vi "myRIO_BRig_RT_v0,80__PortC.vi"() -> ()   [LabVIEW 2014]
uses:
  myRIO_BRig_RT__Case_Exp_stateList.ctl
  myRIO_BRig_RT__Case_NonExp_stateList.ctl
  <vilib>/Platform/TimedLoop/XDataNode/timing_clust.ctl
  <vilib>/Platform/TimedLoop/XDataNode/nitl_modes.ctl
  <vilib>/Platform/TimedLoop/XDataNode/wakeup.ctl
  <vilib>/WebDAVClient/Advanced/SessionHandle.ctl
  <vilib>/myRIO/Common/Instrument Driver Framework/myRIO v1.0/UART/vis/myRIO v1.0 Close UART.vi
  <vilib>/FPGAPlugInAG/myRIO-1900/niLvFpga_Open_myRIO-1900.vi
  <vilib>/rvi/interface/common/dynamic/niFpgaDynamicAddResources.vi
  <vilib>/Utility/error.llb/Error Cluster From Error Code.vi
  <vilib>/rvi/errors/niLvFpgaAdjustHostInterfaceError.vi
  <vilib>/FPGAPlugInAG/Dynamic/niLvFpga_Close_Dynamic.vi
  <vilib>/myRIO/Common/Instrument Driver Framework/Utilities/vis/FPGA Ref Manager.vi
  <vilib>/myRIO/Common/Instrument Driver Framework/myRIO v1.0/myRIO v1.0 Reset FPGA.vi
  <vilib>/myRIO/Common/Instrument Driver Framework/myRIO v1.0/IRQ/vis/myRIO v1.0 IRQ Info FGV.vi
  <vilib>/myRIO/Common/Instrument Driver Framework/myRIO v1.0/IRQ/vis/myRIO v1.0 Timer IRQ Info FGV.vi
  <vilib>/myRIO/Common/Instrument Driver Framework/myRIO v1.0/IRQ/vis/myRIO v1.0 ISR Agent.vi
  <vilib>/rvi/interface/nirviOpenFPGA/nirviOpenFPGA.xnode
  myRIO_BRig_FPGA_v3,71__PortC__build.lvbitx
  myRIO_BRig_FPGA_v3,71__PortC.vi
  <vilib>/rvi/interface/nirviReadWriteControl/nirviReadWriteControl.xnode
  <vilib>/Platform/TimedLoop/XDataNode/XDataNode.xnode
  <vilib>/rvi/interface/nirviCloseFPGA/nirviCloseFPGA.xnode
  <vilib>/Platform/TimedLoop/XDataNode/XDNodeRunTimeDep.lvlib
  <vilib>/rvi/interface/Simulation/niFpgaSimulationCallBeginRW.vi
  <vilib>/myRIO/Instrument Drivers/Utilities/Utilities.lvlib
  <vilib>/WebDAVClient/NI_WebDAV.lvlib
  NiFpgaLv.dll
panel:
  in  "Tcycle_Cue_LED_max":u16=1000 caption="Max" min=5 max=5000 step=5
  in  "Tcycle_Cue_LED_min":u16=1000 caption="Min" min=5 max=5000 step=5
  in  "Tcycle_CuePenalty_LED":u16=1000 caption="Penalty" min=1 max=10000 step=1
  out "power_l2":dbl
  out "error out 6":errorcluster
  in  "MTrig_Laser_Switch":bool
  in  "Cue1Param_AudioLed_Count_NS":u16
  in  "Cue1Param_AudioLed_Count_Switch":u16
  in  "Cue1Param_AudioLed_Probability_NS":u16
  in  "Cue1Param_CueType_NS":u16(slide) max=2 step=1 scale=0.0..2.0
  in  "Cue1Param_AudioLed_Probability_Switch":u16
  in  "Cue1Param_CueType_Switch":u16(slide) max=2 step=1 scale=0.0..2.0
  in  "CueLed_Freq":dbl=10.0
  in  "CueLed_Tpeak":dbl=2.0
  in  "Laser_power_step_l2":dbl
  in  "Laser_power_max_l2":dbl
  in  "Laser_power_min_l2":dbl
  in  "Laser_Tshutter_l2":dbl=2.0
  in  "Laser_Freq_l2":dbl=10.0
  in  "Laser_Tpeak_l2":dbl=2.0
  in  "Laser_duration_l2":u16
  in  "LC_Sel_Count_NS_l2":u16
  in  "LC_Sel_Count_Switch_l2":u16
  in  "LC_Sel_Probability_NS_l2":u16
  in  "LC_Sel_Block_NS_l2":u16(slide) max=2 step=1 scale=0.0..2.0
  in  "LC_Sel_OnOff_NS_l2":bool
  in  "LC_Sel_Probability_Switch_l2":u16
  in  "LC_Sel_Block_Switch_l2":u16(slide) max=2 step=1 scale=0.0..2.0
  in  "LC_Sel_OnOff_Switch_l2":bool
  in  "LC_Sel_Tdelay_NS_l2":u16
  in  "LC_Sel_Tdelay_Switch_l2":u16
  in  "LC_Cue1_Count_NS_l2":u16
  in  "LC_Cue1_Count_Switch_l2":u16
  in  "LC_Cue1_delayOpt_NS_l2":bool
  in  "LC_ENL1_delayOpt_NS_l2":bool
  in  "LC_ENL1_Count_NS_l2":u16
  in  "LC_ENL1_Count_Switch_l2":u16
  in  "LC_Cue1_delayOpt_Switch_l2":bool
  in  "LC_ENL1_delayOpt_Switch_l2":bool
  in  "LC_Cue1_Probability_NS_l2":u16
  in  "LC_Cue1_Block_NS_l2":u16(slide) max=2 step=1 scale=0.0..2.0
  in  "LC_Cue1_OnOff_NS_l2":bool
  in  "LC_Cue1_Probability_Switch_l2":u16
  in  "LC_Cue1_Block_Switch_l2":u16(slide) max=2 step=1 scale=0.0..2.0
  in  "LC_Cue1_OnOff_Switch_l2":bool
  in  "LC_ENL1_Probability_NS_l2":u16 max=100 step=1
  in  "LC_ENL1_Block_NS_l2":u16(slide) max=2 step=1 scale=0.0..2.0
  in  "LC_ENL1_OnOff_NS_l2":bool
  in  "LC_ENL1_Probability_Switch_l2":u16 max=100 step=1
  in  "LC_ENL1_Block_Switch_l2":u16(slide) max=2 step=1 scale=0.0..2.0
  in  "LC_Cue1_Tdelay_NS_l2":u16
  in  "LC_ENL1_Tdelay_NS_l2":u16
  in  "LC_Cue1_Tdelay_Switch_l2":u16
  in  "LC_ENL1_Tdelay_Switch_l2":u16
  in  "LC_ENL1_OnOff_Switch_l2":bool
  in  "LC_Wrong_Probability_l2":u16
  in  "LC_Wrong_Trial_l2":u16(slide) max=2 step=1 scale=0.0..2.0
  in  "LC_Wrong_Block_l2":u16(slide) max=2 step=1 scale=0.0..2.0
  in  "LC_Wrong_OnOff_l2":bool
  in  "LC_Reward_Probability_l2":u16
  in  "LC_Reward_Trial_l2":u16(slide) max=2 step=1 scale=0.0..2.0
  in  "LC_Reward_Block_l2":u16(slide) max=2 step=1 scale=0.0..2.0
  in  "LC_Reward_OnOff_l2":bool
  in  "LC_Wrong_Tdelay_l2":u16
  in  "LC_Reward_Tdelay_l2":u16
  in  "LC_Sel_Count_NS_l1":u16
  in  "LC_Sel_Count_Switch_l1":u16
  in  "LC_Sel_Probability_NS_l1":u16
  in  "LC_Sel_Block_NS_l1":u16(slide) max=2 step=1 scale=0.0..2.0
  in  "LC_Sel_OnOff_NS_l1":bool
  in  "LC_Sel_Probability_Switch_l1":u16
  in  "LC_Sel_Block_Switch_l1":u16(slide) max=2 step=1 scale=0.0..2.0
  in  "LC_Sel_OnOff_Switch_l1":bool
  in  "LC_Sel_Tdelay_NS_l1":u16
  in  "LC_Sel_Tdelay_Switch_l1":u16
  out "I_connect_TCP":bool
  out "error out 5":errorcluster
  in  "get_countPerMS":bool
  in  "count_warmup_R_reset":bool
  in  "count_warmup_L_reset":bool
  out "count_warmup_R":u16
  out "count_warmup_L":u16
  out "SolenoidReward":bool
  in  "SolenoidProbability_L":u16=100 caption="Reward Time [ms]" min=1 max=1000 step=1
  in  "SolenoidProbability_R":u16=100 caption="Reward Time [ms]" min=1 max=1000 step=1
  out "power_l1":dbl caption="LaserPower"
  out "error out 4":errorcluster
  in  "Laser_power_step_l1":dbl
  in  "Laser_power_max_l1":dbl
  in  "Recording":bool
  out "error out 3":errorcluster
  out "error out 2":errorcluster
  in  "Laser_power_min_l1":dbl
  in  "FPGA_count2ms":dbl=159.0
  in  "Laser_Tshutter_l1":dbl=2.0
  in  "Laser_Freq_l1":dbl=10.0
  in  "Laser_Tpeak_l1":dbl=2.0
  in  "Laser_duration_l1":u16
  out "error out":errorcluster
  in  "LC_Cue1_Count_NS_l1":u16
  in  "LC_Cue1_Count_Switch_l1":u16
  in  "LC_Cue1_delayOpt_NS_l1":bool
  in  "LC_ENL1_delayOpt_NS_l1":bool
  in  "LC_ENL1_Count_NS_l1":u16
  in  "LC_ENL1_Count_Switch_l1":u16
  in  "LC_Cue1_delayOpt_Switch_l1":bool
  in  "LC_ENL1_delayOpt_Switch_l1":bool
  in  "Tcycle_Cue_Audio_max":u16=1000 caption="Max" min=5 max=5000 step=5
  in  "Tcycle_Cue_Audio_min":u16=1000 caption="Min" min=5 max=5000 step=5
  in  "SendData":bool
  out "cSpout":enum16{"Left", "Right"}(ring) caption="Left or Right Spout"
  out "A4":u32 caption="LickCounter_Right"
  out "A2":u32 caption="LickCounter_Left"
  in  "LR_wrong_Event":bool
  out "error_initTrial":errorcluster
  out "error_Selection_pre":errorcluster
  out "error_Selection":errorcluster
  out "SelectWrong":bool
  out "SelectReward":bool
  in  "Left(F)_or_Right(T)":bool
  in  "ignoreWrong":bool
  in  "SelectionState":bool
  in  "LR_wrong_Laser":bool
  in  "LR_reward_Laser":bool
  in  "LR_reward_Event":bool
  out "nRewards_Right":u16 caption="# Rewards Total (Right)"
  out "nRewards_Left":u16 caption="# Rewards Total (Left)"
  out "nRewards_cur":u16 caption="# Rewards in Current Block"
  out "TpB_target":u16 caption="Target Trials Per Block"
  out "cState_NonExp":T1 caption="WarmUp State"
  out "iBlock":u16 caption="Current Block"
  out "cState":T2 caption="Experimental State"
  out "iTrial":u16 caption="Current Trial"
  in  "warmupType":u8(slide) max=2 step=1 scale=0.0..2.0
  in  "TestConnection":bool
  in  "warmup":bool caption="WarmUp"
  in  "Data Set Prefix":string="Exp1_TM2"
  out "Connected To Host?":bool
  in  "Host Password":string="sabalab"
  in  "Host UserName":string="Test2"
  in  "sp_RightSpout":u16(slide)=2 max=2 step=1 scale=0.0..2.0
  in  "sp_LeftSpout":u16(slide)=2 max=2 step=1 scale=0.0..2.0
  in  "BUR_max":u16 caption="Count Reward Structure  (0 = off)"
  in  "LC_Wrong_Probability_l1":u16
  in  "LC_Wrong_Trial_l1":u16(slide) max=2 step=1 scale=0.0..2.0
  in  "LC_Wrong_Block_l1":u16(slide) max=2 step=1 scale=0.0..2.0
  in  "LC_Wrong_OnOff_l1":bool
  in  "LC_Reward_Probability_l1":u16
  in  "LC_Reward_Trial_l1":u16(slide) max=2 step=1 scale=0.0..2.0
  in  "LC_Reward_Block_l1":u16(slide) max=2 step=1 scale=0.0..2.0
  in  "LC_Reward_OnOff_l1":bool
  in  "LC_Cue1_Probability_NS_l1":u16
  in  "LC_Cue1_Block_NS_l1":u16(slide) max=2 step=1 scale=0.0..2.0
  in  "LC_Cue1_OnOff_NS_l1":bool
  in  "LC_Cue1_Probability_Switch_l1":u16
  in  "LC_Cue1_Block_Switch_l1":u16(slide) max=2 step=1 scale=0.0..2.0
  in  "LC_Cue1_OnOff_Switch_l1":bool
  in  "LC_ENL1_Probability_NS_l1":u16 max=100 step=1
  in  "LC_ENL1_Block_NS_l1":u16(slide) max=2 step=1 scale=0.0..2.0
  in  "LC_ENL1_OnOff_NS_l1":bool
  in  "LC_ENL1_Probability_Switch_l1":u16 max=100 step=1
  in  "LC_ENL1_Block_Switch_l1":u16(slide) max=2 step=1 scale=0.0..2.0
  in  "Tcycle_Timeout":u16=1000 caption="Timeout Time [ms]" min=10 max=10000 step=1
  in  "Tcycle_Wrong":u16=1000 caption="Wrong Time [ms]" min=10 max=10000 step=1
  in  "Tcycle_Selection":u16=1000 caption="Answer Time [ms]" min=1 max=10000 step=1
  in  "Tcycle_RewardPost":u16=1000 caption="Consumption Time [ms]" min=250 max=10000 step=250
  in  "Tcycle_Reward_L":u16=500 caption="Reward Time [ms]" min=1 max=1000 step=1
  in  "Tcycle_Reward_R":u16=500 caption="Reward Time [ms]" min=1 max=1000 step=1
  in  "TpB_Max_R":u16=4 caption="Max TrialsPerBlock" min=1 max=12 step=1
  in  "TpB_Min_R":u16=4 caption="Min TrialsPerBlock" min=1 max=12 step=1
  in  "TpB_Max_L":u16=4 caption="Max TrialsPerBlock" min=1 max=12 step=1
  in  "TpB_Min_L":u16=4 caption="Min TrialsPerBlock" min=1 max=12 step=1
  in  "BUR_min":u16 caption="Count Reward Structure\n(0 = off)"
  in  "TrialUntilReward":bool caption="Ignore Wrong Selection"
  in  "CueCycles":u16=1 caption="Cue Structure" min=1 max=1 step=1
  in  "MTrig_Laser_Tcycle":u16=10 caption="Time [ms]"
  in  "MTrig_Laser_trig":bool
  in  "MTrig_Audio_trig__R":bool caption="Trigger Audio"
  in  "MTrig_Audio_trig__L":bool caption="Trigger Audio"
  in  "RewCalib_Trig_R":bool caption="Calibrate_R"
  in  "RewCalib_Trig_L":bool caption="Calibrate_L"
  in  "MTrig_Solenoid_Tcycle__R":u16=300 caption="Time [ms]"
  in  "MTrig_Solenoid_Tcycle__L":u16=300 caption="Time [ms]"
  in  "MTrig_Solenoid_trig__R":bool caption="Solenoid"
  in  "MTrig_Solenoid_trig__L":bool caption="Solenoid"
  in  "STOP_abort":bool caption="Stop LabView\n(Stops myRio and FPGA)"
  in  "STOP_endBlock":bool caption="Stop Experiment\n@ End of Block"
  in  "STOP_endTrial":bool caption="Stop Experiment\n@ End of Trial"
  in  "START":bool caption="Start Experiment"
  in  "Tcycle_CuePenalty_Audio":u16=1000 caption="Penalty" min=1 max=10000 step=1
  in  "Audio_Amp__R":u16=100 caption="Amp"
  in  "Audio_Freq__R":u8=5 caption="Freq [kHz]" max=14 step=1
  in  "Audio_Amp__L":u16=100 caption="Amp"
  in  "Audio_Freq__L":u8=5 caption="Freq [kHz]" max=14 step=1
  in  "LC_Wrong_Tdelay_l1":u16
  in  "LC_Cue1_Tdelay_NS_l1":u16
  in  "LC_ENL1_Tdelay_NS_l1":u16
  in  "LC_Reward_Tdelay_l1":u16
  in  "LC_Cue1_Tdelay_Switch_l1":u16
  in  "LC_ENL1_Tdelay_Switch_l1":u16
  in  "LC_ENL1_OnOff_Switch_l1":bool
  in  "Tcycle_ENLPenalty":u16=100 caption="Penalty" min=10 max=10000 step=10
  in  "Tcycle_ENL_max":u16=1000 caption="Max" min=250 max=10000 step=250
  in  "Tcycle_ENL_min":u16=1000 caption="Min" min=250 max=10000 step=250
  # "Communication (Host PC)"
  # "Recording Rig"
  # "Experimental Run"
  # "Current State"
  # "STOP experiment at"
  # "Global Parameters                                                         Trial Parameters"
  # "Left/Right        Give Reward?        Laser Power [V]"
  # "Laser1      Laser2"
  # "FPGA Count per [ms]"
  # "Experiment Task Structure"
  # "Block                   Trial            Target Trials       # Rewards \n                                                            Per Block             Current"
  # "Min            Max            Penalty"
  # "(1) = Switching\n(2) = Two Choice"
  # "WarmUp State"
  # "Lick Counter"
  # "Enforced\nNonLick"
  # "WarmUp"
  # "Left           Right"
  # "Cue then reward (no lick)\n \nLeft                    Right"
  # "# Rewards Total\n                                                                  Left                    Right"
  # "Cue Audio"
  # "Experimental State"
  # "Cue LED"
  # "Selection\n \n\n \nReward\n    Dispense\n    Time\n \n    Dispense\n    Probability\n \n\n    Consumption\n    Time\n\nWrong Choice\n \n \nTimeout Penalty"
  # "Left                  Right"
  # "Manual Control"
  # "Min"
  # "Max"
  # "Solenoid\n \nLeft              Right"
  # "Speaker\n \nLeft                    Right"
  # "Laser 1  |  Laser 2"
  # "Trial Per Block Structure \n               Left                        Right"
  # "Time\n[ms]"
  # "Time\n[ms]"
  # "Time = Cue Min"
  # "Min"
  # "Power = Min"
  # "Max"
  # "Cue1 Control\n                                  Cue Type           LED Probability [%]      Count"
  # "Laser1 Control\n                               On/Off      Block        Probability [%]   Delay [ms]                              Count"
  # "Laser2 Control\n                               On/Off      Block        Probability [%]   Delay [ms]                              Count"
  # "Audio or LED"
  # "Cue 1"
  # "Enforced\nNonLick\n      1"
  # "Enforced\nNonLick\n      1"
  # "from end"
  # "from end"
  # "Switch\nTrial"
  # "Switch\nTrial"
  # "Switch\nTrial"
  # "from start"
  # "from start"
  # "from end"
  # "from end"
  # "NonSwitch\nTrials"
  # "NonSwitch\nTrials"
  # "NonSwitch\nTrials"
  # "from start"
  # "from start"
  # "Cue 1"
  # "Cue 1"
  # "from end"
  # "from end"
  # "Switch\nTrial"
  # "Switch\nTrial"
  # "Cue Audio Parameters"
  # "Cue LED Parameters"
  # "from start"
  # "from start"
  # "Left                  Right"
  # "Frequency\n[Hz]"
  # "Frequency\n[kHz]"
  # "from end"
  # "from end"
  # "NonSwitch\nTrials"
  # "NonSwitch\nTrials"
  # "Timing [ms]\n                    Peak Width"
  # "from start"
  # "from start"
  # "Amp\n(0 - 32,000)"
  # "Selection"
  # "Selection"
  # "from start"
  # "from start"
  # "Switch\nTrial"
  # "Switch\nTrial"
  # "Speaker\nPattern\nDuring Cue"
  # "from start"
  # "from start"
  # "NonSwitch\nTrials"
  # "NonSwitch\nTrials"
  # "Laser1 Parameters"
  # "Laser2 Parameters"
  # "Laser1 Response\n                               On/Off      Block       Trial       Probability [%]   Delay [ms]"
  # "Laser2 Response\n                               On/Off      Block       Trial       Probability [%]   Delay [ms]"
  # "Frequency\n[Hz]"
  # "Frequency\n[Hz]"
  # "Timing [ms]\n Duration     Peak Width   Shutter"
  # "Timing [ms]\n Duration     Peak Width   Shutter"
  # "Selection Reward"
  # "Selection Reward"
  # "Laser Power [V]\nMin          Max              Step"
  # "Laser Power [V]\nMin          Max              Step"
  # "Selection Wrong"
  # "Selection Wrong"
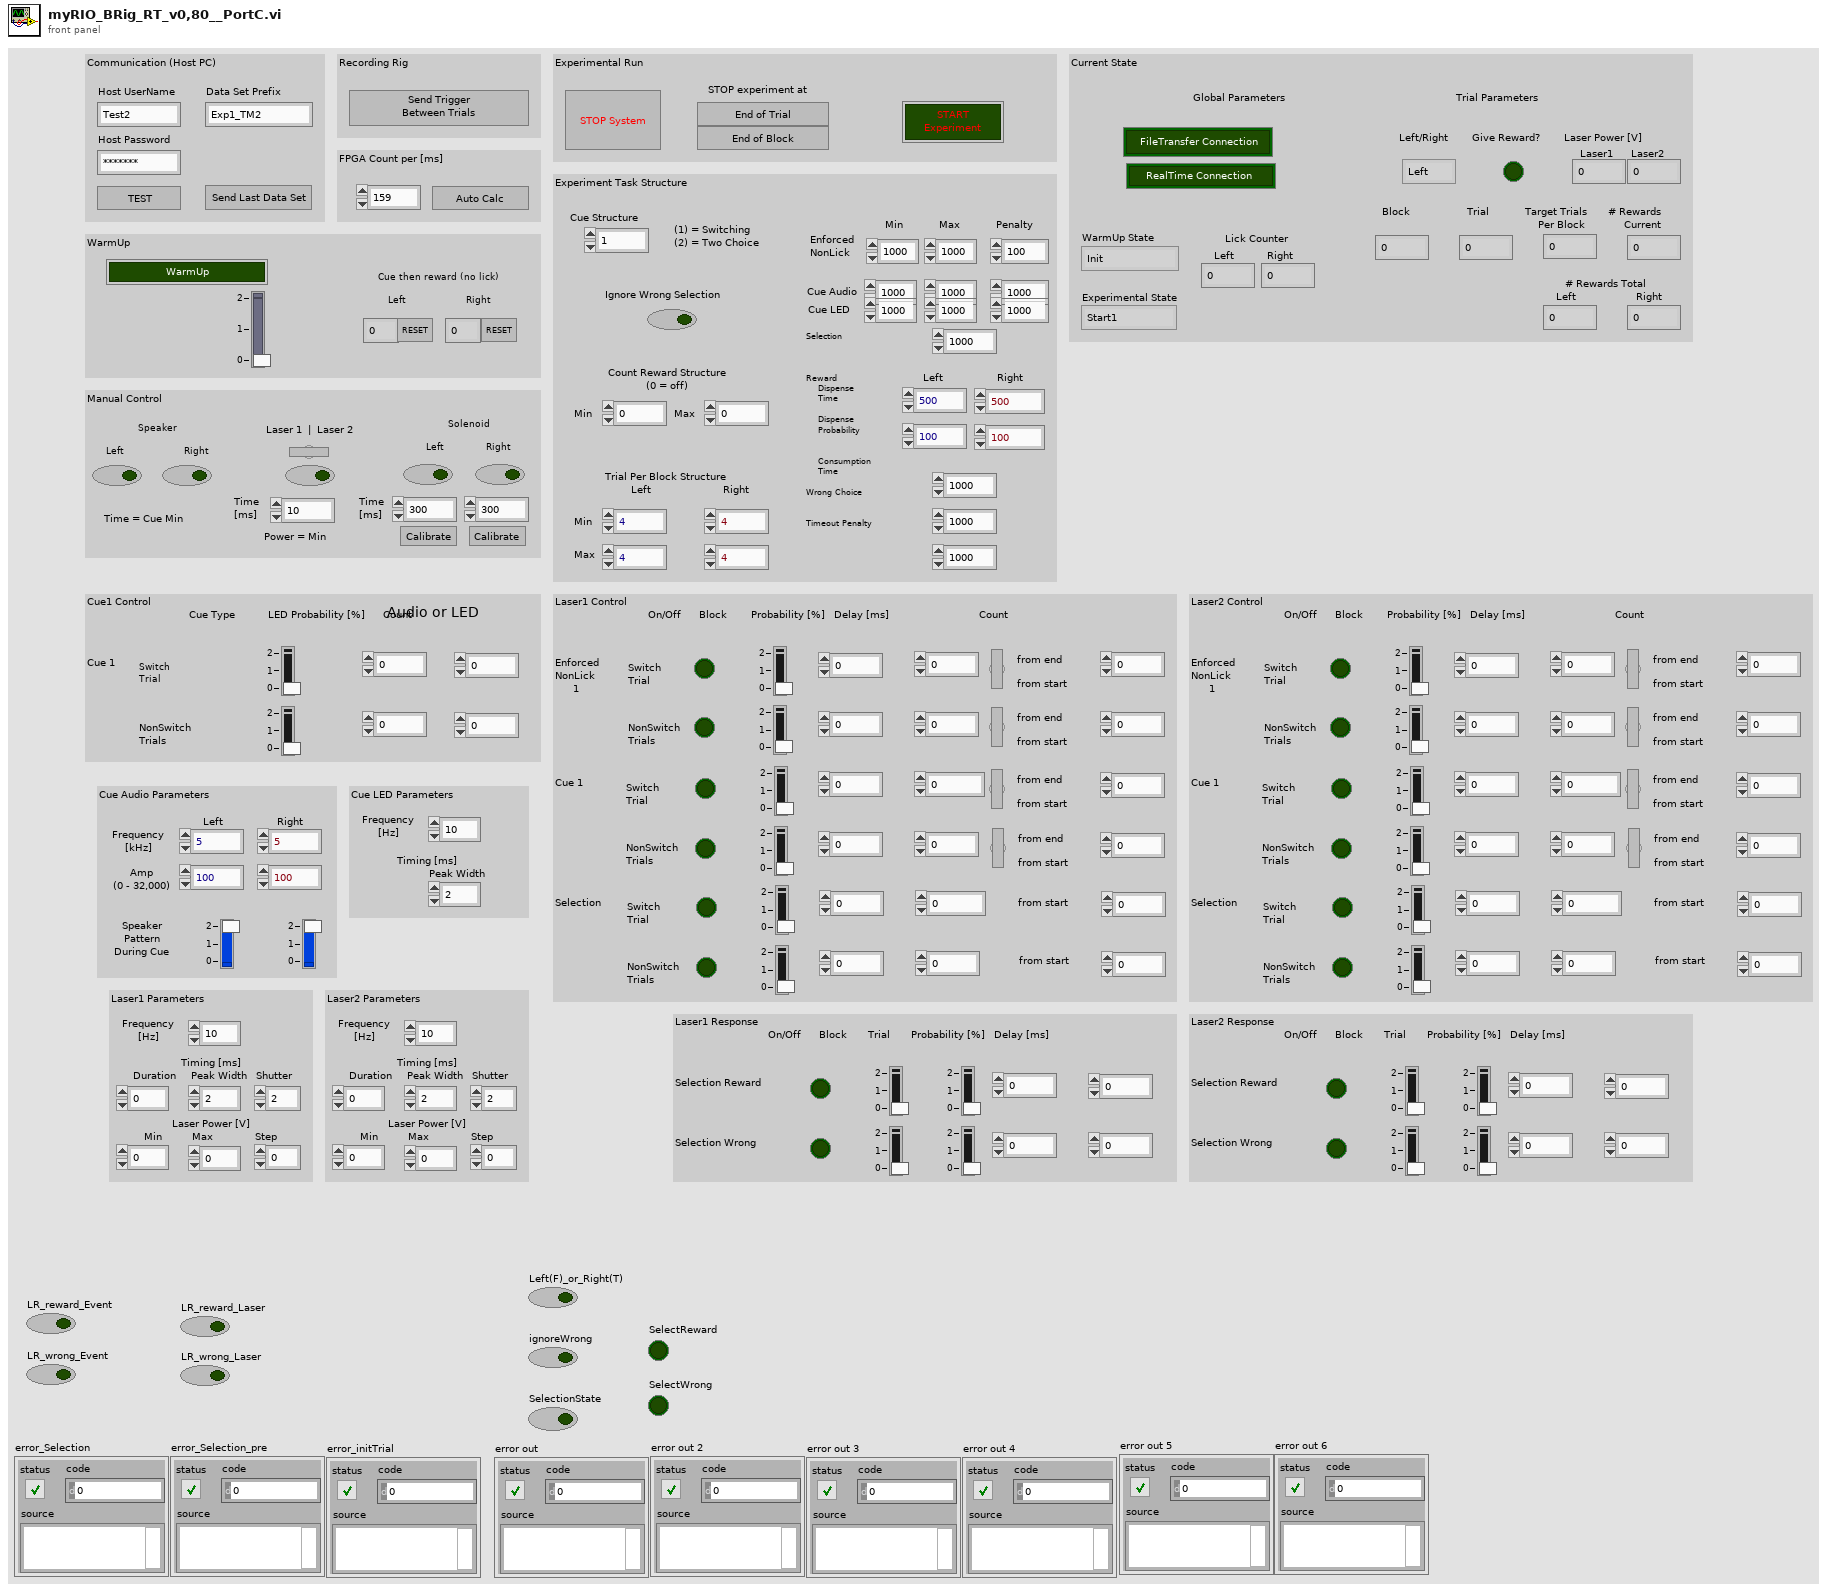
[diagram p1: front panel]
types:
  T1 = typedef "myRIO_BRig_RT__Case_NonExp_stateList.ctl" = enum16{"Init", "UploadSettings_pre", "UploadSettings_Read_dataExp", "UploadSettings_dataExp_1", "UploadSettings_dataExp_2", "UploadSettings_Read_dataLC", "UploadSettings_dataLC_1", "UploadSettings_dataLC_2", "UploadSettings_dataLC_3", "UploadSettings_dataLC_4", "UploadSettings_Read_dataMTrig", "UploadSettings_dataMTrig_1", "UploadSettings_post", "Idle_pre", "IdleEmpty", "IdleEmpty2", "IdleEmpty3", "IdleEmpty4", "Idle", "Idle_2", "Idle_3", "Idle_4", "Idle_5", "Idle_6", "Idle_post", "Cue_pre__pre", "Cue_pre", "Cue", "Cue_LED", "Cue_post", "RewardCalibration_pre", "DispenseWater_pre__pre", "DispenseWater_pre", "DispenseWater", "DispenseWater_post", "TestConnection", "SendData", "Get_FPGA_count_per_ms", "End"}
  T2 = typedef "myRIO_BRig_RT__Case_Exp_stateList.ctl" = enum16{"Start1", "Start2", "Start3", "saveSettings1", "saveSettings2", "saveSettings3", "saveSettings4", "saveSettings_LC_ENL_l1", "saveSettings_LC_ENL_l2", "saveSettings_LC_Cue_l1", "saveSettings_LC_Cue_l2", "saveSettings6_LC_l1_Other", "SaveSettings6_LC_l2_Other", "setSettings_Audio", "setSettings_Laser", "initBlock_pre", "initBlock", "initBlock2", "initBlock_post", "initTrial_pre", "initTrial", "initTrial2", "initTrial3", "initTrial4", "initTrial_LC_ENL1", "initTrial_LC_Cue1", "initTrial_LC_Cue1_2", "initTrial_LC_Sel", "initTrial_post", "ENL1_pre", "ENL1", "ENL1_post", "ENL1Penalty_pre", "ENL1Penalty", "ENL2_pre", "ENL2", "ENL2Penalty_pre", "ENL2Penalty", "Cue1_pre", "Cue1", "Cue1_post", "Cue1Penalty_pre", "Cue1Penalty", "Cue2_pre", "Cue2", "Cue2Penalty_pre", "Cue2Penalty", "Selection_pre", "Selection", "Select_post", "SelectReward_pre", "SelectReward", "SelectRewardPost_pre", "SelectRewardPost", "SelectWrong_pre", "SelectWrong", "SelectWrong_post", "SelectTimeout_pre", "SelectTimeout", "SelectTimeout_post", "endTrial_pre", "endTrial1", "endTrial2", "endTrial3", "endTrial_post", "endBlock_pre", "endBlock", "endBlock_post", "endExp", "commConnect", "commUpload_pre", "commUpload_dataBlock", "commUpload_dataCurrent", "commUpload_dataExp", "commUpload_dataLC", "commUpload_dataTrial", "commUpload_post", "saveData_pre", "saveData_dataBlock", "saveData_dataCurrent", "saveData_dataExp", "saveData_dataLC", "saveData_dataTrial", "saveData_post", "empty_endBlock1", "empty_endBlock2", "empty_endTrial1", "empty_endTrial2", "empty_endTrial3", "empty_endTrial4", "empty_endTrial5", "dummyState", "dummyState_endBlock"}
  T3 = typedef "XDNodeRunTimeDep.lvlib/timing_clust.ctl" = cluster{"Expected End [f-1]":u64, "Actual End [f-1]":u64, "Finished Late? [f-1]":bool, "Expected End [i-1]":u64, "Actual End [i-1]":u64, "Finished Late? [i-1]":bool, "Expected Start [i]":u64, "Actual Start [i]":u64, "Expected Start [f]":u64, "Actual Start [f]":u64, "Source Name":string, "Structure Name":string, "Period":i64, "Deadline":i64, "Offset":i64, "Start":i64, "Priority":i32, "Timeout":i32, "Mode":T4, "Wakeup Reason":T5, "Error":errorcluster, "Source Type":string, "Secondary Source Type":string, "Global End Time":u64, "Global Start Time":u64, "Frame Duration":u64, "Iteration Duration":u64, "Assigned CPU":i32, "I/O Scan Engine Mode":u32}
  T4 = typedef "XDNodeRunTimeDep.lvlib/nitl_modes.ctl" = enum32{"No Change", "Process missed periods, maintain original phase", "Discard missed periods, maintain original phase", "Process missed periods, ignore original phase", "Discard missed periods, ignore original phase"}
  T5 = typedef "XDNodeRunTimeDep.lvlib/wakeup.ctl" = enum32{"Normal", "Aborted", "Asynchronous wakeup", "Timing source error", "Timed loop error", "Timeout"}
  T6 = typedef "NI_WebDAV.lvlib/SessionHandle.ctl" = refnum<k1>
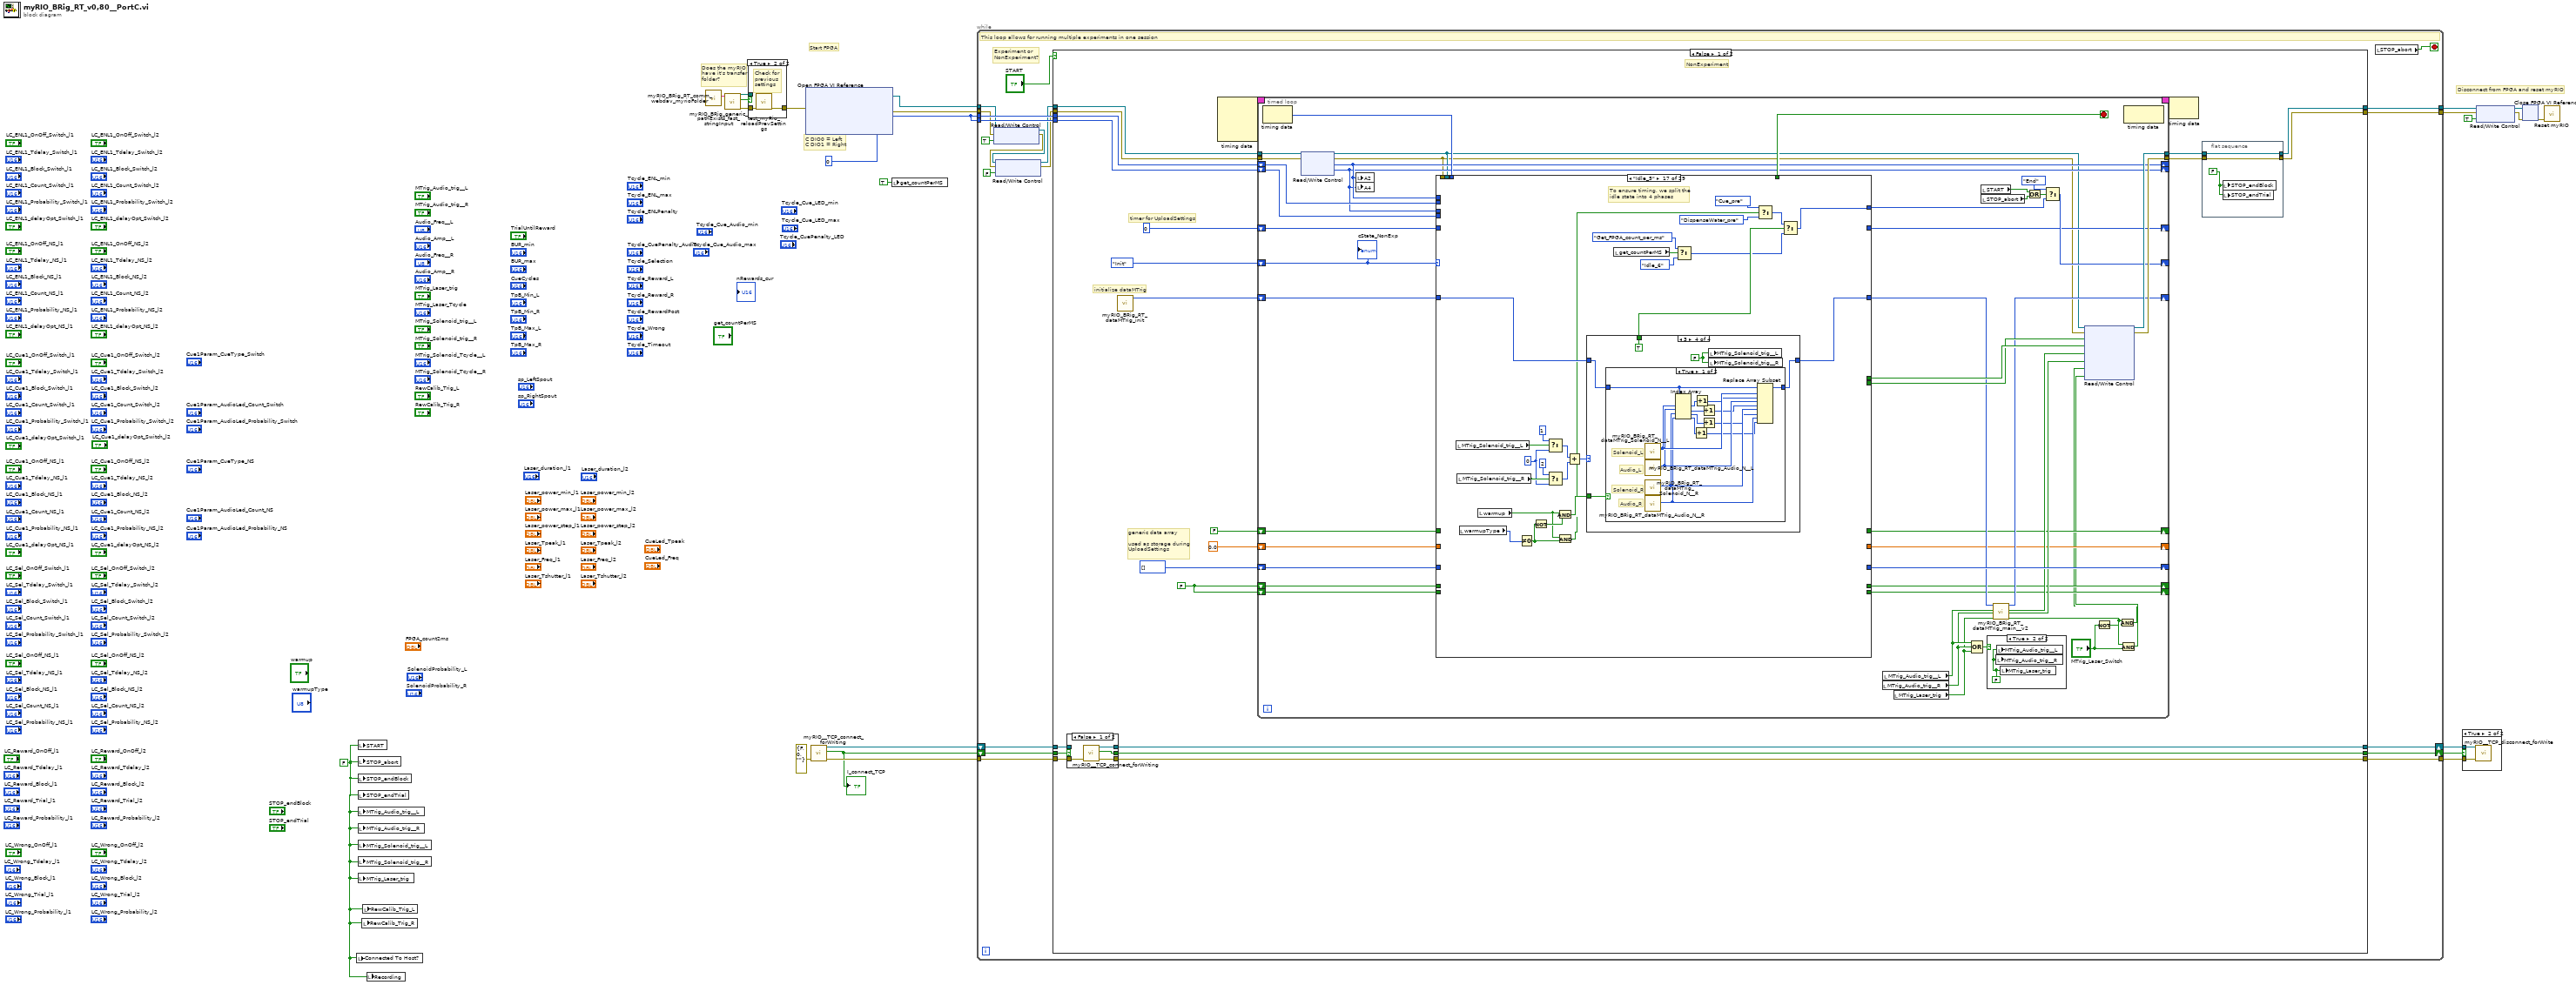
[diagram p0: block diagram]
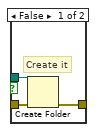
[diagram p3: hidden frame]
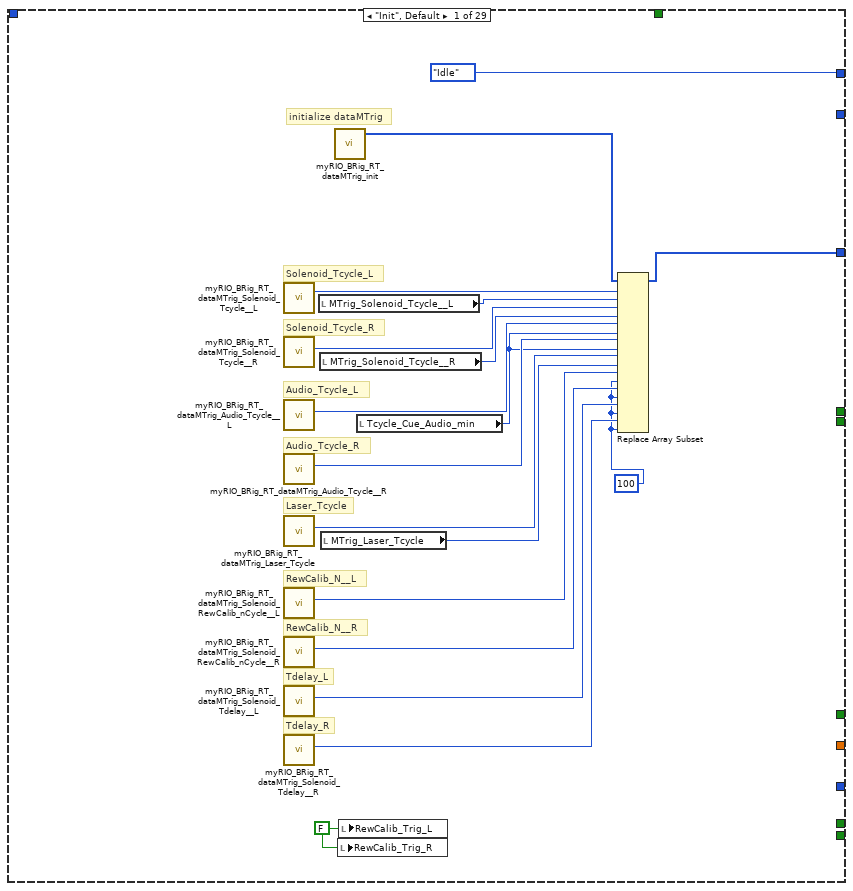
[diagram p6: hidden frame]
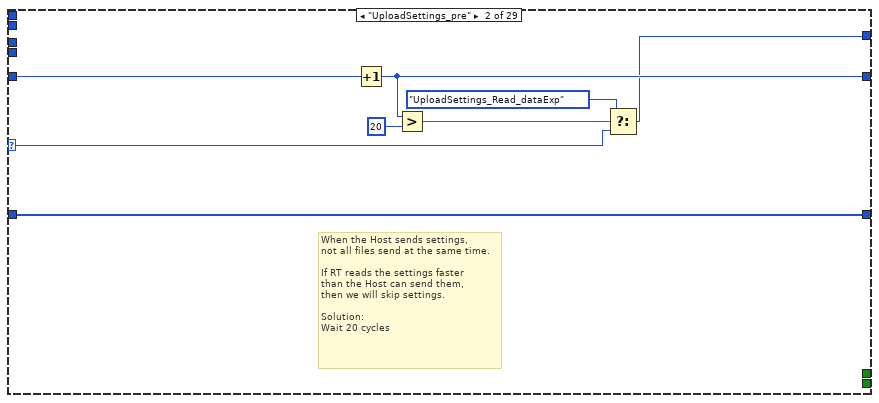
[diagram p7: hidden frame]
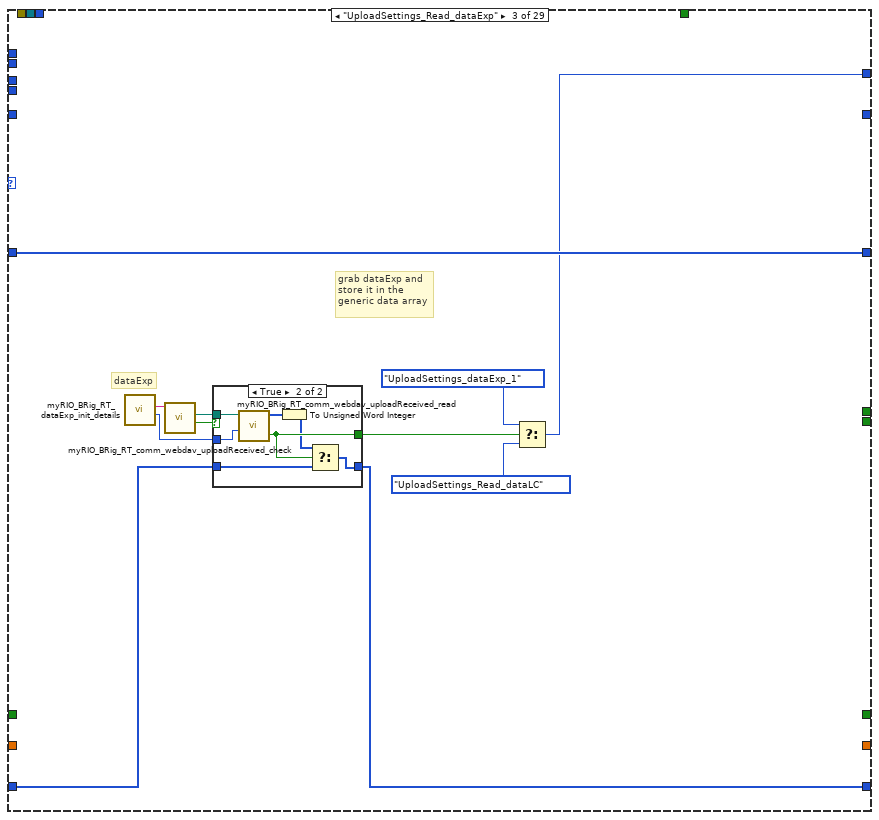
[diagram p8: hidden frame]
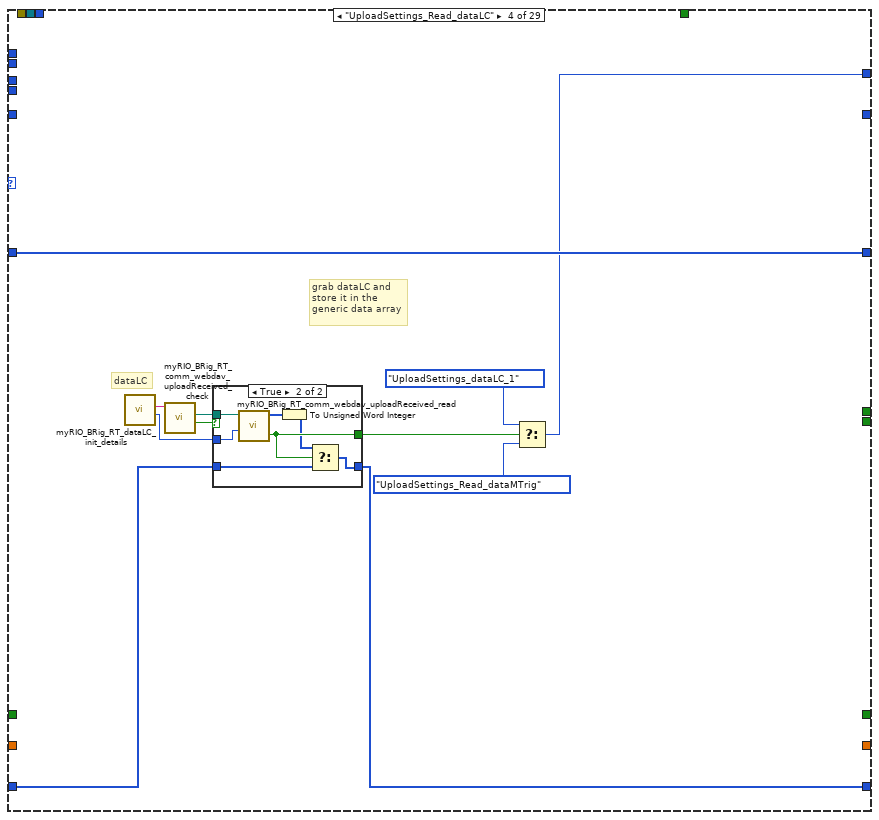
[diagram p10: hidden frame]
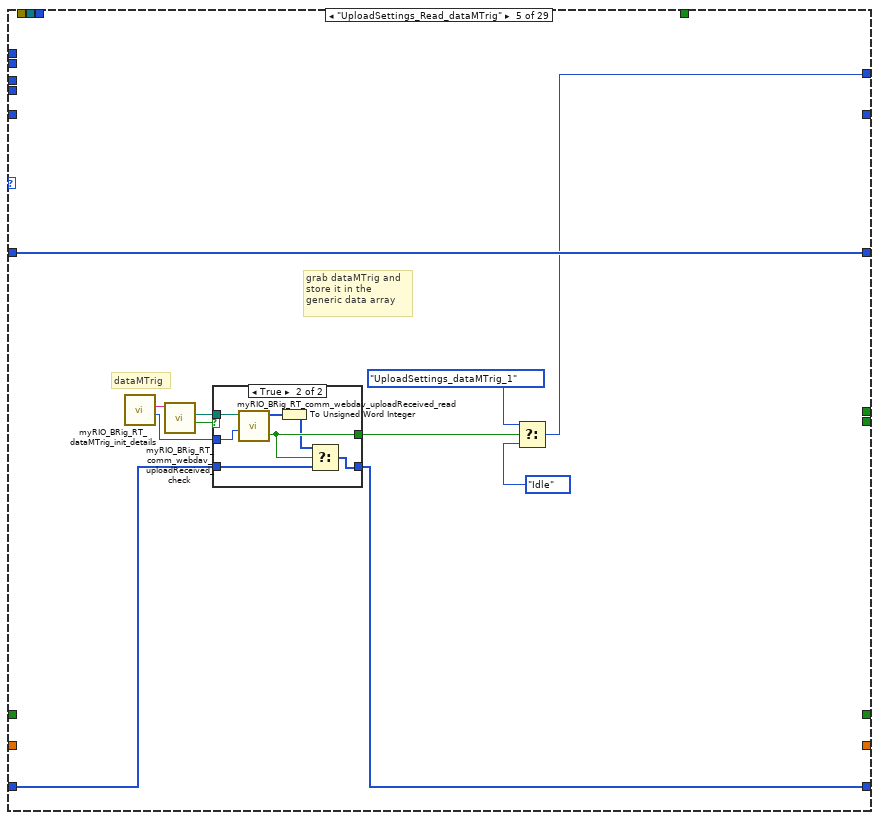
[diagram p12: hidden frame]
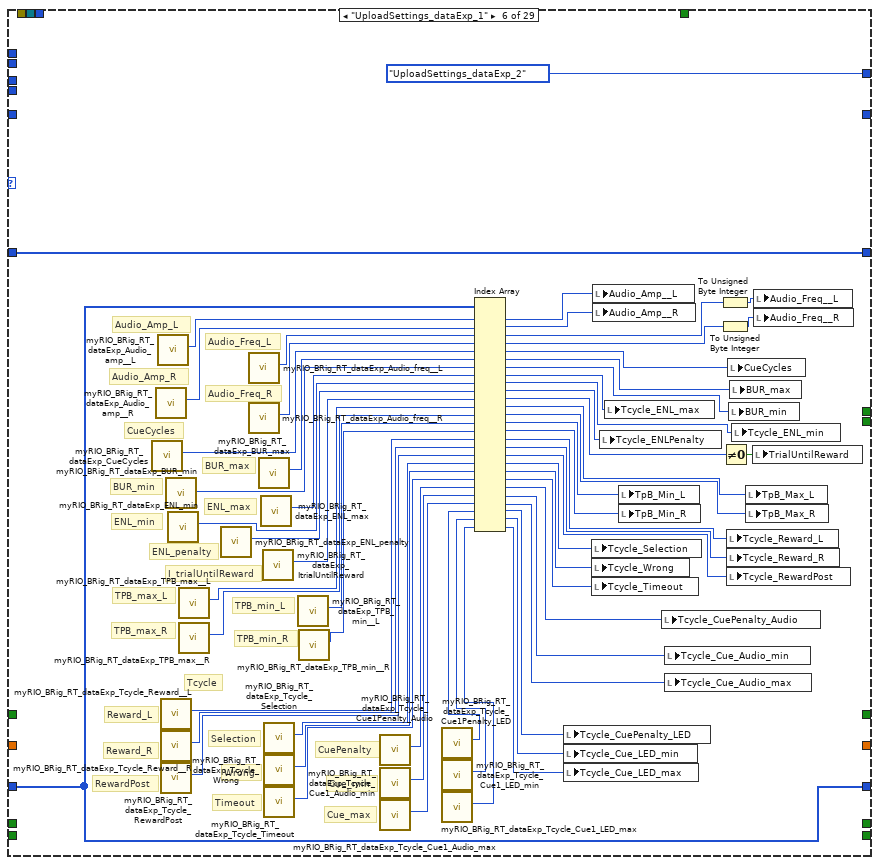
[diagram p14: hidden frame]
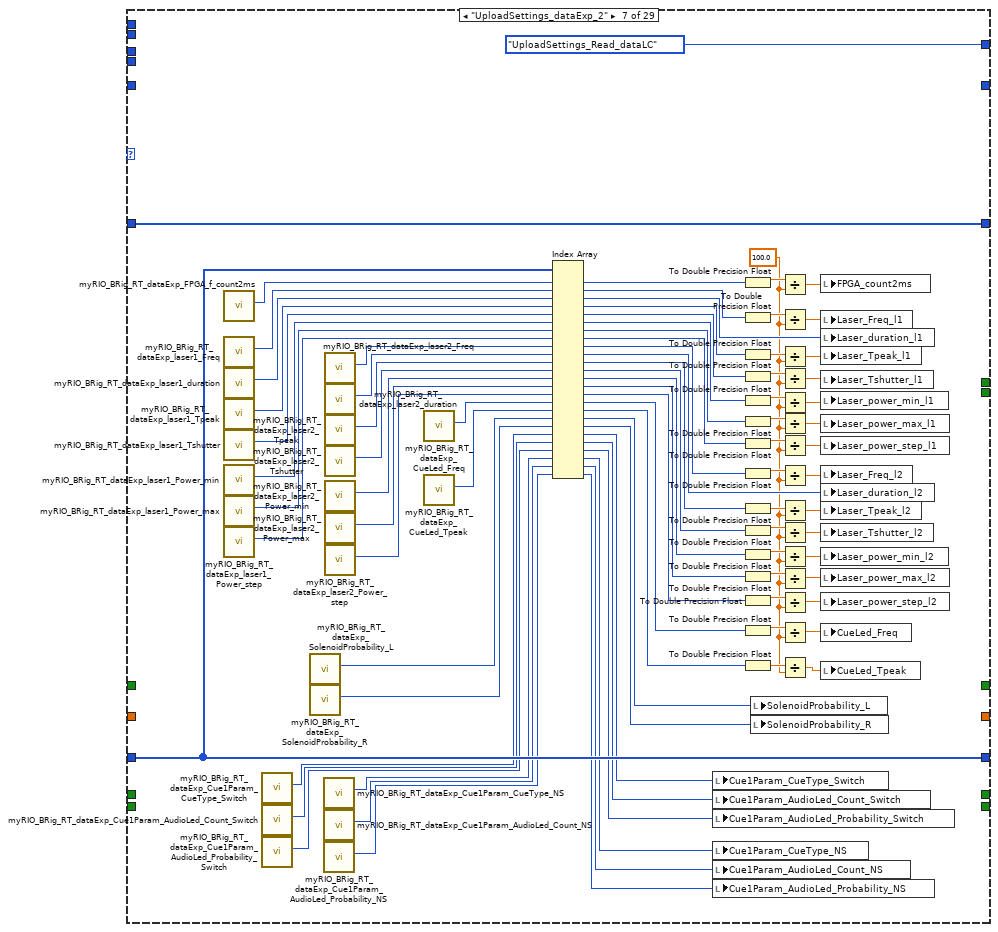
[diagram p15: hidden frame]
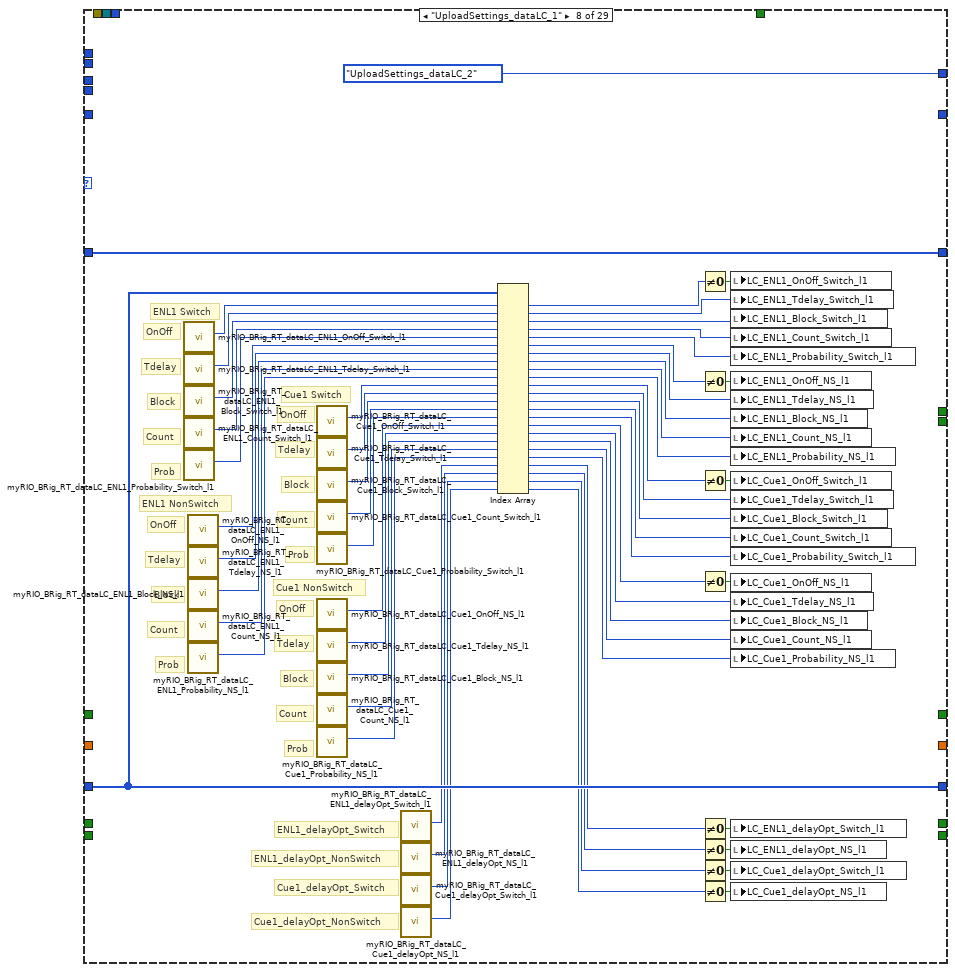
[diagram p16: hidden frame]
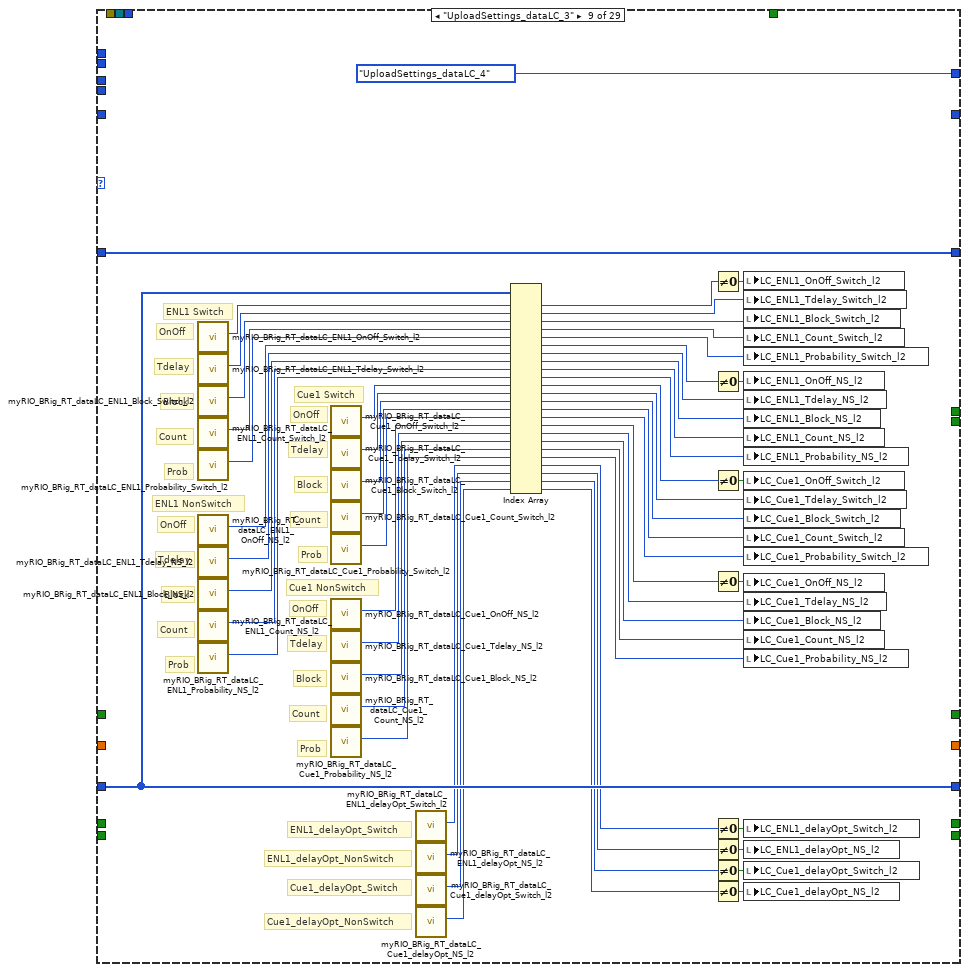
[diagram p17: hidden frame]
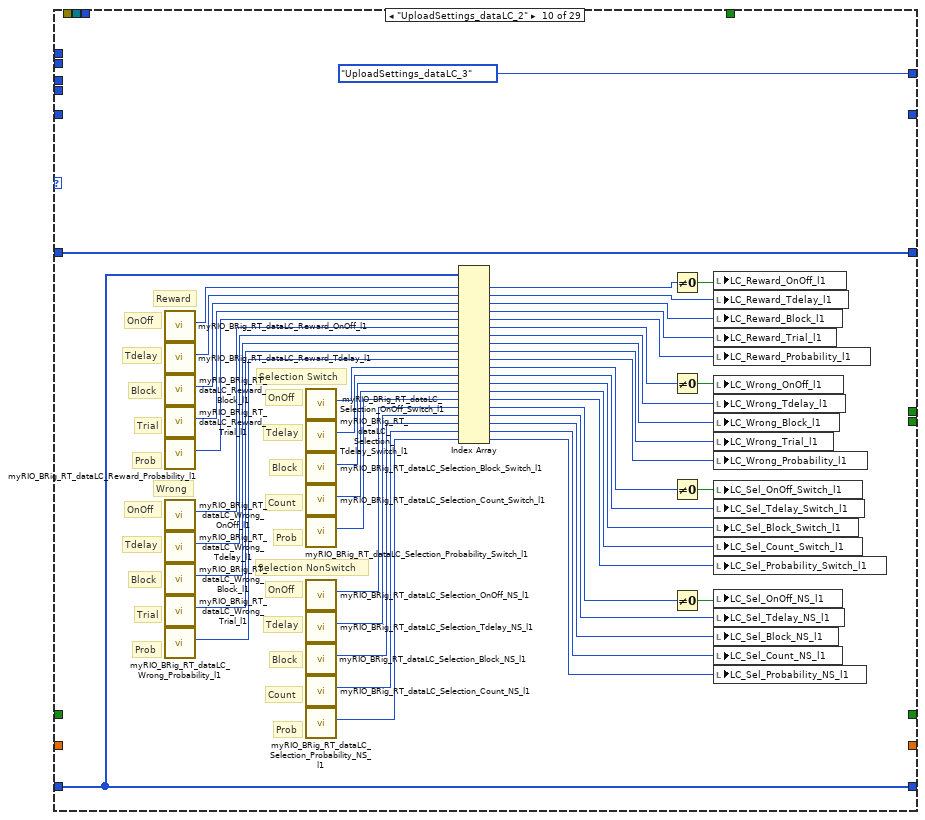
[diagram p18: hidden frame]
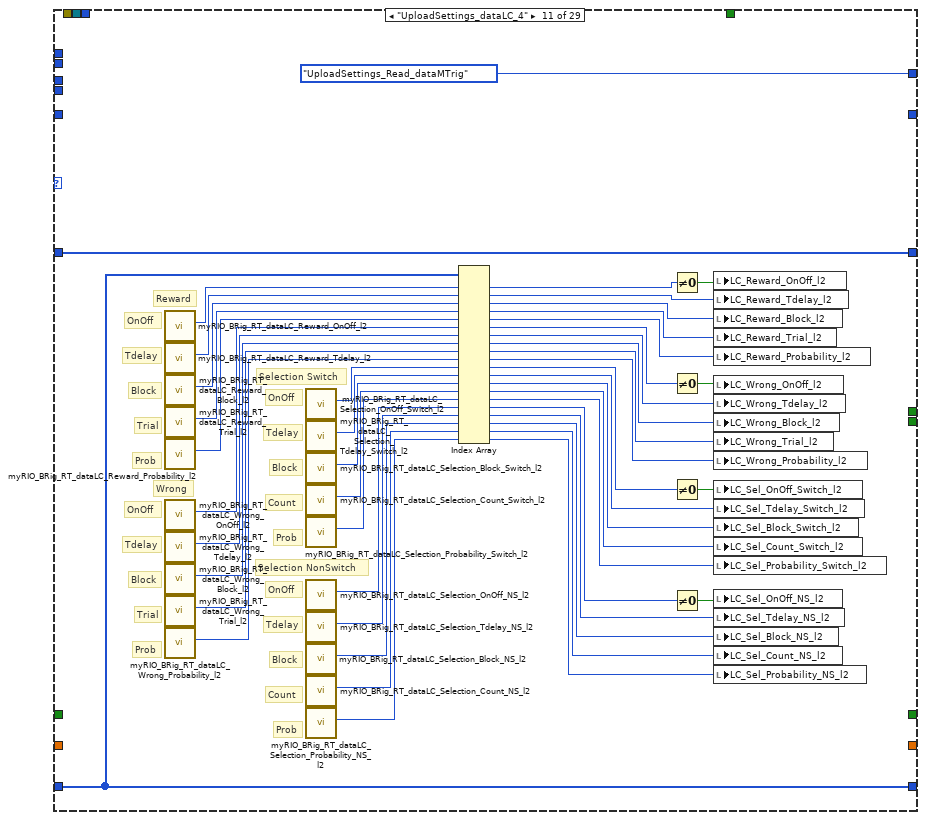
[diagram p19: hidden frame]
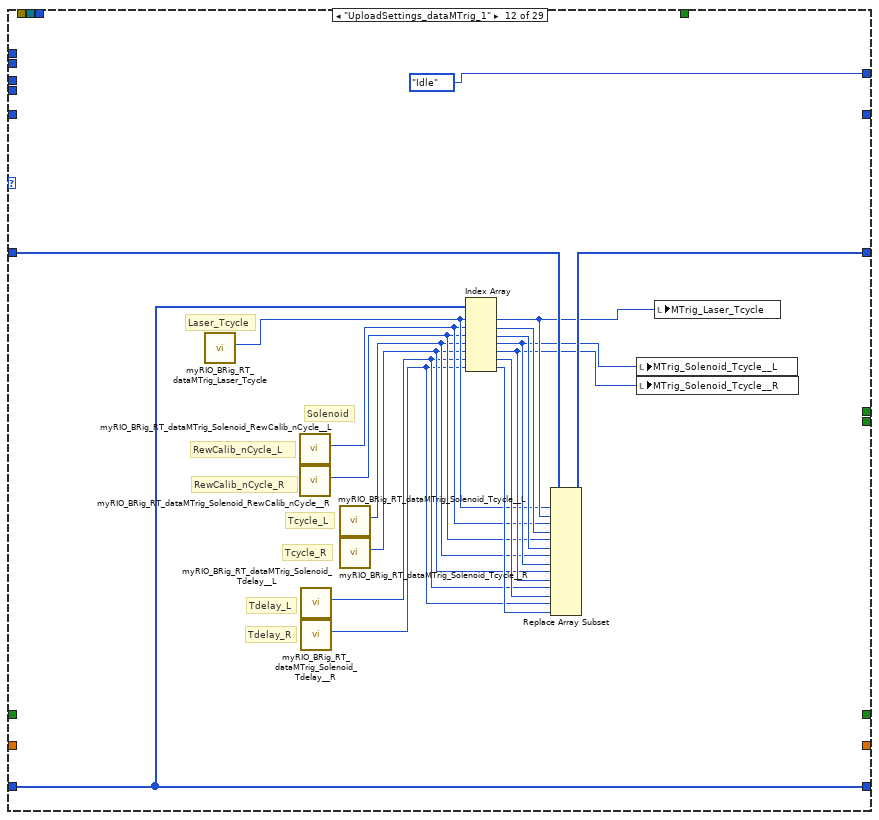
[diagram p20: hidden frame]
diagram:
  w17 = u32 0
  w1 = FALSE
  # "Does the myRIO\nhave it's transfer\nfolder?"
  # "C DIO0 = Left\nC DIO1 = Right"
  # "Start FPGA"
  # "Disconnect from FPGA and reset myRIO"
  n1 = local write "Connected To Host?"(w1) -> ()
  n2 = local write "START"(w1) -> ()
  n3 = local write "STOP_abort"(w1) -> ()
  n4 = local write "STOP_endBlock"(w1) -> ()
  n5 = local write "STOP_endTrial"(w1) -> ()
  n6 = local write "MTrig_Audio_trig__L"(w1) -> ()
  n7 = local write "MTrig_Audio_trig__R"(w1) -> ()
  n8 = local write "MTrig_Solenoid_trig__L"(w1) -> ()
  n9 = local write "MTrig_Solenoid_trig__R"(w1) -> ()
  n10 = local write "MTrig_Laser_trig"(w1) -> ()
  n11 = local write "RewCalib_Trig_R"(w1) -> ()
  n12 = local write "RewCalib_Trig_L"(w1) -> ()
  n13 = local write "Recording"(w1) -> ()
  n14 = call "myRIO_BRig_RT_comm_webdav_myrioFolder.vi"() -> ("output_myrioFolder"=w14:string)  [unwired: 11 in]
  n15 = call "myRIO_BRig_generic_pathExists_fast_stringInput.vi"("input_filePath"=w14) -> ("output_error"=w13:errorcluster, "output_Iexist"=w12:bool, "output_filePath"=w11:path)  [unwired: 8 in]
  n16 = case shown="True" w12 {
    tunnel: w11 -> [w26 _]
    tunnel: w13 -> [w25 w28]
    tunnel: [w24 w27] -> w9
    frame False {
      # "Create it"
      n17 = Create Folder(path (use dialog)=w26, error in=w25) -> (error out=w24:errorcluster)  [unwired: 1 in, 2 out]
    }
    frame True {
      # "Check for\nprevious\nsettings"
      n18 = call "test_myRio_reloadPrevSettings.vi"("input_error"=w28) -> ("output_error"=w27:errorcluster)  [unwired: 10 in]
    }
  }
  n19 = xnode "Open FPGA VI Reference"("error in"=w9) -> ("FPGA VI Reference Out"=w19:refnum<k20>, "error out"=w18:errorcluster)  [unwired: 1 in]
  n20 = call "myRIO__TCP_connect_forWriting.vi"("input_error"=errorcluster {"status"=FALSE, "code"=0, "source"=""}) -> ("output_error"=w7:errorcluster, "output_connected"=w6:bool, "output_hTCP"=w10:refnum<k5>)  [unwired: 8 in]
  "I_connect_TCP" <- w6
  n21 = local write "get_countPerMS"(TRUE ("get_countPerMS")) -> ()
  n22 = while {
    tunnel: w19 -> [w38]
    tunnel: w18 -> [w43]
    tunnel: w17 -> [w46]
    tunnel: w17 -> [w45]
    tunnel: [w36] -> w16
    tunnel: [w35] -> w15
    shift-right: [w32] -> w5
    shift-left: w6 -> [w33]
    tunnel: w7 -> [w31]
    shift-right: [w30] -> w4
    shift-left: w10 -> [w34]
    tunnel: [w29] -> w3
    stop <- w44 stop-if-true
    # "Experiment or\nNonExperiment?"
    # "This loop allows for running multiple experiments in one session"
    n23 = xnode "Read/Write Control"("FPGA VI Reference In"=w38, "error in"=w43, "Counts_Reset"=TRUE) -> ("FPGA VI Reference Out"=w40:refnum<k20>, "error out"=w41:errorcluster)
    n24 = xnode "Read/Write Control"("FPGA VI Reference In"=w40, "error in"=w41, "Counts_Reset"=FALSE) -> ("FPGA VI Reference Out"=w37:refnum<k20>, "error out"=w39:errorcluster)
    n25 = case shown="False" "START" {
      tunnel: w46 -> [w67 w1331]
      tunnel: w45 -> [w66 w1330]
      tunnel: w39 -> [w64 w1262]
      tunnel: w37 -> [w65 w1263]
      tunnel: [w62 w1327] -> w36
      tunnel: [w60 w1322] -> w35
      tunnel: w34 -> [w53 w1273]
      tunnel: [w51 w1277] -> w30
      tunnel: w33 -> [w52 w1275]
      tunnel: [w50 w1276] -> w32
      tunnel: w31 -> [w54 w1274]
      tunnel: [w49 w1272] -> w29
      frame False {
        w57 = FALSE
        # "generic data array\n\nused as storage during\nUploadSettings"
        # "timer for UploadSettings"
        # "initialize dataMTrig"
        # "NonExperiment"
        n26 = case shown="False" w52 {
          selector: w52 -> [_ w76]
          tunnel: w54 -> [w73 w78]
          tunnel: [w74 w78] -> w49
          tunnel: w53 -> [_ w77]
          tunnel: [w75 w77] -> w51
          tunnel: [w72 w76] -> w50
          frame False {
            n27 = call "myRIO__TCP_connect_forWriting.vi"("input_error"=w73) -> ("output_error"=w74:errorcluster, "output_connected"=w72:bool, "output_hTCP"=w75:refnum<k5>)  [unwired: 8 in]
          }
          frame True {
          }
        }
        n28 = call "myRIO_BRig_RT_dataMTrig_init.vi"() -> ("output_dataMTrig"=w68:u16[])  [unwired: 5 in]
        n29 = node-c288() -> (w71:T3)  [unwired: 4 in]
        n30 = timed-loop {
          timing: w71 -> [_]
          timing-out: [_] -> w70
          shift-right: [w115] -> _
          shift-left: w68 -> [w127]
          shift-right: [w109] -> _
          shift-left: myRIO_BRig_RT__Case_NonExp_stateList."Init" ("Enum") -> [w121]
          shift-right: [w103] -> _
          shift-left: w67 -> [w104]
          shift-right: [w101] -> _
          shift-left: w66 -> [w102]
          tunnel: [w123] -> w63
          tunnel: [w122] -> w61
          tunnel: w64 -> [w125]
          tunnel: w65 -> [w124]
          shift-right: [w120] -> _
          shift-left: u16[] [] ("output_data") -> [w119]
          shift-right: [w105] -> _
          shift-left: u16 0 ("Audio_Amp__L") -> [w106]
          shift-right: [w98] -> _
          shift-left: w57 -> [w100]
          shift-right: [w97] -> _
          shift-left: w57 -> [w99]
          shift-right: [w93] -> _
          shift-left: FALSE -> [w94]
          shift-right: [w91] -> _
          shift-left: 0.0 -> [w92]
          stop <- w128 stop-if-true
          n31 = node-c288() -> (w126:i64)  [unwired: 1 in]
          n32 = xnode "Read/Write Control"("FPGA VI Reference In"=w124, "error in"=w125) -> ("FPGA VI Reference Out"=w96:refnum<k20>, "error out"=w95:errorcluster, "A2_LickL"=w103:u32, "A4_LickR"=w101:u32)
          n33 = local write "A2"(w103) -> ()
          n34 = local write "A4"(w101) -> ()
          n35 = case shown="\"Idle_5\"" w121 {
            selector: w121 -> [_ w151 _ _ _ _ _ _ _ _ _ _ _ _ _ _ _ _ _ w881 w937 _ _ w1142 _ _ _ w1214 w1256]
            tunnel: [myRIO_BRig_RT__Case_NonExp_stateList."Idle" ("Enum") w149 w156 w175 w194 myRIO_BRig_RT__Case_NonExp_stateList."UploadSettings_dataExp_2" ("Enum") myRIO_BRig_RT__Case_NonExp_stateList."UploadSettings_Read_dataLC" ("Enum") myRIO_BRig_RT__Case_NonExp_stateList."UploadSettings_dataLC_2" ("Enum") myRIO_BRig_RT__Case_NonExp_stateList."UploadSettings_dataLC_4" ("Enum") myRIO_BRig_RT__Case_NonExp_stateList."UploadSettings_dataLC_3" ("f") myRIO_BRig_RT__Case_NonExp_stateList."UploadSettings_Read_dataMTrig" ("f") myRIO_BRig_RT__Case_NonExp_stateList."Idle" ("Enum") w604 w619 myRIO_BRig_RT__Case_NonExp_stateList."Idle_4" ("Enum") myRIO_BRig_RT__Case_NonExp_stateList."Idle_5" ("Enum") w715 w823 w847 w876 w932 myRIO_BRig_RT__Case_NonExp_stateList."DispenseWater_pre" ("Enum") w1088 w1140 w1162 myRIO_BRig_RT__Case_NonExp_stateList."Idle" ("Enum") myRIO_BRig_RT__Case_NonExp_stateList."Idle" ("Enum") w1213 w1256] -> w110
            tunnel: [w139 w148 w166 w185 w204 w272 w356 w409 w468 w521 w568 w584 w608 w634 w647 w701 w720 w821 w856 w882 w938 w999 w1125 w1147 w1173 w1207 w1212 w1224 w1254] -> w116
            tunnel: [_ _ _ _ _ _ _ _ _ _ _ _ _ _ _ _ _ _ _ _ _ _ _ _ _ _ _ _ TRUE] -> w128
            tunnel: w127 -> [_ w148 w166 w185 w204 w272 w356 w409 w468 w521 w568 w585 w607 w634 w647 w701 w721 w821 w857 w883 w939 w985 w1121 w1148 w1174 w1207 w1212 w1224 w1254]
            tunnel: w126 -> [_ _ _ _ _ _ _ _ _ _ _ _ _ _ _ _ _ _ _ _ _ _ _ w1152 _ _ _ _ _]
            tunnel: [_ _ w157 w176 w195 w221 w354 w410 w469 w517 w564 w569 _ _ _ _ _ _ w843 _ w926 _ _ _ _ _ _ _ _] -> w120
            tunnel: w119 -> [_ _ w158 w177 w196 w221 w354 w410 w469 w517 w564 w569 _ _ _ _ _ _ _ _ w927 _ _ _ _ _ _ _ _]
            tunnel: [_ _ _ _ _ _ _ _ _ _ _ _ _ _ _ _ _ _ _ _ _ _ _ w1149 _ _ _ _ _] -> w118
            tunnel: [_ _ _ _ _ _ _ _ _ _ _ _ _ _ _ _ _ _ _ _ _ _ _ w1131 _ _ _ _ _] -> w117
            tunnel: w106 -> [_ w155 _ _ _ _ _ _ _ _ _ _ _ _ _ _ _ _ _ _ _ _ _ _ _ _ _ _ _]
            tunnel: [_ w154 _ _ _ _ _ _ _ _ _ _ _ _ _ _ _ _ _ _ _ _ _ _ _ _ _ _ _] -> w105
            tunnel: w104 -> [_ _ _ _ _ _ _ _ _ _ _ _ _ _ _ _ _ _ _ w887 w943 _ _ _ _ _ _ _ _]
            tunnel: w103 -> [_ _ _ _ _ _ _ _ _ _ _ _ _ _ _ _ _ _ _ w888 w944 _ _ _ _ _ _ _ _]
            tunnel: w102 -> [_ _ _ _ _ _ _ _ _ _ _ _ _ _ _ _ _ _ _ w885 w941 _ _ _ _ _ _ _ _]
            tunnel: w101 -> [_ _ _ _ _ _ _ _ _ _ _ _ _ _ _ _ _ _ _ w886 w942 _ _ _ _ _ _ _ _]
            tunnel: w100 -> [_ _ _ _ _ _ _ _ _ _ _ _ _ _ _ _ _ _ _ w873 w929 _ _ _ _ _ _ _ _]
            tunnel: w99 -> [_ _ _ _ _ _ _ _ _ _ _ _ _ _ _ _ _ _ _ w872 w928 _ _ _ _ _ _ _ _]
            tunnel: [_ _ _ _ _ _ _ _ _ _ _ _ _ _ _ _ _ _ w845 w873 w929 _ _ _ _ _ _ _ _] -> w98
            tunnel: [_ _ _ _ _ _ _ _ _ _ _ _ _ _ _ _ _ _ w844 w872 w928 _ _ _ _ _ _ _ _] -> w97
            tunnel: w96 -> [_ _ _ _ _ _ _ _ _ _ _ _ w597 _ w668 w703 _ _ _ _ w925 _ _ _ _ _ _ w1219 _]
            tunnel: w95 -> [_ _ _ _ _ _ _ _ _ _ _ _ w596 _ w667 w702 _ _ _ _ w924 _ _ _ _ _ _ w1218 _]
            tunnel: w94 -> [_ _ _ _ _ _ _ _ _ _ _ _ _ _ _ _ _ _ _ _ _ _ _ _ _ _ _ w1223 _]
            tunnel: [_ _ _ _ _ _ _ _ _ _ _ _ _ _ _ _ _ _ _ _ _ _ _ _ _ _ _ TRUE _] -> w93
            tunnel: w92 -> [_ _ _ _ _ _ _ _ _ _ _ _ _ _ _ _ _ _ _ _ _ _ _ _ _ _ _ w1221 _]
            tunnel: [_ _ _ _ _ _ _ _ _ _ _ _ _ _ _ _ _ _ _ _ _ _ _ _ _ _ _ w1220 _] -> w91
            frame "Init", Default {
              w133 = FALSE ("RewCalib_Trig_L")
              w130 = u16 100 ("new element/subarray")
              # "Tdelay_R"
              # "Tdelay_L"
              # "RewCalib_N__R"
              # "RewCalib_N__L"
              # "Solenoid_Tcycle_R"
              # "Solenoid_Tcycle_L"
              # "Laser_Tcycle"
              # "Audio_Tcycle_R"
              # "Audio_Tcycle_L"
              # "initialize dataMTrig"
              n36 = call "myRIO_BRig_RT_dataMTrig_Solenoid_Tcycle__L.vi"() -> ("output_Solenoid_Tcycle__L"=w141:i32)  [unwired: 11 in]
              n37 = call "myRIO_BRig_RT_dataMTrig_Solenoid_Tcycle__R.vi"() -> ("output_Solenoid_Tcycle__R"=w142:i32)  [unwired: 11 in]
              n38 = call "myRIO_BRig_RT_dataMTrig_Audio_Tcycle__L.vi"() -> ("output_Audio_Tcycle__L"=w143:i32)  [unwired: 11 in]
              n39 = call "myRIO_BRig_RT_dataMTrig_Audio_Tcycle__R.vi"() -> ("output_Audio_Tcycle__R"=w144:i32)  [unwired: 11 in]
              n40 = call "myRIO_BRig_RT_dataMTrig_Laser_Tcycle.vi"() -> ("output_Laser_Tcycle"=w145:i32)  [unwired: 11 in]
              n41 = call "myRIO_BRig_RT_dataMTrig_Solenoid_RewCalib_nCycle__L.vi"() -> ("output_Solenoid_RewCalib_nCycle__L"=w137:i32)  [unwired: 11 in]
              n42 = call "myRIO_BRig_RT_dataMTrig_Solenoid_RewCalib_nCycle__R.vi"() -> ("output_Solenoid_RewCalib_nCycle__R"=w136:i32)  [unwired: 11 in]
              n43 = call "myRIO_BRig_RT_dataMTrig_Solenoid_Tdelay__L.vi"() -> ("output_Solenoid_Tdelay__L"=w135:i32)  [unwired: 11 in]
              n44 = call "myRIO_BRig_RT_dataMTrig_Solenoid_Tdelay__R.vi"() -> ("output_Solenoid_Tdelay__R"=w134:i32)  [unwired: 11 in]
              n45 = local read "MTrig_Solenoid_Tcycle__L"() -> (w146:u16)
              n46 = local read "MTrig_Solenoid_Tcycle__R"() -> (w147:u16)
              n47 = local read "MTrig_Laser_Tcycle"() -> (w131:u16)
              n48 = call "myRIO_BRig_RT_dataMTrig_init.vi"() -> ("output_dataMTrig"=w140:u16[])  [unwired: 5 in]
              n49 = local write "RewCalib_Trig_R"(w133) -> ()
              n50 = local write "RewCalib_Trig_L"(w133) -> ()
              n51 = local read "Tcycle_Cue_Audio_min"() -> (w132:u16)
              n52 = Replace Array Subset(array=w140, new element #1=w146, index #1=w141, new element #2=w147, index #2=w142, new element #3=w132, index #3=w143, new element #4=w132, index #4=w144, new element #5=w131, index #5=w145, new element #6=w130, index #6=w137, new element #7=w130, index #7=w136, new element #8=w130, index #8=w135, new element #9=w130, index #9=w134) -> (w139:u16[])
            }
            frame "UploadSettings_pre" {
              # "When the Host sends settings,\nnot all files send at the same time.\n\nIf RT reads the settings faster\nthan the Host can send them,\nthen we will skip settings.\n\nSolution:\nWait 20 cycles"
              n53 = Increment(x=w155) -> (x+1=w154:u16)
              n54 = Greater?(x=w154, y=u16 20) -> (0:w152:bool)
              n55 = Select(t=myRIO_BRig_RT__Case_NonExp_stateList."UploadSettings_Read_dataExp", s=w152, f=w151) -> (s? t:f=w149:T1)
            }
            frame "UploadSettings_Read_dataExp" {
              # "grab dataExp and\nstore it in the\ngeneric data array"
              # "dataExp"
              n56 = call "myRIO_BRig_RT_dataExp_init_details.vi"() -> ("output_dataSize"=w162:i32, "output_dataName"=w165:string)  [unwired: 10 in]
              n57 = call "myRIO_BRig_RT_comm_webdav_uploadReceived_check.vi"("input_dataName"=w165) -> ("output_Iexist"=w164:bool, "output_dataPath"=w163:path)  [unwired: 9 in]
              n58 = case shown="True" w164 {
                tunnel: w163 -> [_ w174]
                tunnel: w162 -> [_ w173]
                tunnel: [_ w172] -> w161
                tunnel: w158 -> [w167 w171]
                tunnel: [w167 w168] -> w157
                frame False {
                }
                frame True {
                  n59 = call "myRIO_BRig_RT_comm_webdav_uploadReceived_read.vi"("input_dataSize"=w173, "input_filePath"=w174) -> ("output_Ivalid"=w172:bool, "output_data"=w170:i64[])  [unwired: 8 in]
                  n60 = To Unsigned Word Integer(number=w170) -> (unsigned 16bit integer=w169:u16[])
                  n61 = Select(t=w169, s=w172, f=w171) -> (s? t:f=w168:u16[])
                }
              }
              n62 = Select(t=myRIO_BRig_RT__Case_NonExp_stateList."UploadSettings_dataExp_1", s=w161, f=myRIO_BRig_RT__Case_NonExp_stateList."UploadSettings_Read_dataLC" ("t")) -> (s? t:f=w156:T1)
            }
            frame "UploadSettings_Read_dataLC" {
              # "grab dataLC and\nstore it in the\ngeneric data array"
              # "dataLC"
              n63 = call "myRIO_BRig_RT_dataLC_init_details.vi"() -> ("output_dataSize"=w181:i32, "output_dataName"=w184:string)  [unwired: 10 in]
              n64 = call "myRIO_BRig_RT_comm_webdav_uploadReceived_check.vi"("input_dataName"=w184) -> ("output_Iexist"=w183:bool, "output_dataPath"=w182:path)  [unwired: 9 in]
              n65 = case shown="True" w183 {
                tunnel: w182 -> [_ w193]
                tunnel: w181 -> [_ w192]
                tunnel: [_ w191] -> w180
                tunnel: w177 -> [w186 w190]
                tunnel: [w186 w187] -> w176
                frame False {
                }
                frame True {
                  n66 = call "myRIO_BRig_RT_comm_webdav_uploadReceived_read.vi"("input_dataSize"=w192, "input_filePath"=w193) -> ("output_Ivalid"=w191:bool, "output_data"=w189:i64[])  [unwired: 8 in]
                  n67 = To Unsigned Word Integer(number=w189) -> (unsigned 16bit integer=w188:u16[])
                  n68 = Select(t=w188, s=w191, f=w190) -> (s? t:f=w187:u16[])
                }
              }
              n69 = Select(t=myRIO_BRig_RT__Case_NonExp_stateList."UploadSettings_dataLC_1", s=w180, f=myRIO_BRig_RT__Case_NonExp_stateList."UploadSettings_Read_dataMTrig" ("t")) -> (s? t:f=w175:T1)
            }
            frame "UploadSettings_Read_dataMTrig" {
              # "grab dataMTrig and\nstore it in the\ngeneric data array"
              # "dataMTrig"
              n70 = call "myRIO_BRig_RT_dataMTrig_init_details.vi"() -> ("output_dataSize"=w200:i32, "output_dataName"=w203:string)  [unwired: 10 in]
              n71 = call "myRIO_BRig_RT_comm_webdav_uploadReceived_check.vi"("input_dataName"=w203) -> ("output_Iexist"=w202:bool, "output_dataPath"=w201:path)  [unwired: 9 in]
              n72 = case shown="True" w202 {
                tunnel: w201 -> [_ w212]
                tunnel: w200 -> [_ w211]
                tunnel: [_ w210] -> w199
                tunnel: w196 -> [w205 w209]
                tunnel: [w205 w206] -> w195
                frame False {
                }
                frame True {
                  n73 = call "myRIO_BRig_RT_comm_webdav_uploadReceived_read.vi"("input_dataSize"=w211, "input_filePath"=w212) -> ("output_Ivalid"=w210:bool, "output_data"=w208:i64[])  [unwired: 8 in]
                  n74 = To Unsigned Word Integer(number=w208) -> (unsigned 16bit integer=w207:u16[])
                  n75 = Select(t=w207, s=w210, f=w209) -> (s? t:f=w206:u16[])
                }
              }
              n76 = Select(t=myRIO_BRig_RT__Case_NonExp_stateList."UploadSettings_dataMTrig_1", s=w199, f=myRIO_BRig_RT__Case_NonExp_stateList."Idle" ("t")) -> (s? t:f=w194:T1)
            }
            frame "UploadSettings_dataExp_1" {
              # "Cue_max"
              # "Cue_min"
              # "CuePenalty"
              # "Timeout"
              # "Wrong"
              # "Selection"
              # "RewardPost"
              # "Reward_R"
              # "Reward_L"
              # "Tcycle"
              # "TPB_min_R"
              # "TPB_min_L"
              # "TPB_max_R"
              # "TPB_max_L"
              # "I_trialUntilReward"
              # "ENL_penalty"
              # "ENL_min"
              # "ENL_max"
              # "BUR_max"
              # "BUR_min"
              # "CueCycles"
              # "Audio_Freq_R"
              # "Audio_Freq_L"
              # "Audio_Amp_R"
              # "Audio_Amp_L"
              n77 = call "myRIO_BRig_RT_dataExp_CueCycles.vi"() -> ("output_CueCycles"=w264:i32)  [unwired: 11 in]
              n78 = call "myRIO_BRig_RT_dataExp_Audio_amp__R.vi"() -> ("output_Audio_amp__R"=w268:i32)  [unwired: 11 in]
              n79 = call "myRIO_BRig_RT_dataExp_Audio_amp__L.vi"() -> ("output_Audio_amp__L"=w270:i32)  [unwired: 11 in]
              n80 = call "myRIO_BRig_RT_dataExp_Tcycle_Reward__L.vi"() -> ("output_Tcycle_Reward__L"=w241:i32)  [unwired: 11 in]
              n81 = call "myRIO_BRig_RT_dataExp_Tcycle_Reward__R.vi"() -> ("output_Tcycle_Reward__R"=w240:i32)  [unwired: 11 in]
              n82 = call "myRIO_BRig_RT_dataExp_Tcycle_RewardPost.vi"() -> ("output_Tcycle_RewardPost"=w239:i32)  [unwired: 11 in]
              n83 = call "myRIO_BRig_RT_dataExp_BUR_min.vi"() -> ("output_BUR_min"=w261:i32)  [unwired: 11 in]
              n84 = call "myRIO_BRig_RT_dataExp_ENL_min.vi"() -> ("output_ENL_min"=w257:i32)  [unwired: 11 in]
              n85 = call "myRIO_BRig_RT_dataExp_TPB_max__L.vi"() -> ("output_TPB_max__L"=w249:i32)  [unwired: 11 in]
              n86 = call "myRIO_BRig_RT_dataExp_TPB_max__R.vi"() -> ("output_TPB_max__R"=w248:i32)  [unwired: 11 in]
              n87 = call "myRIO_BRig_RT_dataExp_ENL_penalty.vi"() -> ("output_ENL_penalty"=w256:i32)  [unwired: 11 in]
              n88 = call "myRIO_BRig_RT_dataExp_Audio_freq__L.vi"() -> ("output_Audio_freq__L"=w266:i32)  [unwired: 11 in]
              n89 = call "myRIO_BRig_RT_dataExp_Audio_freq__R.vi"() -> ("output_Audio_freq__R"=w265:i32)  [unwired: 11 in]
              n90 = call "myRIO_BRig_RT_dataExp_BUR_max.vi"() -> ("output_BUR_max"=w262:i32)  [unwired: 11 in]
              n91 = call "myRIO_BRig_RT_dataExp_ENL_max.vi"() -> ("output_ENL_max"=w258:i32)  [unwired: 11 in]
              n92 = call "myRIO_BRig_RT_dataExp_ItrialUntilReward.vi"() -> ("output_I_trialUntilReward"=w252:i32)  [unwired: 11 in]
              n93 = call "myRIO_BRig_RT_dataExp_Tcycle_Selection.vi"() -> ("output_Tcycle_Selection"=w238:i32)  [unwired: 11 in]
              n94 = call "myRIO_BRig_RT_dataExp_Tcycle_Wrong.vi"() -> ("output_Tcycle_Wrong"=w237:i32)  [unwired: 11 in]
              n95 = call "myRIO_BRig_RT_dataExp_Tcycle_Timeout.vi"() -> ("output_Tcycle_Timeout"=w236:i32)  [unwired: 11 in]
              n96 = call "myRIO_BRig_RT_dataExp_TPB_min__L.vi"() -> ("output_TPB_min__L"=w247:i32)  [unwired: 11 in]
              n97 = call "myRIO_BRig_RT_dataExp_TPB_min__R.vi"() -> ("output_TPB_min__R"=w246:i32)  [unwired: 11 in]
              n98 = call "myRIO_BRig_RT_dataExp_Tcycle_Cue1Penalty_Audio.vi"() -> ("output_Tcycle_Cue1Penalty_Audio"=w229:i32)  [unwired: 11 in]
              n99 = call "myRIO_BRig_RT_dataExp_Tcycle_Cue1_Audio_min.vi"() -> ("output_Tcycle_Cue1_Audio_min"=w228:i32)  [unwired: 11 in]
              n100 = call "myRIO_BRig_RT_dataExp_Tcycle_Cue1_Audio_max.vi"() -> ("output_Tcycle_Cue1_Audio_max"=w227:i32)  [unwired: 11 in]
              n101 = call "myRIO_BRig_RT_dataExp_Tcycle_Cue1Penalty_LED.vi"() -> ("output_Tcycle_Cue1Penalty_LED"=w218:i32)  [unwired: 11 in]
              n102 = call "myRIO_BRig_RT_dataExp_Tcycle_Cue1_LED_min.vi"() -> ("output_Tcycle_Cue1_LED_min"=w217:i32)  [unwired: 11 in]
              n103 = call "myRIO_BRig_RT_dataExp_Tcycle_Cue1_LED_max.vi"() -> ("output_Tcycle_Cue1_LED_max"=w216:i32)  [unwired: 11 in]
              n104 = Index Array(array=w221, index #1=w270, index #2=w268, index #3=w266, index #4=w265, index #5=w264, index #6=w262, index #7=w261, index #8=w258, index #9=w257, index #10=w256, index #11=w252, index #12=w249, index #13=w248, index #14=w247, index #15=w246, index #16=w241, index #17=w240, index #18=w239, index #19=w238, index #20=w237, index #21=w236, index #22=w229, index #23=w228, index #24=w227, index #25=w218, index #26=w217, index #27=w216) -> (element #1=w269:u16, element #2=w267:u16, element #3=w224:u16, element #4=w223:u16, element #5=w263:u16, element #6=w260:u16, element #7=w259:u16, element #8=w255:u16, element #9=w254:u16, element #10=w253:u16, element #11=w250:u16, element #12=w245:u16, element #13=w244:u16, element #14=w243:u16, element #15=w242:u16, element #16=w235:u16, element #17=w234:u16, element #18=w233:u16, element #19=w232:u16, element #20=w231:u16, element #21=w230:u16, element #22=w226:u16, element #23=w220:u16, element #24=w219:u16, element #25=w215:u16, element #26=w214:u16, element #27=w213:u16)
              n105 = local write "Tcycle_CuePenalty_LED"(w215) -> ()
              n106 = local write "Tcycle_Cue_LED_min"(w214) -> ()
              n107 = local write "Tcycle_Cue_LED_max"(w213) -> ()
              n108 = local write "Tcycle_Selection"(w232) -> ()
              n109 = local write "Tcycle_Wrong"(w231) -> ()
              n110 = local write "Tcycle_Timeout"(w230) -> ()
              n111 = local write "Audio_Amp__L"(w269) -> ()
              n112 = local write "Audio_Amp__R"(w267) -> ()
              n113 = local write "Tcycle_ENLPenalty"(w253) -> ()
              n114 = local write "Tcycle_ENL_max"(w255) -> ()
              n115 = local write "TpB_Min_L"(w243) -> ()
              n116 = local write "TpB_Min_R"(w242) -> ()
              n117 = local write "Tcycle_CuePenalty_Audio"(w226) -> ()
              n118 = local write "Tcycle_Cue_Audio_min"(w220) -> ()
              n119 = local write "Tcycle_Cue_Audio_max"(w219) -> ()
              n120 = To Unsigned Byte Integer(number=w224) -> (unsigned 8bit integer=w225:u8)
              n121 = To Unsigned Byte Integer(number=w223) -> (unsigned 8bit integer=w222:u8)
              n122 = Not Equal To 0?(x=w250) -> (x != 0?=w251:bool)
              n123 = local write "Tcycle_Reward_L"(w235) -> ()
              n124 = local write "Tcycle_Reward_R"(w234) -> ()
              n125 = local write "Tcycle_RewardPost"(w233) -> ()
              n126 = local write "CueCycles"(w263) -> ()
              n127 = local write "BUR_min"(w259) -> ()
              n128 = local write "BUR_max"(w260) -> ()
              n129 = local write "Tcycle_ENL_min"(w254) -> ()
              n130 = local write "TpB_Max_L"(w245) -> ()
              n131 = local write "TpB_Max_R"(w244) -> ()
              n132 = local write "TrialUntilReward"(w251) -> ()
              n133 = local write "Audio_Freq__L"(w225) -> ()
              n134 = local write "Audio_Freq__R"(w222) -> ()
            }
            frame "UploadSettings_dataExp_2" {
              w292 = 100.0 ("y")
              n135 = call "myRIO_BRig_RT_dataExp_FPGA_f_count2ms.vi"() -> ("output_FPGA_f_count2ms"=w353:i32)  [unwired: 11 in]
              n136 = call "myRIO_BRig_RT_dataExp_laser1_Freq.vi"() -> ("output_laser1_Freq"=w341:i32)  [unwired: 11 in]
              n137 = call "myRIO_BRig_RT_dataExp_laser1_duration.vi"() -> ("output_laser1_duration"=w340:i32)  [unwired: 11 in]
              n138 = call "myRIO_BRig_RT_dataExp_laser1_Tpeak.vi"() -> ("output_laser1_Tpeak"=w339:i32)  [unwired: 11 in]
              n139 = call "myRIO_BRig_RT_dataExp_laser1_Tshutter.vi"() -> ("output_laser1_Tshutter"=w338:i32)  [unwired: 11 in]
              n140 = call "myRIO_BRig_RT_dataExp_laser1_Power_min.vi"() -> ("output_laser1_Power_min"=w337:i32)  [unwired: 11 in]
              n141 = call "myRIO_BRig_RT_dataExp_laser1_Power_max.vi"() -> ("output_laser1_Power_max"=w336:i32)  [unwired: 11 in]
              n142 = call "myRIO_BRig_RT_dataExp_laser1_Power_step.vi"() -> ("output_laser1_Power_step"=w335:i32)  [unwired: 11 in]
              n143 = call "myRIO_BRig_RT_dataExp_Cue1Param_CueType_Switch.vi"() -> ("output_Cue1Param_CueType_Switch"=w286:i32)  [unwired: 11 in]
              n144 = call "myRIO_BRig_RT_dataExp_Cue1Param_AudioLed_Count_Switch.vi"() -> ("output_Cue1Param_AudioLed_Count_Switch"=w285:i32)  [unwired: 11 in]
              n145 = call "myRIO_BRig_RT_dataExp_Cue1Param_AudioLed_Probability_Switch.vi"() -> ("output_Cue1Param_AudioLed_Probability_Switch"=w284:i32)  [unwired: 11 in]
              n146 = call "myRIO_BRig_RT_dataExp_SolenoidProbability_L.vi"() -> ("output_SolenoidProbability_L"=w288:i32)  [unwired: 11 in]
              n147 = call "myRIO_BRig_RT_dataExp_SolenoidProbability_R.vi"() -> ("output_SolenoidProbability_R"=w287:i32)  [unwired: 11 in]
              n148 = call "myRIO_BRig_RT_dataExp_Cue1Param_CueType_NS.vi"() -> ("output_Cue1Param_CueType_NS"=w283:i32)  [unwired: 11 in]
              n149 = call "myRIO_BRig_RT_dataExp_Cue1Param_AudioLed_Count_NS.vi"() -> ("output_Cue1Param_AudioLed_Count_NS"=w282:i32)  [unwired: 11 in]
              n150 = call "myRIO_BRig_RT_dataExp_Cue1Param_AudioLed_Probability_NS.vi"() -> ("output_Cue1Param_AudioLed_Probability_NS"=w281:i32)  [unwired: 11 in]
              n151 = call "myRIO_BRig_RT_dataExp_laser2_Freq.vi"() -> ("output_laser2_Freq"=w334:i32)  [unwired: 11 in]
              n152 = call "myRIO_BRig_RT_dataExp_laser2_duration.vi"() -> ("output_laser2_duration"=w333:i32)  [unwired: 11 in]
              n153 = call "myRIO_BRig_RT_dataExp_laser2_Tpeak.vi"() -> ("output_laser2_Tpeak"=w332:i32)  [unwired: 11 in]
              n154 = call "myRIO_BRig_RT_dataExp_laser2_Tshutter.vi"() -> ("output_laser2_Tshutter"=w331:i32)  [unwired: 11 in]
              n155 = call "myRIO_BRig_RT_dataExp_laser2_Power_min.vi"() -> ("output_laser2_Power_min"=w330:i32)  [unwired: 11 in]
              n156 = call "myRIO_BRig_RT_dataExp_laser2_Power_max.vi"() -> ("output_laser2_Power_max"=w329:i32)  [unwired: 11 in]
              n157 = call "myRIO_BRig_RT_dataExp_laser2_Power_step.vi"() -> ("output_laser2_Power_step"=w328:i32)  [unwired: 11 in]
              n158 = call "myRIO_BRig_RT_dataExp_CueLed_Freq.vi"() -> ("output_CueLed_Freq"=w297:i32)  [unwired: 11 in]
              n159 = call "myRIO_BRig_RT_dataExp_CueLed_Tpeak.vi"() -> ("output_CueLed_Tpeak"=w290:i32)  [unwired: 11 in]
              n160 = Index Array(array=w354, index #1=w353, index #2=w341, index #3=w340, index #4=w339, index #5=w338, index #6=w337, index #7=w336, index #8=w335, index #9=w334, index #10=w333, index #11=w332, index #12=w331, index #13=w330, index #14=w329, index #15=w328, index #16=w297, index #17=w290, index #18=w288, index #19=w287, index #20=w286, index #21=w285, index #22=w284, index #23=w283, index #24=w282, index #25=w281) -> (element #1=w352:u16, element #2=w327:u16, element #3=w326:u16, element #4=w325:u16, element #5=w324:u16, element #6=w323:u16, element #7=w313:u16, element #8=w312:u16, element #9=w308:u16, element #10=w307:u16, element #11=w306:u16, element #12=w305:u16, element #13=w304:u16, element #14=w299:u16, element #15=w298:u16, element #16=w291:u16, element #17=w289:u16, element #18=w280:u16, element #19=w279:u16, element #20=w278:u16, element #21=w277:u16, element #22=w276:u16, element #23=w275:u16, element #24=w274:u16, element #25=w273:u16)
              n161 = local write "Cue1Param_CueType_Switch"(w278) -> ()
              n162 = local write "Cue1Param_AudioLed_Count_Switch"(w277) -> ()
              n163 = local write "Cue1Param_AudioLed_Probability_Switch"(w276) -> ()
              n164 = local write "Cue1Param_CueType_NS"(w275) -> ()
              n165 = local write "Cue1Param_AudioLed_Count_NS"(w274) -> ()
              n166 = local write "Cue1Param_AudioLed_Probability_NS"(w273) -> ()
              n167 = To Double Precision Float(number=w352) -> (double precision float=w351:dbl)
              n168 = To Double Precision Float(number=w327) -> (double precision float=w349:dbl)
              n169 = To Double Precision Float(number=w325) -> (double precision float=w346:dbl)
              n170 = To Double Precision Float(number=w324) -> (double precision float=w345:dbl)
              n171 = To Double Precision Float(number=w323) -> (double precision float=w347:dbl)
              n172 = To Double Precision Float(number=w313) -> (double precision float=w318:dbl)
              n173 = To Double Precision Float(number=w312) -> (double precision float=w314:dbl)
              n174 = To Double Precision Float(number=w308) -> (double precision float=w319:dbl)
              n175 = To Double Precision Float(number=w306) -> (double precision float=w321:dbl)
              n176 = To Double Precision Float(number=w305) -> (double precision float=w322:dbl)
              n177 = To Double Precision Float(number=w304) -> (double precision float=w320:dbl)
              n178 = To Double Precision Float(number=w299) -> (double precision float=w302:dbl)
              n179 = To Double Precision Float(number=w298) -> (double precision float=w303:dbl)
              n180 = To Double Precision Float(number=w291) -> (double precision float=w296:dbl)
              n181 = To Double Precision Float(number=w289) -> (double precision float=w295:dbl)
              n182 = local write "SolenoidProbability_L"(w280) -> ()
              n183 = local write "SolenoidProbability_R"(w279) -> ()
              n184 = Divide(x=w351, y=w292) -> (x/y=w350:dbl)
              n185 = Divide(x=w349, y=w292) -> (x/y=w348:dbl)
              n186 = Divide(x=w346, y=w292) -> (x/y=w343:dbl)
              n187 = Divide(x=w345, y=w292) -> (x/y=w342:dbl)
              n188 = Divide(x=w347, y=w292) -> (x/y=w344:dbl)
              n189 = Divide(x=w318, y=w292) -> (x/y=w316:dbl)
              n190 = Divide(x=w314, y=w292) -> (x/y=w315:dbl)
              n191 = Divide(x=w319, y=w292) -> (x/y=w317:dbl)
              n192 = Divide(x=w321, y=w292) -> (x/y=w311:dbl)
              n193 = Divide(x=w322, y=w292) -> (x/y=w310:dbl)
              n194 = Divide(x=w320, y=w292) -> (x/y=w309:dbl)
              n195 = Divide(x=w302, y=w292) -> (x/y=w301:dbl)
              n196 = Divide(x=w303, y=w292) -> (x/y=w300:dbl)
              n197 = Divide(x=w296, y=w292) -> (x/y=w294:dbl)
              n198 = Divide(x=w295, y=w292) -> (x/y=w293:dbl)
              n199 = local write "FPGA_count2ms"(w350) -> ()
              n200 = local write "Laser_Freq_l1"(w348) -> ()
              n201 = local write "Laser_duration_l1"(w326) -> ()
              n202 = local write "Laser_Tpeak_l1"(w343) -> ()
              n203 = local write "Laser_Tshutter_l1"(w342) -> ()
              n204 = local write "Laser_power_min_l1"(w344) -> ()
              n205 = local write "Laser_power_max_l1"(w316) -> ()
              n206 = local write "Laser_power_step_l1"(w315) -> ()
              n207 = local write "Laser_Freq_l2"(w317) -> ()
              n208 = local write "Laser_duration_l2"(w307) -> ()
              n209 = local write "Laser_Tpeak_l2"(w311) -> ()
              n210 = local write "Laser_Tshutter_l2"(w310) -> ()
              n211 = local write "Laser_power_min_l2"(w309) -> ()
              n212 = local write "Laser_power_max_l2"(w301) -> ()
              n213 = local write "Laser_power_step_l2"(w300) -> ()
              n214 = local write "CueLed_Freq"(w294) -> ()
              n215 = local write "CueLed_Tpeak"(w293) -> ()
            }
            frame "UploadSettings_dataLC_1" {
              # "Cue1_delayOpt_NonSwitch"
              # "ENL1_delayOpt_NonSwitch"
              # "Cue1_delayOpt_Switch"
              # "ENL1_delayOpt_Switch"
              # "Count"
              # "Tdelay"
              # "Prob"
              # "OnOff"
              # "Block"
              # "Count"
              # "Tdelay"
              # "Prob"
              # "OnOff"
              # "Block"
              # "Count"
              # "Tdelay"
              # "Prob"
              # "OnOff"
              # "Block"
              # "ENL1 Switch"
              # "Cue1 NonSwitch"
              # "Cue1 Switch"
              # "ENL1 NonSwitch"
              # "Count"
              # "Tdelay"
              # "Prob"
              # "OnOff"
              # "Block"
              n216 = call "myRIO_BRig_RT_dataLC_ENL1_OnOff_Switch_l1.vi"() -> ("output_ENL1_OnOff_Switch_l1"=w408:i32)  [unwired: 11 in]
              n217 = call "myRIO_BRig_RT_dataLC_ENL1_Tdelay_Switch_l1.vi"() -> ("output_ENL1_Tdelay_Switch_l1"=w407:i32)  [unwired: 11 in]
              n218 = call "myRIO_BRig_RT_dataLC_ENL1_Block_Switch_l1.vi"() -> ("output_ENL1_Block_Switch_l1"=w406:i32)  [unwired: 11 in]
              n219 = call "myRIO_BRig_RT_dataLC_ENL1_Count_Switch_l1.vi"() -> ("output_ENL1_Count_Switch_l1"=w405:i32)  [unwired: 11 in]
              n220 = call "myRIO_BRig_RT_dataLC_ENL1_Probability_Switch_l1.vi"() -> ("output_ENL1_Probability_Switch_l1"=w404:i32)  [unwired: 11 in]
              n221 = call "myRIO_BRig_RT_dataLC_ENL1_OnOff_NS_l1.vi"() -> ("output_ENL1_OnOff_NS_l1"=w403:i32)  [unwired: 11 in]
              n222 = call "myRIO_BRig_RT_dataLC_ENL1_Tdelay_NS_l1.vi"() -> ("output_ENL1_Tdelay_NS_l1"=w402:i32)  [unwired: 11 in]
              n223 = call "myRIO_BRig_RT_dataLC_ENL1_Block_NS_l1.vi"() -> ("output_ENL1_All_Block"=w401:i32)  [unwired: 11 in]
              n224 = call "myRIO_BRig_RT_dataLC_ENL1_Count_NS_l1.vi"() -> ("output_ENL1_Count_NS_l1"=w400:i32)  [unwired: 11 in]
              n225 = call "myRIO_BRig_RT_dataLC_ENL1_Probability_NS_l1.vi"() -> ("output_ENL1_Probability_NS_l1"=w399:i32)  [unwired: 11 in]
              n226 = call "myRIO_BRig_RT_dataLC_Cue1_OnOff_Switch_l1.vi"() -> ("output_Cue1_OnOff_Switch_l1"=w398:i32)  [unwired: 11 in]
              n227 = call "myRIO_BRig_RT_dataLC_Cue1_Tdelay_Switch_l1.vi"() -> ("output_Cue1_Tdelay_Switch_l1"=w397:i32)  [unwired: 11 in]
              n228 = call "myRIO_BRig_RT_dataLC_Cue1_Block_Switch_l1.vi"() -> ("output_Cue1_Block_Switch_l1"=w396:i32)  [unwired: 11 in]
              n229 = call "myRIO_BRig_RT_dataLC_Cue1_Count_Switch_l1.vi"() -> ("output_Cue1_Count_Switch_l1"=w395:i32)  [unwired: 11 in]
              n230 = call "myRIO_BRig_RT_dataLC_Cue1_Probability_Switch_l1.vi"() -> ("output_Cue1_Probability_Switch_l1"=w394:i32)  [unwired: 11 in]
              n231 = call "myRIO_BRig_RT_dataLC_Cue1_OnOff_NS_l1.vi"() -> ("output_Cue1_OnOff_NS_l1"=w393:i32)  [unwired: 11 in]
              n232 = call "myRIO_BRig_RT_dataLC_Cue1_Tdelay_NS_l1.vi"() -> ("output_Cue1_Tdelay_NS_l1"=w392:i32)  [unwired: 11 in]
              n233 = call "myRIO_BRig_RT_dataLC_Cue1_Block_NS_l1.vi"() -> ("output_Cue1_Block_NS_l1"=w391:i32)  [unwired: 11 in]
              n234 = call "myRIO_BRig_RT_dataLC_Cue1_Count_NS_l1.vi"() -> ("output_Cue1_Count_NS_l1"=w390:i32)  [unwired: 11 in]
              n235 = call "myRIO_BRig_RT_dataLC_Cue1_Probability_NS_l1.vi"() -> ("output_Cue1_l1_All_Probability"=w389:i32)  [unwired: 11 in]
              n236 = call "myRIO_BRig_RT_dataLC_ENL1_delayOpt_Switch_l1.vi"() -> ("output_ENL1_delayOpt_Switch_l1"=w368:i32)  [unwired: 11 in]
              n237 = call "myRIO_BRig_RT_dataLC_ENL1_delayOpt_NS_l1.vi"() -> ("output_ENL1_delayOpt_NS_l1"=w367:i32)  [unwired: 11 in]
              n238 = call "myRIO_BRig_RT_dataLC_Cue1_delayOpt_Switch_l1.vi"() -> ("output_Cue1_delayOpt_Switch_l1"=w366:i32)  [unwired: 11 in]
              n239 = call "myRIO_BRig_RT_dataLC_Cue1_delayOpt_NS_l1.vi"() -> ("output_Cue1_delayOpt_NS_l1"=w365:i32)  [unwired: 11 in]
              n240 = Index Array(array=w410, index #1=w408, index #2=w407, index #3=w406, index #4=w405, index #5=w404, index #6=w403, index #7=w402, index #8=w401, index #9=w400, index #10=w399, index #11=w398, index #12=w397, index #13=w396, index #14=w395, index #15=w394, index #16=w393, index #17=w392, index #18=w391, index #19=w390, index #20=w389, index #21=w368, index #22=w367, index #23=w366, index #24=w365) -> (element #1=w388:u16, element #2=w387:u16, element #3=w386:u16, element #4=w385:u16, element #5=w384:u16, element #6=w383:u16, element #7=w382:u16, element #8=w381:u16, element #9=w380:u16, element #10=w379:u16, element #11=w378:u16, element #12=w377:u16, element #13=w376:u16, element #14=w375:u16, element #15=w374:u16, element #16=w373:u16, element #17=w372:u16, element #18=w371:u16, element #19=w370:u16, element #20=w369:u16, element #21=w360:u16, element #22=w359:u16, element #23=w358:u16, element #24=w357:u16)
              n241 = Not Equal To 0?(x=w388) -> (x != 0?=w412:bool)
              n242 = Not Equal To 0?(x=w383) -> (x != 0?=w411:bool)
              n243 = Not Equal To 0?(x=w378) -> (x != 0?=w414:bool)
              n244 = Not Equal To 0?(x=w373) -> (x != 0?=w413:bool)
              n245 = Not Equal To 0?(x=w360) -> (x != 0?=w362:bool)
              n246 = Not Equal To 0?(x=w359) -> (x != 0?=w363:bool)
              n247 = Not Equal To 0?(x=w358) -> (x != 0?=w364:bool)
              n248 = Not Equal To 0?(x=w357) -> (x != 0?=w361:bool)
              n249 = local write "LC_ENL1_OnOff_Switch_l1"(w412) -> ()
              n250 = local write "LC_ENL1_Tdelay_Switch_l1"(w387) -> ()
              n251 = local write "LC_ENL1_Block_Switch_l1"(w386) -> ()
              n252 = local write "LC_ENL1_Count_Switch_l1"(w385) -> ()
              n253 = local write "LC_ENL1_Probability_Switch_l1"(w384) -> ()
              n254 = local write "LC_ENL1_OnOff_NS_l1"(w411) -> ()
              n255 = local write "LC_ENL1_Tdelay_NS_l1"(w382) -> ()
              n256 = local write "LC_ENL1_Block_NS_l1"(w381) -> ()
              n257 = local write "LC_ENL1_Count_NS_l1"(w380) -> ()
              n258 = local write "LC_ENL1_Probability_NS_l1"(w379) -> ()
              n259 = local write "LC_Cue1_OnOff_Switch_l1"(w414) -> ()
              n260 = local write "LC_Cue1_Tdelay_Switch_l1"(w377) -> ()
              n261 = local write "LC_Cue1_Block_Switch_l1"(w376) -> ()
              n262 = local write "LC_Cue1_Count_Switch_l1"(w375) -> ()
              n263 = local write "LC_Cue1_Probability_Switch_l1"(w374) -> ()
              n264 = local write "LC_Cue1_OnOff_NS_l1"(w413) -> ()
              n265 = local write "LC_Cue1_Tdelay_NS_l1"(w372) -> ()
              n266 = local write "LC_Cue1_Block_NS_l1"(w371) -> ()
              n267 = local write "LC_Cue1_Count_NS_l1"(w370) -> ()
              n268 = local write "LC_Cue1_Probability_NS_l1"(w369) -> ()
              n269 = local write "LC_ENL1_delayOpt_Switch_l1"(w362) -> ()
              n270 = local write "LC_ENL1_delayOpt_NS_l1"(w363) -> ()
              n271 = local write "LC_Cue1_delayOpt_Switch_l1"(w364) -> ()
              n272 = local write "LC_Cue1_delayOpt_NS_l1"(w361) -> ()
            }
            frame "UploadSettings_dataLC_3" {
              # "Cue1_delayOpt_NonSwitch"
              # "ENL1_delayOpt_NonSwitch"
              # "Cue1_delayOpt_Switch"
              # "ENL1_delayOpt_Switch"
              # "Count"
              # "Tdelay"
              # "Prob"
              # "OnOff"
              # "Block"
              # "Count"
              # "Tdelay"
              # "Prob"
              # "OnOff"
              # "Block"
              # "Count"
              # "Tdelay"
              # "Prob"
              # "OnOff"
              # "Block"
              # "ENL1 Switch"
              # "Cue1 NonSwitch"
              # "Cue1 Switch"
              # "ENL1 NonSwitch"
              # "Count"
              # "Tdelay"
              # "Prob"
              # "OnOff"
              # "Block"
              n273 = call "myRIO_BRig_RT_dataLC_ENL1_OnOff_Switch_l2.vi"() -> ("output_ENL1_OnOff_Switch_l2"=w435:i32)  [unwired: 11 in]
              n274 = call "myRIO_BRig_RT_dataLC_ENL1_Tdelay_Switch_l2.vi"() -> ("output_ENL1_Tdelay_Switch_l2"=w436:i32)  [unwired: 11 in]
              n275 = call "myRIO_BRig_RT_dataLC_ENL1_Block_Switch_l2.vi"() -> ("output_ENL1_Block_Switch_l2"=w437:i32)  [unwired: 11 in]
              n276 = call "myRIO_BRig_RT_dataLC_ENL1_Count_Switch_l2.vi"() -> ("output_ENL1_Count_Switch_l2"=w438:i32)  [unwired: 11 in]
              n277 = call "myRIO_BRig_RT_dataLC_ENL1_Probability_Switch_l2.vi"() -> ("output_ENL1_Probability_Switch_l2"=w439:i32)  [unwired: 11 in]
              n278 = call "myRIO_BRig_RT_dataLC_ENL1_OnOff_NS_l2.vi"() -> ("output_ENL1_OnOff_NS_l2"=w430:i32)  [unwired: 11 in]
              n279 = call "myRIO_BRig_RT_dataLC_ENL1_Tdelay_NS_l2.vi"() -> ("output_ENL1_Tdelay_NS_l2"=w431:i32)  [unwired: 11 in]
              n280 = call "myRIO_BRig_RT_dataLC_ENL1_Block_NS_l2.vi"() -> ("output_ENL1_Block_NS_l2"=w432:i32)  [unwired: 11 in]
              n281 = call "myRIO_BRig_RT_dataLC_ENL1_Count_NS_l2.vi"() -> ("output_ENL1_Count_NS_l2"=w433:i32)  [unwired: 11 in]
              n282 = call "myRIO_BRig_RT_dataLC_ENL1_Probability_NS_l2.vi"() -> ("output_ENL1_Probability_NS_l2"=w434:i32)  [unwired: 11 in]
              n283 = call "myRIO_BRig_RT_dataLC_Cue1_OnOff_Switch_l2.vi"() -> ("output_Cue1_OnOff_Switch_l2"=w425:i32)  [unwired: 11 in]
              n284 = call "myRIO_BRig_RT_dataLC_Cue1_Tdelay_Switch_l2.vi"() -> ("output_Cue1_Tdelay_Switch_l2"=w426:i32)  [unwired: 11 in]
              n285 = call "myRIO_BRig_RT_dataLC_Cue1_Block_Switch_l2.vi"() -> ("output_Cue1_Block_Switch_l2"=w427:i32)  [unwired: 11 in]
              n286 = call "myRIO_BRig_RT_dataLC_Cue1_Count_Switch_l2.vi"() -> ("output_Cue1_Count_Switch_l2"=w428:i32)  [unwired: 11 in]
              n287 = call "myRIO_BRig_RT_dataLC_Cue1_Probability_Switch_l2.vi"() -> ("output_Cue1_l2_First_Probability"=w429:i32)  [unwired: 11 in]
              n288 = call "myRIO_BRig_RT_dataLC_Cue1_OnOff_NS_l2.vi"() -> ("output_Cue1_OnOff_NS_l2"=w420:i32)  [unwired: 11 in]
              n289 = call "myRIO_BRig_RT_dataLC_Cue1_Tdelay_NS_l2.vi"() -> ("output_Cue1_Tdelay_NS_l2"=w421:i32)  [unwired: 11 in]
              n290 = call "myRIO_BRig_RT_dataLC_Cue1_Block_NS_l2.vi"() -> ("output_Cue1_Block_NS_l2"=w422:i32)  [unwired: 11 in]
              n291 = call "myRIO_BRig_RT_dataLC_Cue1_Count_NS_l2.vi"() -> ("output_Cue1_Count_NS_l2"=w423:i32)  [unwired: 11 in]
              n292 = call "myRIO_BRig_RT_dataLC_Cue1_Probability_NS_l2.vi"() -> ("output_Cue1_l2_All_Probability"=w424:i32)  [unwired: 11 in]
              n293 = call "myRIO_BRig_RT_dataLC_ENL1_delayOpt_Switch_l2.vi"() -> ("output_ENL1_delayOpt_Switch_l2"=w416:i32)  [unwired: 11 in]
              n294 = call "myRIO_BRig_RT_dataLC_ENL1_delayOpt_NS_l2.vi"() -> ("output_ENL1_delayOpt_NS_l2"=w417:i32)  [unwired: 11 in]
              n295 = call "myRIO_BRig_RT_dataLC_Cue1_delayOpt_Switch_l2.vi"() -> ("output_Cue1_delayOpt_Switch_l2"=w418:i32)  [unwired: 11 in]
              n296 = call "myRIO_BRig_RT_dataLC_Cue1_delayOpt_NS_l2.vi"() -> ("output_Cue1_delayOpt_NS_l2"=w419:i32)  [unwired: 11 in]
              n297 = Index Array(array=w469, index #1=w435, index #2=w436, index #3=w437, index #4=w438, index #5=w439, index #6=w430, index #7=w431, index #8=w432, index #9=w433, index #10=w434, index #11=w425, index #12=w426, index #13=w427, index #14=w428, index #15=w429, index #16=w420, index #17=w421, index #18=w422, index #19=w423, index #20=w424, index #21=w416, index #22=w417, index #23=w418, index #24=w419) -> (element #1=w467:u16, element #2=w466:u16, element #3=w465:u16, element #4=w464:u16, element #5=w463:u16, element #6=w462:u16, element #7=w461:u16, element #8=w460:u16, element #9=w459:u16, element #10=w458:u16, element #11=w457:u16, element #12=w456:u16, element #13=w455:u16, element #14=w454:u16, element #15=w453:u16, element #16=w452:u16, element #17=w451:u16, element #18=w450:u16, element #19=w449:u16, element #20=w448:u16, element #21=w443:u16, element #22=w442:u16, element #23=w441:u16, element #24=w440:u16)
              n298 = Not Equal To 0?(x=w467) -> (x != 0?=w471:bool)
              n299 = Not Equal To 0?(x=w462) -> (x != 0?=w470:bool)
              n300 = Not Equal To 0?(x=w457) -> (x != 0?=w473:bool)
              n301 = Not Equal To 0?(x=w452) -> (x != 0?=w472:bool)
              n302 = Not Equal To 0?(x=w443) -> (x != 0?=w445:bool)
              n303 = Not Equal To 0?(x=w442) -> (x != 0?=w446:bool)
              n304 = Not Equal To 0?(x=w441) -> (x != 0?=w447:bool)
              n305 = Not Equal To 0?(x=w440) -> (x != 0?=w444:bool)
              n306 = local write "LC_ENL1_OnOff_Switch_l2"(w471) -> ()
              n307 = local write "LC_ENL1_Tdelay_Switch_l2"(w466) -> ()
              n308 = local write "LC_ENL1_Block_Switch_l2"(w465) -> ()
              n309 = local write "LC_ENL1_Count_Switch_l2"(w464) -> ()
              n310 = local write "LC_ENL1_Probability_Switch_l2"(w463) -> ()
              n311 = local write "LC_ENL1_OnOff_NS_l2"(w470) -> ()
              n312 = local write "LC_ENL1_Tdelay_NS_l2"(w461) -> ()
              n313 = local write "LC_ENL1_Block_NS_l2"(w460) -> ()
              n314 = local write "LC_ENL1_Count_NS_l2"(w459) -> ()
              n315 = local write "LC_ENL1_Probability_NS_l2"(w458) -> ()
              n316 = local write "LC_Cue1_OnOff_Switch_l2"(w473) -> ()
              n317 = local write "LC_Cue1_Tdelay_Switch_l2"(w456) -> ()
              n318 = local write "LC_Cue1_Block_Switch_l2"(w455) -> ()
              n319 = local write "LC_Cue1_Count_Switch_l2"(w454) -> ()
              n320 = local write "LC_Cue1_Probability_Switch_l2"(w453) -> ()
              n321 = local write "LC_Cue1_OnOff_NS_l2"(w472) -> ()
              n322 = local write "LC_Cue1_Tdelay_NS_l2"(w451) -> ()
              n323 = local write "LC_Cue1_Block_NS_l2"(w450) -> ()
              n324 = local write "LC_Cue1_Count_NS_l2"(w449) -> ()
              n325 = local write "LC_Cue1_Probability_NS_l2"(w448) -> ()
              n326 = local write "LC_ENL1_delayOpt_Switch_l2"(w445) -> ()
              n327 = local write "LC_ENL1_delayOpt_NS_l2"(w446) -> ()
              n328 = local write "LC_Cue1_delayOpt_Switch_l2"(w447) -> ()
              n329 = local write "LC_Cue1_delayOpt_NS_l2"(w444) -> ()
            }
            frame "UploadSettings_dataLC_2" {
              # "Count"
              # "Tdelay"
              # "Prob"
              # "OnOff"
              # "Block"
              # "Selection NonSwitch"
              # "Count"
              # "Tdelay"
              # "Prob"
              # "OnOff"
              # "Block"
              # "Selection Switch"
              # "Trial"
              # "Tdelay"
              # "Prob"
              # "OnOff"
              # "Block"
              # "Wrong"
              # "Reward"
              # "Trial"
              # "Tdelay"
              # "Prob"
              # "OnOff"
              # "Block"
              n330 = call "myRIO_BRig_RT_dataLC_Reward_OnOff_l1.vi"() -> ("output_Reward_OnOff_l1"=w516:i32)  [unwired: 11 in]
              n331 = call "myRIO_BRig_RT_dataLC_Reward_Tdelay_l1.vi"() -> ("output_Reward_Tdelay_l1"=w515:i32)  [unwired: 11 in]
              n332 = call "myRIO_BRig_RT_dataLC_Reward_Block_l1.vi"() -> ("output_Reward_Block_l1"=w514:i32)  [unwired: 11 in]
              n333 = call "myRIO_BRig_RT_dataLC_Reward_Trial_l1.vi"() -> ("output_Reward_Trial_l1"=w513:i32)  [unwired: 11 in]
              n334 = call "myRIO_BRig_RT_dataLC_Reward_Probability_l1.vi"() -> ("output_Reward_Probability_l1"=w512:i32)  [unwired: 11 in]
              n335 = call "myRIO_BRig_RT_dataLC_Wrong_OnOff_l1.vi"() -> ("output_Wrong_OnOff_l1"=w505:i32)  [unwired: 11 in]
              n336 = call "myRIO_BRig_RT_dataLC_Wrong_Tdelay_l1.vi"() -> ("output_Wrong_Tdelay_l1"=w504:i32)  [unwired: 11 in]
              n337 = call "myRIO_BRig_RT_dataLC_Wrong_Block_l1.vi"() -> ("output_Wrong_Block_l1"=w503:i32)  [unwired: 11 in]
              n338 = call "myRIO_BRig_RT_dataLC_Wrong_Trial_l1.vi"() -> ("output_Wrong_Trial_l1"=w502:i32)  [unwired: 11 in]
              n339 = call "myRIO_BRig_RT_dataLC_Wrong_Probability_l1.vi"() -> ("output_Wrong_Probability_l1"=w501:i32)  [unwired: 11 in]
              n340 = call "myRIO_BRig_RT_dataLC_Selection_OnOff_Switch_l1.vi"() -> ("output_Selection_OnOff_Switch_l1"=w496:i32)  [unwired: 11 in]
              n341 = call "myRIO_BRig_RT_dataLC_Selection_Tdelay_Switch_l1.vi"() -> ("output_Selection_Tdelay_Switch_l1"=w495:i32)  [unwired: 11 in]
              n342 = call "myRIO_BRig_RT_dataLC_Selection_Block_Switch_l1.vi"() -> ("output_Selection_Block_Switch_l1"=w494:i32)  [unwired: 11 in]
              n343 = call "myRIO_BRig_RT_dataLC_Selection_Count_Switch_l1.vi"() -> ("output_Selection_Count_Switch_l1"=w493:i32)  [unwired: 11 in]
              n344 = call "myRIO_BRig_RT_dataLC_Selection_Probability_Switch_l1.vi"() -> ("output_Selection_Probability_Switch_l1"=w492:i32)  [unwired: 11 in]
              n345 = call "myRIO_BRig_RT_dataLC_Selection_OnOff_NS_l1.vi"() -> ("output_Selection_OnOff_NS_l1"=w491:i32)  [unwired: 11 in]
              n346 = call "myRIO_BRig_RT_dataLC_Selection_Tdelay_NS_l1.vi"() -> ("output_Selection_Tdelay_NS_l1"=w490:i32)  [unwired: 11 in]
              n347 = call "myRIO_BRig_RT_dataLC_Selection_Block_NS_l1.vi"() -> ("output_Selection_Block_NS_l1"=w489:i32)  [unwired: 11 in]
              n348 = call "myRIO_BRig_RT_dataLC_Selection_Count_NS_l1.vi"() -> ("output_Selection_Count_NS_l1"=w488:i32)  [unwired: 11 in]
              n349 = call "myRIO_BRig_RT_dataLC_Selection_Probability_NS_l1.vi"() -> ("output_Selection_Probability_NS_l1"=w487:i32)  [unwired: 11 in]
              n350 = Index Array(array=w517, index #1=w516, index #2=w515, index #3=w514, index #4=w513, index #5=w512, index #6=w505, index #7=w504, index #8=w503, index #9=w502, index #10=w501, index #11=w496, index #12=w495, index #13=w494, index #14=w493, index #15=w492, index #16=w491, index #17=w490, index #18=w489, index #19=w488, index #20=w487) -> (element #1=w511:u16, element #2=w510:u16, element #3=w509:u16, element #4=w508:u16, element #5=w507:u16, element #6=w506:u16, element #7=w500:u16, element #8=w499:u16, element #9=w498:u16, element #10=w497:u16, element #11=w484:u16, element #12=w483:u16, element #13=w482:u16, element #14=w481:u16, element #15=w480:u16, element #16=w479:u16, element #17=w478:u16, element #18=w477:u16, element #19=w476:u16, element #20=w475:u16)
              n351 = Not Equal To 0?(x=w511) -> (x != 0?=w519:bool)
              n352 = Not Equal To 0?(x=w506) -> (x != 0?=w518:bool)
              n353 = Not Equal To 0?(x=w484) -> (x != 0?=w486:bool)
              n354 = Not Equal To 0?(x=w479) -> (x != 0?=w485:bool)
              n355 = local write "LC_Reward_OnOff_l1"(w519) -> ()
              n356 = local write "LC_Reward_Tdelay_l1"(w510) -> ()
              n357 = local write "LC_Reward_Block_l1"(w509) -> ()
              n358 = local write "LC_Reward_Trial_l1"(w508) -> ()
              n359 = local write "LC_Reward_Probability_l1"(w507) -> ()
              n360 = local write "LC_Wrong_OnOff_l1"(w518) -> ()
              n361 = local write "LC_Wrong_Tdelay_l1"(w500) -> ()
              n362 = local write "LC_Wrong_Block_l1"(w499) -> ()
              n363 = local write "LC_Wrong_Trial_l1"(w498) -> ()
              n364 = local write "LC_Wrong_Probability_l1"(w497) -> ()
              n365 = local write "LC_Sel_OnOff_Switch_l1"(w486) -> ()
              n366 = local write "LC_Sel_Tdelay_Switch_l1"(w483) -> ()
              n367 = local write "LC_Sel_Block_Switch_l1"(w482) -> ()
              n368 = local write "LC_Sel_Count_Switch_l1"(w481) -> ()
              n369 = local write "LC_Sel_Probability_Switch_l1"(w480) -> ()
              n370 = local write "LC_Sel_OnOff_NS_l1"(w485) -> ()
              n371 = local write "LC_Sel_Tdelay_NS_l1"(w478) -> ()
              n372 = local write "LC_Sel_Block_NS_l1"(w477) -> ()
              n373 = local write "LC_Sel_Count_NS_l1"(w476) -> ()
              n374 = local write "LC_Sel_Probability_NS_l1"(w475) -> ()
            }
            frame "UploadSettings_dataLC_4" {
              # "Count"
              # "Tdelay"
              # "Prob"
              # "OnOff"
              # "Block"
              # "Selection NonSwitch"
              # "Count"
              # "Tdelay"
              # "Prob"
              # "OnOff"
              # "Block"
              # "Selection Switch"
              # "Trial"
              # "Tdelay"
              # "Prob"
              # "OnOff"
              # "Block"
              # "Wrong"
              # "Reward"
              # "Trial"
              # "Tdelay"
              # "Prob"
              # "OnOff"
              # "Block"
              n375 = call "myRIO_BRig_RT_dataLC_Reward_OnOff_l2.vi"() -> ("output_Reward_OnOff_l2"=w527:i32)  [unwired: 11 in]
              n376 = call "myRIO_BRig_RT_dataLC_Reward_Tdelay_l2.vi"() -> ("output_Reward_Tdelay_l2"=w528:i32)  [unwired: 11 in]
              n377 = call "myRIO_BRig_RT_dataLC_Reward_Block_l2.vi"() -> ("output_Reward_Block_l2"=w529:i32)  [unwired: 11 in]
              n378 = call "myRIO_BRig_RT_dataLC_Reward_Trial_l2.vi"() -> ("output_Reward_Trial_l2"=w530:i32)  [unwired: 11 in]
              n379 = call "myRIO_BRig_RT_dataLC_Reward_Probability_l2.vi"() -> ("output_Reward_Probability_l2"=w531:i32)  [unwired: 11 in]
              n380 = call "myRIO_BRig_RT_dataLC_Wrong_OnOff_l2.vi"() -> ("output_Wrong_OnOff_l2"=w522:i32)  [unwired: 11 in]
              n381 = call "myRIO_BRig_RT_dataLC_Wrong_Tdelay_l2.vi"() -> ("output_Wrong_Tdelay_l2"=w523:i32)  [unwired: 11 in]
              n382 = call "myRIO_BRig_RT_dataLC_Wrong_Block_l2.vi"() -> ("output_Wrong_Block_l2"=w524:i32)  [unwired: 11 in]
              n383 = call "myRIO_BRig_RT_dataLC_Wrong_Trial_l2.vi"() -> ("output_Wrong_Trial_l2"=w525:i32)  [unwired: 11 in]
              n384 = call "myRIO_BRig_RT_dataLC_Wrong_Probability_l2.vi"() -> ("output_Wrong_Probability_l2"=w526:i32)  [unwired: 11 in]
              n385 = call "myRIO_BRig_RT_dataLC_Selection_OnOff_Switch_l2.vi"() -> ("output_Selection_OnOff_Switch_l2"=w537:i32)  [unwired: 11 in]
              n386 = call "myRIO_BRig_RT_dataLC_Selection_Tdelay_Switch_l2.vi"() -> ("output_Selection_Tdelay_Switch_l2"=w538:i32)  [unwired: 11 in]
              n387 = call "myRIO_BRig_RT_dataLC_Selection_Block_Switch_l2.vi"() -> ("output_Selection_Block_Switch_l2"=w539:i32)  [unwired: 11 in]
              n388 = call "myRIO_BRig_RT_dataLC_Selection_Count_Switch_l2.vi"() -> ("output_Selection_Count_Switch_l2"=w540:i32)  [unwired: 11 in]
              n389 = call "myRIO_BRig_RT_dataLC_Selection_Probability_Switch_l2.vi"() -> ("output_Selection_Probability_Switch_l1"=w541:i32)  [unwired: 11 in]
              n390 = call "myRIO_BRig_RT_dataLC_Selection_OnOff_NS_l2.vi"() -> ("output_Selection_OnOff_NS_l2"=w532:i32)  [unwired: 11 in]
              n391 = call "myRIO_BRig_RT_dataLC_Selection_Tdelay_NS_l2.vi"() -> ("output_Selection_Tdelay_NS_l2"=w533:i32)  [unwired: 11 in]
              n392 = call "myRIO_BRig_RT_dataLC_Selection_Block_NS_l2.vi"() -> ("output_Selection_Block_NS_l2"=w534:i32)  [unwired: 11 in]
              n393 = call "myRIO_BRig_RT_dataLC_Selection_Count_NS_l2.vi"() -> ("output_Selection_Count_NS_l2"=w535:i32)  [unwired: 11 in]
              n394 = call "myRIO_BRig_RT_dataLC_Selection_Probability_NS_l2.vi"() -> ("output_Selection_Probability_NS_l2"=w536:i32)  [unwired: 11 in]
              n395 = Index Array(array=w564, index #1=w527, index #2=w528, index #3=w529, index #4=w530, index #5=w531, index #6=w522, index #7=w523, index #8=w524, index #9=w525, index #10=w526, index #11=w537, index #12=w538, index #13=w539, index #14=w540, index #15=w541, index #16=w532, index #17=w533, index #18=w534, index #19=w535, index #20=w536) -> (element #1=w563:u16, element #2=w562:u16, element #3=w561:u16, element #4=w560:u16, element #5=w559:u16, element #6=w558:u16, element #7=w557:u16, element #8=w556:u16, element #9=w555:u16, element #10=w554:u16, element #11=w551:u16, element #12=w550:u16, element #13=w549:u16, element #14=w548:u16, element #15=w547:u16, element #16=w546:u16, element #17=w545:u16, element #18=w544:u16, element #19=w543:u16, element #20=w542:u16)
              n396 = Not Equal To 0?(x=w563) -> (x != 0?=w566:bool)
              n397 = Not Equal To 0?(x=w558) -> (x != 0?=w565:bool)
              n398 = Not Equal To 0?(x=w551) -> (x != 0?=w553:bool)
              n399 = Not Equal To 0?(x=w546) -> (x != 0?=w552:bool)
              n400 = local write "LC_Reward_OnOff_l2"(w566) -> ()
              n401 = local write "LC_Reward_Tdelay_l2"(w562) -> ()
              n402 = local write "LC_Reward_Block_l2"(w561) -> ()
              n403 = local write "LC_Reward_Trial_l2"(w560) -> ()
              n404 = local write "LC_Reward_Probability_l2"(w559) -> ()
              n405 = local write "LC_Wrong_OnOff_l2"(w565) -> ()
              n406 = local write "LC_Wrong_Tdelay_l2"(w557) -> ()
              n407 = local write "LC_Wrong_Block_l2"(w556) -> ()
              n408 = local write "LC_Wrong_Trial_l2"(w555) -> ()
              n409 = local write "LC_Wrong_Probability_l2"(w554) -> ()
              n410 = local write "LC_Sel_OnOff_Switch_l2"(w553) -> ()
              n411 = local write "LC_Sel_Tdelay_Switch_l2"(w550) -> ()
              n412 = local write "LC_Sel_Block_Switch_l2"(w549) -> ()
              n413 = local write "LC_Sel_Count_Switch_l2"(w548) -> ()
              n414 = local write "LC_Sel_Probability_Switch_l2"(w547) -> ()
              n415 = local write "LC_Sel_OnOff_NS_l2"(w552) -> ()
              n416 = local write "LC_Sel_Tdelay_NS_l2"(w545) -> ()
              n417 = local write "LC_Sel_Block_NS_l2"(w544) -> ()
              n418 = local write "LC_Sel_Count_NS_l2"(w543) -> ()
              n419 = local write "LC_Sel_Probability_NS_l2"(w542) -> ()
            }
            frame "UploadSettings_dataMTrig_1" {
              # "Tdelay_R"
              # "Tdelay_L"
              # "Tcycle_R"
              # "Tcycle_L"
              # "RewCalib_nCycle_R"
              # "RewCalib_nCycle_L"
              # "Solenoid"
              # "Laser_Tcycle"
              n420 = call "myRIO_BRig_RT_dataMTrig_Laser_Tcycle.vi"() -> ("output_Laser_Tcycle"=w576:i32)  [unwired: 11 in]
              n421 = call "myRIO_BRig_RT_dataMTrig_Solenoid_RewCalib_nCycle__L.vi"() -> ("output_Solenoid_RewCalib_nCycle__L"=w575:i32)  [unwired: 11 in]
              n422 = call "myRIO_BRig_RT_dataMTrig_Solenoid_RewCalib_nCycle__R.vi"() -> ("output_Solenoid_RewCalib_nCycle__R"=w574:i32)  [unwired: 11 in]
              n423 = call "myRIO_BRig_RT_dataMTrig_Solenoid_Tdelay__L.vi"() -> ("output_Solenoid_Tdelay__L"=w571:i32)  [unwired: 11 in]
              n424 = call "myRIO_BRig_RT_dataMTrig_Solenoid_Tdelay__R.vi"() -> ("output_Solenoid_Tdelay__R"=w570:i32)  [unwired: 11 in]
              n425 = call "myRIO_BRig_RT_dataMTrig_Solenoid_Tcycle__L.vi"() -> ("output_Solenoid_Tcycle__L"=w573:i32)  [unwired: 11 in]
              n426 = call "myRIO_BRig_RT_dataMTrig_Solenoid_Tcycle__R.vi"() -> ("output_Solenoid_Tcycle__R"=w572:i32)  [unwired: 11 in]
              n427 = Index Array(array=w569, index #1=w576, index #2=w575, index #3=w574, index #4=w573, index #5=w572, index #6=w571, index #7=w570) -> (element #1=w583:u16, element #2=w582:u16, element #3=w581:u16, element #4=w580:u16, element #5=w579:u16, element #6=w578:u16, element #7=w577:u16)
              n428 = Replace Array Subset(array=w585, new element #1=w583, index #1=w576, new element #2=w582, index #2=w575, new element #3=w581, index #3=w574, new element #4=w580, index #4=w573, new element #5=w579, index #5=w572, new element #6=w578, index #6=w571, new element #7=w577, index #7=w570) -> (w584:u16[])
              n429 = local write "MTrig_Solenoid_Tcycle__L"(w580) -> ()
              n430 = local write "MTrig_Solenoid_Tcycle__R"(w579) -> ()
              n431 = local write "MTrig_Laser_Tcycle"(w583) -> ()
            }
            frame "Idle" {
              # "To ensure timing, we split the\nidle state into 4 phases"
              # "Laser_Tcycle"
              # "Audio_Tcycle_R"
              # "Audio_Tcycle_L"
              n432 = local read "Laser_power_min_l1"() -> (w591:dbl)
              n433 = local read "Laser_power_min_l2"() -> (w589:dbl)
              n434 = local read "Audio_Amp__R"() -> (w593:u16)
              n435 = local read "Audio_Amp__L"() -> (w595:u16)
              n436 = local read "Audio_Freq__R"() -> (w592:u8)
              n437 = local read "Audio_Freq__L"() -> (w594:u8)
              n438 = Select(t=myRIO_BRig_RT__Case_NonExp_stateList."SendData" ("Enum"), s="SendData", f=myRIO_BRig_RT__Case_NonExp_stateList."Idle_2" ("Enum")) -> (s? t:f=w600:T1)
              n439 = call "myRIO__convert__Voltage_to_FPGAvalue.vi"("input_voltage"=w591) -> ("output_PortC"=w590:i16)  [unwired: 9 in, 1 out]
              n440 = call "myRIO__convert__Voltage_to_FPGAvalue.vi"("input_voltage"=w589) -> ("output_PortC"=w588:i16)  [unwired: 9 in, 1 out]
              n441 = Select(t=myRIO_BRig_RT__Case_NonExp_stateList."TestConnection" ("Enum"), s="TestConnection", f=w600) -> (s? t:f=w604:T1)
              n442 = xnode "Read/Write Control"("FPGA VI Reference In"=w597, "error in"=w596, "audioAmp_L"=w595, "audioFreq_L_kHz"=w594, "audioAmp_R"=w593, "audioFreq_R_kHz"=w592, "AnaOut_0"=w590, "AnaOut_1"=w588) -> ("error out"=w587:errorcluster)  [unwired: 1 out]
              n443 = local write "error out"(w587) -> ()
              n444 = call "myRIO_BRig_RT_dataMTrig_Audio_Tcycle__L.vi"() -> ("output_Audio_Tcycle__L"=w611:i32)  [unwired: 11 in]
              n445 = call "myRIO_BRig_RT_dataMTrig_Audio_Tcycle__R.vi"() -> ("output_Audio_Tcycle__R"=w610:i32)  [unwired: 11 in]
              n446 = call "myRIO_BRig_RT_dataMTrig_Laser_Tcycle.vi"() -> ("output_Laser_Tcycle"=w609:i32)  [unwired: 11 in]
              n447 = local read "Tcycle_Cue_Audio_min"() -> (w599:u16)
              n448 = local read "MTrig_Laser_Tcycle"() -> (w598:u16)
              n449 = Replace Array Subset(array=w607, new element #1=w599, index #1=w611, new element #2=w599, index #2=w610, new element #3=w598, index #3=w609) -> (w608:u16[])
            }
            frame "Idle_2" {
              w613 = u16 0 ("t")
              # "To ensure timing, we split the\nidle state into 4 phases"
              # "Ncycles"
              # "Ncycles"
              # "RewCalib"
              # "RewCalib"
              # "Solenoid R"
              # "Solenoid L"
              n450 = call "myRIO_BRig_RT_dataMTrig_Solenoid_RewCalib_OnOff__L.vi"() -> ("output_Solenoid_RewCalib_OnOff__L"=w643:i32)  [unwired: 11 in]
              n451 = call "myRIO_BRig_RT_dataMTrig_Solenoid_N__L.vi"() -> ("output_Solenoid_N__L"=w631:i32)  [unwired: 11 in]
              n452 = call "myRIO_BRig_RT_dataMTrig_Solenoid_RewCalib_OnOff__R.vi"() -> ("output_Solenoid_RewCalib_OnOff__R"=w628:i32)  [unwired: 11 in]
              n453 = call "myRIO_BRig_RT_dataMTrig_Solenoid_N__R.vi"() -> ("output_Solenoid_N__R"=w627:i32)  [unwired: 11 in]
              n454 = Index Array(array=w634, index #1=w643, index #2=w631, index #3=w628, index #4=w627) -> (element #1=w630:u16, element #2=w625:u16, element #3=w626:u16, element #4=w624:u16)
              n455 = local read "RewCalib_Trig_L"() -> (w623:bool)
              n456 = local read "RewCalib_Trig_R"() -> (w622:bool)
              n457 = Equal To 0?(x=w625) -> (x = 0?=w633:bool)
              n458 = Equal To 0?(x=w624) -> (x = 0?=w632:bool)
              n459 = Not Equal To 0?(x=w626) -> (x != 0?=w644:bool)
              n460 = Not Equal To 0?(x=w630) -> (x != 0?=w645:bool)
              n461 = And(x=w633, y=w632) -> (x .and. y?=w637:bool)
              n462 = Or(x=w623, y=w622) -> (x .or. y?=w638:bool)
              n463 = Not Exclusive Or(1:w645, 2:w623) -> (0:w640:bool)
              n464 = Not Exclusive Or(1:w644, 2:w622) -> (0:w642:bool)
              n465 = And(x=w638, y=w637) -> (x .and. y?=w620:bool)
              n466 = Not(x=w640) -> (.not. x?=w639:bool)
              n467 = Not(x=w642) -> (.not. x?=w641:bool)
              n468 = Or(x=w639, y=w641) -> (x .or. y?=w621:bool)
              n469 = Or(x=w620, y=w621) -> (x .or. y?=w636:bool)
              n470 = local read "count_warmup_R"() -> (w612:u16)
              n471 = local read "count_warmup_L"() -> (w617:u16)
              n472 = Select(t=myRIO_BRig_RT__Case_NonExp_stateList."RewardCalibration_pre" ("Enum"), s=w636, f=myRIO_BRig_RT__Case_NonExp_stateList."Idle_3" ("Enum")) -> (s? t:f=w619:T1)
              n473 = Select(t=w613, s="count_warmup_L_reset", f=w617) -> (s? t:f=→"count_warmup_L":u16)
              n474 = Select(t=w613, s="count_warmup_R_reset", f=w612) -> (s? t:f=→"count_warmup_R":u16)
            }
            frame "Idle_3" {
              n475 = local read "MTrig_Laser_Switch"() -> (w660:bool)
              n476 = case shown="False" w660 {
                tunnel: "LR_reward_Event" -> [w672 w676]
                tunnel: "LR_wrong_Event" -> [w671 w675]
                tunnel: "LR_reward_Laser" -> [w670 w674]
                tunnel: "LR_wrong_Laser" -> [w669 w673]
                tunnel: [w672 _] -> w655
                tunnel: [w671 _] -> w654
                tunnel: [w670 _] -> w653
                tunnel: [w669 _] -> w652
                tunnel: [_ w676] -> w651
                tunnel: [_ w675] -> w650
                tunnel: [_ w674] -> w649
                tunnel: [_ w673] -> w648
                frame False {
                }
                frame True {
                }
              }
              n477 = xnode "Read/Write Control"("FPGA VI Reference In"=w668, "error in"=w667, "Left(F)_or_Right(T)"="Left(F)_or_Right(T)", "SelectionState"="SelectionState", "ignoreWrong"="ignoreWrong", "LR_reward_Event_l1"=w655, "LR_wrong_Event_l1"=w654, "LR_reward_Laser_l1"=w653, "LR_wrong_Laser_l1"=w652, "LR_reward_Event_l2"=w651, "LR_wrong_Event_l2"=w650, "LR_reward_Laser_l2"=w649, "LR_wrong_laser_l2"=w648) -> ("error out"=→"error out 6":errorcluster, "SelectReward"=→"SelectReward":bool, "SelectWrong"=→"SelectWrong":bool)  [unwired: 1 out]
            }
            frame "Idle_4" {
              n478 = local read "Laser_Tshutter_l1"() -> (w695:dbl)
              n479 = local read "Laser_duration_l1"() -> (w694:u16)
              n480 = local read "Laser_Tshutter_l2"() -> (w691:dbl)
              n481 = local read "Laser_duration_l2"() -> (w690:u16)
              n482 = local read "Laser_Tpeak_l1"() -> (w697:dbl)
              n483 = local read "Laser_Tpeak_l2"() -> (w693:dbl)
              n484 = local read "CueLed_Tpeak"() -> (w688:dbl)
              n485 = local read "Laser_Freq_l1"() -> (w696:dbl)
              n486 = local read "Laser_Freq_l2"() -> (w692:dbl)
              n487 = local read "CueLed_Freq"() -> (w687:dbl)
              n488 = local read "FPGA_count2ms"() -> (w689:dbl)
              n489 = To Unsigned Word Integer(number=w689) -> (unsigned 16bit integer=w698:u16)
              n490 = call "myRIO_BRig_RT__calc_laser_FPGA_N.vi"("input_FPGA_ms2count"=w689, "input_Tpeak"=w697, "input_Freq"=w696, "input_Tshutter"=w695, "input_duration"=w694) -> ("output_laser_Npeak"=w686:u32, "output_laser_Nvalley"=w684:u32, "output_laser_Nshutter"=w682:u32, "output_laser_Nduration"=w680:u32)  [unwired: 6 in, 1 out]
              n491 = call "myRIO_BRig_RT__calc_laser_FPGA_N.vi"("input_FPGA_ms2count"=w689, "input_Tpeak"=w693, "input_Freq"=w692, "input_Tshutter"=w691, "input_duration"=w690) -> ("output_laser_Npeak"=w685:u32, "output_laser_Nvalley"=w683:u32, "output_laser_Nshutter"=w681:u32, "output_laser_Nduration"=w679:u32)  [unwired: 6 in, 1 out]
              n492 = call "myRIO_BRig_RT__calc_laser_FPGA_N__CueLed.vi"("input_FPGA_ms2count"=w689, "input_Tpeak"=w688, "input_Freq"=w687) -> ("output_laser_Npeak"=w678:u32, "output_laser_Nvalley"=w677:u32)  [unwired: 11 in]
              n493 = xnode "Read/Write Control"("FPGA VI Reference In"=w703, "error in"=w702, "k1__counter_per_ms"=w698, "LC_nPeak_l1"=w686, "LC_nPeak_l2"=w685, "LC_nValley_l1"=w684, "LC_nValley_l2"=w683, "LC_nShutter_l1"=w682, "LC_nShutter_l2"=w681, "LR_reward_nTotal_l1"=w680, "LR_wrong_nTotal_l1"=w680, "LR_reward_nTotal_l2"=w679, "LR_wrong_nTotal_l2"=w679, "CueLed_nPeak"=w678, "CueLed_nValley"=w677) -> ("error out"=w699:errorcluster)  [unwired: 1 out]
              n494 = local write "error out"(w699) -> ()
            }
            frame "Idle_5" {
              w725 = u8 0 ("f")
              # "To ensure timing, we split the\nidle state into 4 phases"
              n495 = local read "MTrig_Solenoid_trig__L"() -> (w716:bool)
              n496 = local read "MTrig_Solenoid_trig__R"() -> (w726:bool)
              n497 = local read "warmupType"() -> (w709:u8)
              n498 = local read "warmup"() -> (w718:bool)
              n499 = Not Equal To 0?(x=w709) -> (x != 0?=w708:bool)
              n500 = Not(x=w708) -> (.not. x?=w719:bool)
              n501 = Select(t=u8 1, s=w716, f=w725) -> (s? t:f=w724:u8)
              n502 = Select(t=u8 2, s=w726, f=w725) -> (s? t:f=w723:u8)
              n503 = And(x=w718, y=w719) -> (x .and. y?=w717:bool)
              n504 = And(x=w718, y=w708) -> (x .and. y?=w712:bool)
              n505 = Add(x=w724, y=w723) -> (x+y=w722:u8)
              n506 = case shown="3" w722 {
                tunnel: w721 -> [w729 w733 w766 w797]
                tunnel: [w729 w732 w765 w796] -> w720
                tunnel: w717 -> [_ w731 w764 w795]
                tunnel: [_ TRUE TRUE TRUE] -> w714
                frame 0, Default {
                }
                frame 1 {
                  n507 = case shown="False" w731 {
                    tunnel: w733 -> [w746 w761]
                    tunnel: [w745 w760] -> w732
                    frame True {
                      # "Audio_L"
                      # "Solenoid_L"
                      n508 = call "myRIO_BRig_RT_dataMTrig_Solenoid_N__L.vi"() -> ("output_Solenoid_N__L"=w743:i32)  [unwired: 11 in]
                      n509 = call "myRIO_BRig_RT_dataMTrig_Audio_N__L.vi"() -> ("output_Audio_N__L"=w741:i32)  [unwired: 11 in]
                      n510 = call "myRIO_BRig_RT_dataMTrig_Audio_N__R.vi"() -> ("output_Audio_N__R"=w736:i32)  [unwired: 11 in]
                      n511 = local read "sp_LeftSpout"() -> (w740:u16)
                      n512 = Index Array(array=w746, index #1=w743, index #2=w741, index #3=w736) -> (element #1=w744:u16, element #2=w739:u16, element #3=w738:u16)
                      n513 = Increment(x=w744) -> (x+1=w742:u16)
                      n514 = case shown="2" w740 {
                        tunnel: w739 -> [w749 w752 w754]
                        tunnel: w738 -> [w747 w751 w756]
                        tunnel: [w748 w752 w753] -> w737
                        tunnel: [w747 w750 w755] -> w735
                        frame 0, Default {
                          n515 = Increment(x=w749) -> (x+1=w748:u16)
                        }
                        frame 1 {
                          n516 = Increment(x=w751) -> (x+1=w750:u16)
                        }
                        frame 2 {
                          n517 = Increment(x=w756) -> (x+1=w755:u16)
                          n518 = Increment(x=w754) -> (x+1=w753:u16)
                        }
                      }
                      n519 = Replace Array Subset(array=w746, new element #1=w742, index #1=w743, new element #2=w737, index #2=w741, new element #3=w735, index #3=w736) -> (w745:u16[])
                    }
                    frame False {
                      # "Solenoid_L"
                      n520 = call "myRIO_BRig_RT_dataMTrig_Solenoid_N__L.vi"() -> ("output_Solenoid_N__L"=w758:i32)  [unwired: 11 in]
                      n521 = Index Array(array=w761, index=w758) -> (element=w759:u16)
                      n522 = Increment(x=w759) -> (x+1=w757:u16)
                      n523 = Replace Array Subset(array=w761, new element=w757, index=w758) -> (w760:u16[])
                    }
                  }
                  n524 = local write "MTrig_Solenoid_trig__L"(FALSE) -> ()
                }
                frame 2 {
                  n525 = case shown="True" w764 {
                    tunnel: w766 -> [w778 w793]
                    tunnel: [w777 w792] -> w765
                    frame True {
                      # "Solenoid_R"
                      n526 = call "myRIO_BRig_RT_dataMTrig_Solenoid_N__R.vi"() -> ("output_Solenoid_N__R"=w767:i32)  [unwired: 11 in]
                      n527 = call "myRIO_BRig_RT_dataMTrig_Audio_N__L.vi"() -> ("output_Audio_N__L"=w774:i32)  [unwired: 11 in]
                      n528 = call "myRIO_BRig_RT_dataMTrig_Audio_N__R.vi"() -> ("output_Audio_N__R"=w769:i32)  [unwired: 11 in]
                      n529 = local read "sp_RightSpout"() -> (w773:u16)
                      n530 = Index Array(array=w778, index #1=w767, index #2=w774, index #3=w769) -> (element #1=w776:u16, element #2=w772:u16, element #3=w771:u16)
                      n531 = Increment(x=w776) -> (x+1=w775:u16)
                      n532 = case shown="2" w773 {
                        tunnel: w772 -> [w781 w784 w786]
                        tunnel: w771 -> [w779 w783 w788]
                        tunnel: [w780 w784 w785] -> w770
                        tunnel: [w779 w782 w787] -> w768
                        frame 0, Default {
                          n533 = Increment(x=w781) -> (x+1=w780:u16)
                        }
                        frame 1 {
                          n534 = Increment(x=w783) -> (x+1=w782:u16)
                        }
                        frame 2 {
                          n535 = Increment(x=w788) -> (x+1=w787:u16)
                          n536 = Increment(x=w786) -> (x+1=w785:u16)
                        }
                      }
                      n537 = Replace Array Subset(array=w778, new element #1=w775, index #1=w767, new element #2=w770, index #2=w774, new element #3=w768, index #3=w769) -> (w777:u16[])
                    }
                    frame False {
                      # "Solenoid_R"
                      n538 = call "myRIO_BRig_RT_dataMTrig_Solenoid_N__R.vi"() -> ("output_Solenoid_N__R"=w789:i32)  [unwired: 11 in]
                      n539 = Index Array(array=w793, index=w789) -> (element=w791:u16)
                      n540 = Increment(x=w791) -> (x+1=w790:u16)
                      n541 = Replace Array Subset(array=w793, new element=w790, index=w789) -> (w792:u16[])
                    }
                  }
                  n542 = local write "MTrig_Solenoid_trig__R"(FALSE) -> ()
                }
                frame 3 {
                  w798 = FALSE
                  n543 = case shown="True" w795 {
                    tunnel: w797 -> [w812 w820]
                    tunnel: [w811 w819] -> w796
                    frame True {
                      # "Audio_R"
                      # "Solenoid_R"
                      # "Audio_L"
                      # "Solenoid_L"
                      n544 = call "myRIO_BRig_RT_dataMTrig_Solenoid_N__L.vi"() -> ("output_Solenoid_N__L"=w806:i32)  [unwired: 11 in]
                      n545 = call "myRIO_BRig_RT_dataMTrig_Audio_N__L.vi"() -> ("output_Audio_N__L"=w804:i32)  [unwired: 11 in]
                      n546 = call "myRIO_BRig_RT_dataMTrig_Solenoid_N__R.vi"() -> ("output_Solenoid_N__R"=w802:i32)  [unwired: 11 in]
                      n547 = call "myRIO_BRig_RT_dataMTrig_Audio_N__R.vi"() -> ("output_Audio_N__R"=w801:i32)  [unwired: 11 in]
                      n548 = Index Array(array=w812, index #1=w806, index #2=w804, index #3=w802, index #4=w801) -> (element #1=w810:u16, element #2=w809:u16, element #3=w808:u16, element #4=w807:u16)
                      n549 = Increment(x=w807) -> (x+1=w799:u16)
                      n550 = Increment(x=w810) -> (x+1=w805:u16)
                      n551 = Increment(x=w809) -> (x+1=w803:u16)
                      n552 = Increment(x=w808) -> (x+1=w800:u16)
                      n553 = Replace Array Subset(array=w812, new element #1=w805, index #1=w806, new element #2=w803, index #2=w804, new element #3=w800, index #3=w802, new element #4=w799, index #4=w801) -> (w811:u16[])
                    }
                    frame False {
                      # "Solenoid_R"
                      # "Solenoid_L"
                      n554 = call "myRIO_BRig_RT_dataMTrig_Solenoid_N__L.vi"() -> ("output_Solenoid_N__L"=w816:i32)  [unwired: 11 in]
                      n555 = call "myRIO_BRig_RT_dataMTrig_Solenoid_N__R.vi"() -> ("output_Solenoid_N__R"=w813:i32)  [unwired: 11 in]
                      n556 = Index Array(array=w820, index #1=w816, index #2=w813) -> (element #1=w818:u16, element #2=w817:u16)
                      n557 = Increment(x=w818) -> (x+1=w815:u16)
                      n558 = Increment(x=w817) -> (x+1=w814:u16)
                      n559 = Replace Array Subset(array=w820, new element #1=w815, index #1=w816, new element #2=w814, index #2=w813) -> (w819:u16[])
                    }
                  }
                  n560 = local write "MTrig_Solenoid_trig__L"(w798) -> ()
                  n561 = local write "MTrig_Solenoid_trig__R"(w798) -> ()
                }
              }
              n562 = local read "get_countPerMS"() -> (w707:bool)
              n563 = Select(t=myRIO_BRig_RT__Case_NonExp_stateList."Get_FPGA_count_per_ms" ("Enum"), s=w707, f=myRIO_BRig_RT__Case_NonExp_stateList."Idle_6" ("Enum")) -> (s? t:f=w705:T1)
              n564 = Select(t=myRIO_BRig_RT__Case_NonExp_stateList."Cue_pre", s=w712, f=myRIO_BRig_RT__Case_NonExp_stateList."DispenseWater_pre" ("Enum")) -> (s? t:f=w710:T1)
              n565 = Select(t=w710, s=w714, f=w705) -> (s? t:f=w715:T1)
            }
            frame "Idle_6" {
              # "use dataMTrig as it is one of the last to transfer"
              # "To ensure timing, we split the\nidle state into 4 phases"
              n566 = call "myRIO_BRig_RT_comm_webdav_uploadReceived_check_v2,0.vi"("input_dataName"="dataMTrig") -> ("output_Iexist"=w825:bool)  [unwired: 9 in, 1 out]
              n567 = Select(t=myRIO_BRig_RT__Case_NonExp_stateList."UploadSettings_pre" ("Enum"), s=w825, f=myRIO_BRig_RT__Case_NonExp_stateList."Idle") -> (s? t:f=w823:T1)
            }
            frame "Cue_pre" {
              w851 = u16 0 ("new element/subarray")
              # "Right Audio?"
              # "Left Audio?"
              # "Left or Right?"
              # "Cue Audio?"
              # "Ncycle"
              # "count"
              # "Audio_R"
              # "Ncycle"
              # "count"
              # "Audio_L"
              n568 = local read "Cue1Param_CueType_Switch"() -> (w850:u16)
              n569 = case shown="2" w850 {
                tunnel: [TRUE _ w869] -> w849
                frame 0, Default {
                }
                frame 1 {
                }
                frame 2 {
                  n570 = local read "Cue1Param_AudioLed_Probability_Switch"() -> (w871:u16)
                  n571 = call "myRIO__convert__Probability_to_TrueFalse.vi"("input_probability_u16"=w871) -> ("output_TF"=w870:bool)  [unwired: 10 in]
                  n572 = Not(x=w870) -> (.not. x?=w869:bool)
                }
              }
              n573 = call "myRIO_BRig_RT_dataMTrig_Solenoid_N__L.vi"() -> ("output_Solenoid_N__L"=w861:i32)  [unwired: 11 in]
              n574 = call "myRIO_BRig_RT_dataMTrig_Solenoid_N__R.vi"() -> ("output_Solenoid_N__R"=w860:i32)  [unwired: 11 in]
              n575 = Index Array(array=w857, index #1=w861, index #2=w860) -> (element #1=w859:u16, element #2=w858:u16)
              n576 = Not Equal To 0?(x=w859) -> (x != 0?=w845:bool)
              n577 = Not Equal To 0?(x=w858) -> (x != 0?=w844:bool)
              n578 = And(x=w849, y=w845) -> (x .and. y?=w839:bool)
              n579 = And(x=w849, y=w844) -> (x .and. y?=w837:bool)
              n580 = Select(t=myRIO_BRig_RT__Case_NonExp_stateList."Cue", s=w849, f=myRIO_BRig_RT__Case_NonExp_stateList."Cue_LED") -> (s? t:f=w847:T1)
              n581 = local read "sp_RightSpout"() -> (w838:u16)
              n582 = local read "sp_LeftSpout"() -> (w840:u16)
              n583 = case shown="0, Default" w840 {
                tunnel: [w865 _ w867] -> w836
                tunnel: [_ w866 w867] -> w834
                tunnel: w839 -> [w865 w866 w867]
                frame 0, Default {
                }
                frame 1 {
                }
                frame 2 {
                }
              }
              n584 = case shown="0, Default" w838 {
                tunnel: [w862 _ w864] -> w835
                tunnel: [_ w863 w864] -> w833
                tunnel: w837 -> [w862 w863 w864]
                frame 0, Default {
                }
                frame 1 {
                }
                frame 2 {
                }
              }
              n585 = call "myRIO_BRig_RT_dataMTrig_Audio_c__L.vi"() -> ("output_Audio_c__L"=w855:i32)  [unwired: 11 in]
              n586 = call "myRIO_BRig_RT_dataMTrig_Audio_N__L.vi"() -> ("output_Audio_N__L"=w854:i32)  [unwired: 11 in]
              n587 = call "myRIO_BRig_RT_dataMTrig_Audio_c__R.vi"() -> ("output_Audio_c__R"=w853:i32)  [unwired: 11 in]
              n588 = call "myRIO_BRig_RT_dataMTrig_Audio_N__R.vi"() -> ("output_Audio_N__R"=w852:i32)  [unwired: 11 in]
              n589 = Or(x=w836, y=w835) -> (x .or. y?=w832:bool)
              n590 = Boolean To (0,1)(Boolean=w832) -> (0, 1=w830:i16)
              n591 = To Unsigned Word Integer(number=w830) -> (unsigned 16bit integer=w829:u16)
              n592 = Or(x=w834, y=w833) -> (x .or. y?=w831:bool)
              n593 = Boolean To (0,1)(Boolean=w831) -> (0, 1=w828:i16)
              n594 = To Unsigned Word Integer(number=w828) -> (unsigned 16bit integer=w827:u16)
              n595 = Replace Array Subset(array=w857, new element #1=w851, index #1=w855, new element #2=w829, index #2=w854, new element #3=w851, index #3=w853, new element #4=w827, index #4=w852) -> (w856:u16[])
              n596 = Initialize Array(u16 0 ("element"), 1 ("dimension size")) -> (w843:u16[])
            }
            frame "Cue" {
              # "lick did not occur or warmupType==1"
              # "lick occurred?"
              # "Ncycle"
              # "Audio_R"
              # "Ncycle"
              # "Audio_L"
              n597 = local read "warmupType"() -> (w880:u8)
              n598 = Greater?(x=w886, y=w885) -> (0:w889:bool)
              n599 = Greater?(x=w888, y=w887) -> (0:w884:bool)
              n600 = Or(x=w884, y=w889) -> (x .or. y?=w878:bool)
              n601 = Equal?(x=w880, y=u8 1) -> (x = y?=w874:bool)
              n602 = Not(x=w878) -> (.not. x?=w877:bool)
              n603 = call "myRIO_BRig_RT_dataMTrig_Audio_N__L.vi"() -> ("output_Audio_N__L"=w891:i32)  [unwired: 11 in]
              n604 = call "myRIO_BRig_RT_dataMTrig_Audio_N__R.vi"() -> ("output_Audio_N__R"=w890:i32)  [unwired: 11 in]
              n605 = Or(x=w877, y=w874) -> (x .or. y?=w875:bool)
              n606 = case shown="True" w875 {
                tunnel: w891 -> [w897 w915]
                tunnel: w890 -> [w896 w914]
                tunnel: w883 -> [w899 w909]
                tunnel: [w898 w909] -> w882
                tunnel: w881 -> [_ w907]
                tunnel: [myRIO_BRig_RT__Case_NonExp_stateList."Idle" ("t") w906] -> w876
                tunnel: w874 -> [_ w905]
                tunnel: w873 -> [_ w901]
                tunnel: w872 -> [_ w900]
                frame False {
                  w892 = u16 0 ("new element/subarray")
                  # "lick occurred and warmupType==2"
                  n607 = call "myRIO_BRig_RT_dataMTrig_Solenoid_N__R.vi"() -> ("output_Solenoid_N__R"=w893:i32)  [unwired: 11 in]
                  n608 = call "myRIO_BRig_RT_dataMTrig_Solenoid_N__L.vi"() -> ("output_Solenoid_N__L"=w894:i32)  [unwired: 11 in]
                  n609 = Replace Array Subset(array=w899, new element #1=w892, index #1=w897, new element #2=w892, index #2=w896, new element #3=w892, index #3=w894, new element #4=w892, index #4=w893) -> (w898:u16[])
                }
                frame True {
                  n610 = Not(x=w905) -> (.not. x?=w904:bool)
                  n611 = Index Array(array=w909, index #1=w915, index #2=w914) -> (element #1=w913:u16, element #2=w912:u16)
                  n612 = Equal To 0?(x=w913) -> (x = 0?=w911:bool)
                  n613 = Equal To 0?(x=w912) -> (x = 0?=w910:bool)
                  n614 = And(x=w911, y=w910) -> (x .and. y?=w903:bool)
                  n615 = And(x=w903, y=w904) -> (x .and. y?=w902:bool)
                  n616 = case shown="True" w902 {
                    tunnel: w901 -> [_ w923]
                    tunnel: w900 -> [_ w918]
                    frame False {
                    }
                    frame True {
                      n617 = local read "count_warmup_R"() -> (w916:u16)
                      n618 = local read "count_warmup_L"() -> (w921:u16)
                      n619 = Increment(x=w916) -> (x+1=w919:u16)
                      n620 = Increment(x=w921) -> (x+1=w922:u16)
                      n621 = Select(t=w919, s=w918, f=w916) -> (s? t:f=w917:u16)
                      n622 = Select(t=w922, s=w923, f=w921) -> (s? t:f=w920:u16)
                      n623 = local write "count_warmup_R"(w917) -> ()
                      n624 = local write "count_warmup_L"(w920) -> ()
                    }
                  }
                  n625 = Select(t=myRIO_BRig_RT__Case_NonExp_stateList."DispenseWater_pre", s=w903, f=w907) -> (s? t:f=w906:T1)
                }
              }
            }
            frame "Cue_LED" {
              # "lick did not occur or warmupType==1"
              # "lick occurred?"
              n626 = local read "warmupType"() -> (w936:u8)
              n627 = Greater?(x=w942, y=w941) -> (0:w945:bool)
              n628 = Greater?(x=w944, y=w943) -> (0:w940:bool)
              n629 = Or(x=w940, y=w945) -> (x .or. y?=w934:bool)
              n630 = Equal?(x=w936, y=u8 1) -> (x = y?=w930:bool)
              n631 = Not(x=w934) -> (.not. x?=w933:bool)
              n632 = Or(x=w933, y=w930) -> (x .or. y?=w931:bool)
              n633 = case shown="True" w931 {
                tunnel: w939 -> [w952 w972]
                tunnel: [w951 w972] -> w938
                tunnel: w937 -> [_ w958]
                tunnel: [myRIO_BRig_RT__Case_NonExp_stateList."Idle" ("t") w971] -> w932
                tunnel: w930 -> [_ w957]
                tunnel: w929 -> [_ w969]
                tunnel: w928 -> [_ w968]
                tunnel: w927 -> [w946 w967]
                tunnel: [w946 w960] -> w926
                tunnel: w925 -> [_ w955]
                tunnel: w924 -> [_ w954]
                frame False {
                  w947 = u16 0 ("new element/subarray")
                  # "lick occurred and warmupType==2"
                  n634 = call "myRIO_BRig_RT_dataMTrig_Solenoid_N__R.vi"() -> ("output_Solenoid_N__R"=w948:i32)  [unwired: 11 in]
                  n635 = call "myRIO_BRig_RT_dataMTrig_Solenoid_N__L.vi"() -> ("output_Solenoid_N__L"=w949:i32)  [unwired: 11 in]
                  n636 = Replace Array Subset(array=w952, new element #1=w947, new element #2=w947, index #2=w949, new element #3=w947, index #3=w948) -> (w951:u16[])  [unwired: 1 in]
                }
                frame True {
                  w965 = 0 ("index")
                  n637 = local read "Tcycle_Cue_LED_min"() -> (w961:u16)
                  n638 = Index Array(array=w967, index=w965) -> (element=w966:u16)
                  n639 = Increment(x=w966) -> (x+1=w964:u16)
                  n640 = Multiply(x=w964, y=u16 5) -> (x*y=w962:u16)
                  n641 = Replace Array Subset(array=w967, new element=w964, index=w965) -> (w960:u16[])
                  n642 = Less?(x=w962, y=w961) -> (x < y?=w956:bool)
                  n643 = Not Or(1:w957, 2:w956) -> (0:w970:bool)
                  n644 = case shown="True" w970 {
                    tunnel: w969 -> [_ w980]
                    tunnel: w968 -> [_ w975]
                    frame False {
                    }
                    frame True {
                      n645 = local read "count_warmup_R"() -> (w973:u16)
                      n646 = local read "count_warmup_L"() -> (w978:u16)
                      n647 = Increment(x=w973) -> (x+1=w976:u16)
                      n648 = Increment(x=w978) -> (x+1=w979:u16)
                      n649 = Select(t=w976, s=w975, f=w973) -> (s? t:f=w974:u16)
                      n650 = Select(t=w979, s=w980, f=w978) -> (s? t:f=w977:u16)
                      n651 = local write "count_warmup_R"(w974) -> ()
                      n652 = local write "count_warmup_L"(w977) -> ()
                    }
                  }
                  n653 = Select(t=w958, s=w956, f=myRIO_BRig_RT__Case_NonExp_stateList."DispenseWater_pre" ("t")) -> (s? t:f=w971:T1)
                  n654 = xnode "Read/Write Control"("FPGA VI Reference In"=w955, "error in"=w954, "CueLed_Event"=w956) -> ("error out"=w953:errorcluster)  [unwired: 1 out]
                  n655 = local write "error out"(w953) -> ()
                }
              }
            }
            frame "RewardCalibration_pre" {
              (unwired) FALSE
              w981 = FALSE
              w992 = u8 0
              w1008 = u8 0
              # "Are we starting a RewardCalibration?\nOr are we stopping a RewardCalibration?\nOr is a RewardCalibration over?"
              # "RewCalib\nOnOff"
              # "N"
              # "Solenoid R"
              # "RewCalib\nOnOff"
              # "N"
              # "Solenoid L"
              n656 = local read "RewCalib_Trig_L"() -> (w1015:bool)
              n657 = local read "RewCalib_Trig_R"() -> (w984:bool)
              n658 = call "myRIO_BRig_RT_dataMTrig_Solenoid_N__R.vi"() -> ("output_Solenoid_N__R"=w986:i32)  [unwired: 11 in]
              n659 = call "myRIO_BRig_RT_dataMTrig_Solenoid_RewCalib_OnOff__R.vi"() -> ("output_Solenoid_RewCalib_OnOff__R"=w983:i32)  [unwired: 11 in]
              n660 = call "myRIO_BRig_RT_dataMTrig_Solenoid_N__L.vi"() -> ("output_Solenoid_N__L"=w1001:i32)  [unwired: 11 in]
              n661 = call "myRIO_BRig_RT_dataMTrig_Solenoid_RewCalib_OnOff__L.vi"() -> ("output_Solenoid_RewCalib_OnOff__L"=w1002:i32)  [unwired: 11 in]
              n662 = Index Array(array=w985, index #1=w986, index #2=w983) -> (element #1=w996:u16, element #2=w991:u16)
              n663 = Index Array(array=w985, index #1=w1001, index #2=w1002) -> (element #1=w1012:u16, element #2=w1007:u16)
              n664 = Equal To 0?(x=w996) -> (x = 0?=w997:bool)
              n665 = Not Equal To 0?(x=w991) -> (x != 0?=w994:bool)
              n666 = Equal To 0?(x=w1012) -> (x = 0?=w1013:bool)
              n667 = Not Equal To 0?(x=w1007) -> (x != 0?=w1010:bool)
              n668 = local write "MTrig_Solenoid_trig__L"(w981) -> ()
              n669 = local write "MTrig_Solenoid_trig__R"(w981) -> ()
              n670 = Select(t=u8 1, s=w984, f=w992) -> (s? t:f=w988:u8)
              n671 = Select(t=u8 1, s=w1015, f=w1008) -> (s? t:f=w1004:u8)
              n672 = Select(t=u8 2, s=w997, f=w992) -> (s? t:f=w989:u8)
              n673 = Select(t=u8 4, s=w994, f=w992) -> (s? t:f=w990:u8)
              n674 = Select(t=u8 2, s=w1013, f=w1008) -> (s? t:f=w1005:u8)
              n675 = Select(t=u8 4, s=w1010, f=w1008) -> (s? t:f=w1006:u8)
              n676 = Compound Arithmetic op=ADD(w988, w989, w990) -> (w987:u8)
              n677 = Compound Arithmetic op=ADD(w1004, w1005, w1006) -> (w1003:u8)
              n678 = case shown="7" w1003 {
                tunnel: w985 -> [w1045 w1050 w1052 w1057 w1062 w1064 w1067 w1072]
                tunnel: [w1045 w1051 w1052 w1058 w1063 w1064 w1068 w1073] -> w1000
                tunnel: w1002 -> [_ w1048 _ w1055 w1060 _ w1066 w1071]
                tunnel: w1001 -> [_ w1049 _ w1056 w1061 _ _ _]
                frame 0, Default {
                }
                frame 1 {
                  n679 = Replace Array Subset(array=w1050, new element #1=u16 100 ("new element/subarray"), index #1=w1049, new element #2=u16 1 ("new element/subarray"), index #2=w1048) -> (w1051:u16[])
                }
                frame 2 {
                }
                frame 3 {
                  n680 = Replace Array Subset(array=w1057, new element #1=u16 100 ("new element/subarray"), index #1=w1056, new element #2=u16 1 ("new element/subarray"), index #2=w1055) -> (w1058:u16[])
                }
                frame 4 {
                  w1059 = u16 0 ("new element/subarray")
                  n681 = Replace Array Subset(array=w1062, new element #1=w1059, index #1=w1061, new element #2=w1059, index #2=w1060) -> (w1063:u16[])
                }
                frame 5 {
                }
                frame 6 {
                  n682 = Replace Array Subset(array=w1067, new element=u16 0 ("new element/subarray"), index=w1066) -> (w1068:u16[])
                }
                frame 7 {
                  n683 = local write "RewCalib_Trig_L"(FALSE ("RewCalib_Trig_L")) -> ()
                  n684 = Replace Array Subset(array=w1072, new element=u16 0 ("new element/subarray"), index=w1071) -> (w1073:u16[])
                }
              }
              n685 = case shown="7" w987 {
                tunnel: w1000 -> [w1016 w1021 w1023 w1028 w1033 w1035 w1038 w1043]
                tunnel: [w1016 w1022 w1023 w1029 w1034 w1035 w1039 w1044] -> w999
                tunnel: w983 -> [_ w1019 _ w1026 w1031 _ w1037 w1042]
                tunnel: w986 -> [_ w1020 _ w1027 w1032 _ _ _]
                frame 0, Default {
                }
                frame 1 {
                  n686 = Replace Array Subset(array=w1021, new element #1=u16 100 ("new element/subarray"), index #1=w1020, new element #2=u16 1 ("new element/subarray"), index #2=w1019) -> (w1022:u16[])
                }
                frame 2 {
                }
                frame 3 {
                  n687 = Replace Array Subset(array=w1028, new element #1=u16 100 ("new element/subarray"), index #1=w1027, new element #2=u16 1 ("new element/subarray"), index #2=w1026) -> (w1029:u16[])
                }
                frame 4 {
                  w1030 = u16 0 ("new element/subarray")
                  n688 = Replace Array Subset(array=w1033, new element #1=w1030, index #1=w1032, new element #2=w1030, index #2=w1031) -> (w1034:u16[])
                }
                frame 5 {
                }
                frame 6 {
                  n689 = Replace Array Subset(array=w1038, new element=u16 0 ("new element/subarray"), index=w1037) -> (w1039:u16[])
                }
                frame 7 {
                  n690 = local write "RewCalib_Trig_R"(FALSE ("RewCalib_Trig_L")) -> ()
                  n691 = Replace Array Subset(array=w1043, new element=u16 0 ("new element/subarray"), index=w1042) -> (w1044:u16[])
                }
              }
            }
            frame "DispenseWater_pre" {
              w1079 = u16 0 ("t")
              w1122 = u16 0 ("new element/subarray")
              # "just trust me on this one"
              # "RewCalib\nOnOff"
              # "RewCalib\nOnOff"
              # "nCycle"
              # "Solenoid__R"
              # "Tdelay"
              # "delay"
              # "nCycle"
              # "Solenoid__L"
              # "Tdelay"
              # "delay"
              # "Solenoid__R"
              # "count"
              # "Solenoid_Tcycle_R"
              # "Solenoid_Tcycle_L"
              # "Solenoid__L"
              # "count"
              n692 = call "myRIO_BRig_RT_dataMTrig_Solenoid_RewCalib_OnOff__L.vi"() -> ("output_Solenoid_RewCalib_OnOff__L"=w1086:i32)  [unwired: 11 in]
              n693 = call "myRIO_BRig_RT_dataMTrig_Solenoid_N__L.vi"() -> ("output_Solenoid_N__L"=w1077:i32)  [unwired: 11 in]
              n694 = call "myRIO_BRig_RT_dataMTrig_Solenoid_delay__L.vi"() -> ("output_Solenoid_delay__L"=w1120:i32)  [unwired: 11 in]
              n695 = call "myRIO_BRig_RT_dataMTrig_Solenoid_Tdelay__L.vi"() -> ("output_Solenoid_Tdelay__L"=w1119:i32)  [unwired: 11 in]
              n696 = call "myRIO_BRig_RT_dataMTrig_Solenoid_N__R.vi"() -> ("output_Solenoid_N__R"=w1075:i32)  [unwired: 11 in]
              n697 = call "myRIO_BRig_RT_dataMTrig_Solenoid_delay__R.vi"() -> ("output_Solenoid_delay__R"=w1109:i32)  [unwired: 11 in]
              n698 = call "myRIO_BRig_RT_dataMTrig_Solenoid_Tdelay__R.vi"() -> ("output_Solenoid_Tdelay__R"=w1108:i32)  [unwired: 11 in]
              n699 = call "myRIO_BRig_RT_dataMTrig_Solenoid_RewCalib_OnOff__R.vi"() -> ("output_Solenoid_RewCalib_OnOff__R"=w1082:i32)  [unwired: 11 in]
              n700 = Index Array(array=w1121, index #1=w1077, index #2=w1120, index #3=w1119, index #4=w1075, index #5=w1109, index #6=w1108, index #7=w1086, index #8=w1082) -> (element #1=w1078:u16, element #2=w1118:u16, element #3=w1113:u16, element #4=w1081:u16, element #5=w1103:u16, element #6=w1102:u16, element #7=w1087:u16, element #8=w1084:u16)
              n701 = Equal To 0?(x=w1118) -> (x = 0?=w1117:bool)
              n702 = Equal To 0?(x=w1103) -> (x = 0?=w1107:bool)
              n703 = local read "RewCalib_Trig_L"() -> (w1098:bool)
              n704 = local read "RewCalib_Trig_R"() -> (w1093:bool)
              n705 = Not Equal To 0?(x=w1078) -> (x != 0?=w1116:bool)
              n706 = Not Equal To 0?(x=w1081) -> (x != 0?=w1106:bool)
              n707 = local read "MTrig_Solenoid_Tcycle__L"() -> (w1115:u16)
              n708 = local read "MTrig_Solenoid_Tcycle__R"() -> (w1101:u16)
              n709 = Not Equal To 0?(x=w1087) -> (x != 0?=w1097:bool)
              n710 = Not Equal To 0?(x=w1084) -> (x != 0?=w1095:bool)
              n711 = Not(x=w1098) -> (.not. x?=w1096:bool)
              n712 = Not(x=w1093) -> (.not. x?=w1094:bool)
              n713 = And(x=w1097, y=w1096) -> (x .and. y?=w1092:bool)
              n714 = And(x=w1095, y=w1094) -> (x .and. y?=w1091:bool)
              n715 = call "myRIO_BRig_RT_dataMTrig_Solenoid_c__L.vi"() -> ("output_Solenoid_c__L"=w1124:i32)  [unwired: 11 in]
              n716 = call "myRIO_BRig_RT_dataMTrig_Solenoid_c__R.vi"() -> ("output_Solenoid_c__R"=w1123:i32)  [unwired: 11 in]
              n717 = Select(t=w1115, s=w1116, f=u16 0) -> (s? t:f=w1112:u16)
              n718 = Or(x=w1092, y=w1091) -> (x .or. y?=w1080:bool)
              n719 = Select(t=w1101, s=w1106, f=u16 0) -> (s? t:f=w1104:u16)
              n720 = Select(t=w1112, s=w1117, f=w1113) -> (s? t:f=w1110:u16)
              n721 = Select(t=w1104, s=w1107, f=w1102) -> (s? t:f=w1099:u16)
              n722 = call "myRIO_BRig_RT_dataMTrig_Solenoid_Tcycle__L.vi"() -> ("output_Solenoid_Tcycle__L"=w1111:i32)  [unwired: 11 in]
              n723 = call "myRIO_BRig_RT_dataMTrig_Solenoid_Tcycle__R.vi"() -> ("output_Solenoid_Tcycle__R"=w1100:i32)  [unwired: 11 in]
              n724 = Select(t=w1079, s=w1080, f=w1078) -> (s? t:f=w1076:u16)
              n725 = Select(t=w1079, s=w1080, f=w1081) -> (s? t:f=w1074:u16)
              n726 = Select(t=myRIO_BRig_RT__Case_NonExp_stateList."Idle" ("Enum"), s=w1080, f=myRIO_BRig_RT__Case_NonExp_stateList."DispenseWater" ("Enum")) -> (s? t:f=w1088:T1)
              n727 = Select(t=w1079, s=w1080, f=w1087) -> (s? t:f=w1085:u16)
              n728 = Select(t=w1079, s=w1080, f=w1084) -> (s? t:f=w1083:u16)
              n729 = Replace Array Subset(array=w1121, new element #1=w1122, index #1=w1124, new element #2=w1122, index #2=w1123, new element #3=w1110, index #3=w1111, new element #4=w1099, index #4=w1100, new element #5=w1085, index #5=w1086, new element #6=w1083, index #6=w1082, new element #7=w1076, index #7=w1077, new element #8=w1074, index #8=w1075) -> (w1125:u16[])
            }
            frame "DispenseWater" {
              # "D"
              # "C"
              # "B"
              # "A"
              # "(A) Add COUNT and INCREMENT\n(B) Is (A) smaller than Tcycle?\n(C) Are we dispensing water or in the delay phase?\n(D) If (A) is smaller than Tcycle   AND   if we are dispensing water\n      then send TRUE to solenoid"
              # "delay"
              # "Tcycle"
              # "Solenoid__R"
              # "count"
              # "delay"
              # "Tcycle"
              # "Solenoid__L"
              # "count"
              n730 = To Unsigned Word Integer(number=w1152) -> (unsigned 16bit integer=w1134:u16)
              n731 = call "myRIO_BRig_RT_dataMTrig_Solenoid_delay__R.vi"() -> ("output_Solenoid_delay__R"=w1138:i32)  [unwired: 11 in]
              n732 = call "myRIO_BRig_RT_dataMTrig_Solenoid_c__R.vi"() -> ("output_Solenoid_c__R"=w1137:i32)  [unwired: 11 in]
              n733 = call "myRIO_BRig_RT_dataMTrig_Solenoid_Tcycle__R.vi"() -> ("output_Solenoid_Tcycle__R"=w1139:i32)  [unwired: 11 in]
              n734 = call "myRIO_BRig_RT_dataMTrig_Solenoid_delay__L.vi"() -> ("output_Solenoid_delay__L"=w1154:i32)  [unwired: 11 in]
              n735 = call "myRIO_BRig_RT_dataMTrig_Solenoid_c__L.vi"() -> ("output_Solenoid_c__L"=w1146:i32)  [unwired: 11 in]
              n736 = call "myRIO_BRig_RT_dataMTrig_Solenoid_Tcycle__L.vi"() -> ("output_Solenoid_Tcycle__L"=w1155:i32)  [unwired: 11 in]
              n737 = Index Array(array=w1148, index #1=w1146, index #2=w1155, index #3=w1154, index #4=w1137, index #5=w1139, index #6=w1138) -> (element #1=w1153:u16, element #2=w1143:u16, element #3=w1151:u16, element #4=w1133:u16, element #5=w1130:u16, element #6=w1129:u16)
              n738 = Add(x=w1153, y=w1134) -> (x+y=w1144:u16)
              n739 = Add(x=w1133, y=w1134) -> (x+y=w1135:u16)
              n740 = Less?(x=w1144, y=w1143) -> (x < y?=w1127:bool)
              n741 = Equal To 0?(x=w1151) -> (x = 0?=w1150:bool)
              n742 = Less?(x=w1135, y=w1130) -> (x < y?=w1128:bool)
              n743 = Equal To 0?(x=w1129) -> (x = 0?=w1136:bool)
              n744 = And(x=w1127, y=w1150) -> (x .and. y?=w1149:bool)
              n745 = Or(x=w1127, y=w1128) -> (x .or. y?=w1126:bool)
              n746 = And(x=w1128, y=w1136) -> (x .and. y?=w1131:bool)
              n747 = Select(t=w1144, s=w1127, f=w1143) -> (s? t:f=w1145:u16)
              n748 = Select(t=w1135, s=w1128, f=w1130) -> (s? t:f=w1132:u16)
              n749 = Replace Array Subset(array=w1148, new element #1=w1145, index #1=w1146, new element #2=w1132, index #2=w1137) -> (w1147:u16[])
              n750 = Select(t=w1142, s=w1126, f=myRIO_BRig_RT__Case_NonExp_stateList."DispenseWater_post" ("Enum")) -> (s? t:f=w1140:T1)
            }
            frame "DispenseWater_post" {
              # "nCycle"
              # "delay"
              # "Solenoid__R"
              # "nCycle"
              # "delay"
              # "Solenoid__L"
              n751 = call "myRIO_BRig_RT_dataMTrig_Solenoid_N__L.vi"() -> ("output_Solenoid_N__L"=w1172:i32)  [unwired: 11 in]
              n752 = call "myRIO_BRig_RT_dataMTrig_Solenoid_delay__L.vi"() -> ("output_Solenoid_delay__L"=w1171:i32)  [unwired: 11 in]
              n753 = call "myRIO_BRig_RT_dataMTrig_Solenoid_N__R.vi"() -> ("output_Solenoid_N__R"=w1168:i32)  [unwired: 11 in]
              n754 = call "myRIO_BRig_RT_dataMTrig_Solenoid_delay__R.vi"() -> ("output_Solenoid_delay__R"=w1167:i32)  [unwired: 11 in]
              n755 = Index Array(array=w1174, index #1=w1172, index #2=w1171, index #3=w1168, index #4=w1167) -> (element #1=w1176:u16, element #2=w1175:u16, element #3=w1159:u16, element #4=w1161:u16)
              n756 = Not Equal To 0?(x=w1176) -> (x != 0?=w1177:bool)
              n757 = Not Equal To 0?(x=w1159) -> (x != 0?=w1160:bool)
              n758 = case shown="True" w1160 {
                selector: w1160 -> [_ w1181]
                tunnel: w1159 -> [w1179 w1187]
                tunnel: w1161 -> [_ w1188]
                tunnel: [w1179 w1185] -> w1158
                tunnel: [u16 0 w1184] -> w1157
                tunnel: [_ w1181] -> w1156
                frame False {
                }
                frame True {
                  n759 = Equal To 0?(x=w1188) -> (x = 0?=w1180:bool)
                  n760 = Decrement(x=w1187) -> (x-1=w1186:u16)
                  n761 = Select(t=w1186, s=w1180, f=w1187) -> (s? t:f=w1185:u16)
                  n762 = Select(t=u16 1, s=w1180, f=u16 0) -> (s? t:f=w1184:u16)
                }
              }
              n763 = case shown="True" w1177 {
                selector: w1177 -> [_ w1192]
                tunnel: w1176 -> [w1190 w1198]
                tunnel: w1175 -> [_ w1199]
                tunnel: [w1190 w1196] -> w1170
                tunnel: [u16 0 w1195] -> w1169
                tunnel: [_ w1192] -> w1166
                frame False {
                }
                frame True {
                  n764 = Equal To 0?(x=w1199) -> (x = 0?=w1191:bool)
                  n765 = Decrement(x=w1198) -> (x-1=w1197:u16)
                  n766 = Select(t=w1197, s=w1191, f=w1198) -> (s? t:f=w1196:u16)
                  n767 = Select(t=u16 1, s=w1191, f=u16 0) -> (s? t:f=w1195:u16)
                }
              }
              n768 = Or(x=w1166, y=w1156) -> (x .or. y?=w1165:bool)
              n769 = Replace Array Subset(array=w1174, new element #1=w1170, index #1=w1172, new element #2=w1169, index #2=w1171, new element #3=w1158, index #3=w1168, new element #4=w1157, index #4=w1167) -> (w1173:u16[])
              n770 = Select(t=myRIO_BRig_RT__Case_NonExp_stateList."DispenseWater_pre" ("Enum"), s=w1165, f=myRIO_BRig_RT__Case_NonExp_stateList."Idle" ("Enum")) -> (s? t:f=w1162:T1)
            }
            frame "TestConnection" {
              n771 = local read "Host Password"() -> (w1205:string)
              n772 = local read "Host UserName"() -> (w1206:string)
              n773 = call "myRIO_BRig_RT_comm_webdav_testConnect.vi"("input_password"=w1205, "input_username"=w1206) -> ("output_Iconnected"=w1203:bool)  [unwired: 9 in]
              n774 = Select(t="Connection accepted!" ("message"), s=w1203, f="Error!") -> (s? t:f=w1201:string)
              n775 = One Button Dialog(message=w1201) -> ()  [unwired: 1 in, 1 out]
            }
            frame "SendData" {
              n776 = local read "Data Set Prefix"() -> (w1208:string)
              n777 = local read "Host Password"() -> (w1209:string)
              n778 = local read "Host UserName"() -> (w1210:string)
              n779 = call "myRIO_BRig_RT_comm_webdav_sendData_all.vi"("Host Filename Prefix"=w1208, "Host Password"=w1209, "Host UserName"=w1210) -> ()  [unwired: 9 in]
            }
            frame "Get_FPGA_count_per_ms" {
              n780 = case shown="False" w1223 {
                selector: w1223 -> [w1225 _]
                tunnel: w1221 -> [_ w1238]
                tunnel: [w1229 w1238] -> w1220
                tunnel: w1219 -> [w1228 w1236]
                tunnel: w1218 -> [w1227 w1235]
                tunnel: [w1226 w1233] -> w1217
                tunnel: [w1225 w1232] -> w1216
                frame False {
                  n781 = Get Date/Time In Seconds() -> (seconds since 1Jan1904=w1230:timestamp)
                  n782 = xnode "Read/Write Control"("FPGA VI Reference In"=w1228, "error in"=w1227, "timeTrial_trig"=TRUE ("timeTrial")) -> ("error out"=w1226:errorcluster)  [unwired: 1 out]
                  n783 = To Double Precision Float(number=w1230) -> (double precision float=w1229:dbl)
                  n784 = local write "get_countPerMS"(w1225) -> ()
                }
                frame True {
                  w1234 = 1.0
                  n785 = Get Date/Time In Seconds() -> (seconds since 1Jan1904=w1239:timestamp)
                  n786 = To Double Precision Float(number=w1239) -> (double precision float=w1240:dbl)
                  n787 = Subtract(x=w1240, y=w1238) -> (x-y=w1237:dbl)
                  n788 = Less Or Equal?(x=w1234, y=w1237) -> (x <= y?=w1232:bool)
                  n789 = case shown="True" w1232 {
                    tunnel: w1236 -> [_ w1253]
                    tunnel: w1235 -> [w1241 w1252]
                    tunnel: w1234 -> [_ w1243]
                    tunnel: [w1241 w1242] -> w1233
                    frame False {
                    }
                    frame True {
                      n790 = xnode "Read/Write Control"("FPGA VI Reference In"=w1253, "error in"=w1252) -> ("FPGA VI Reference Out"=w1250:refnum<k20>, "error out"=w1249:errorcluster, "timeTrial_count"=w1244:u32)
                      n791 = Multiply(x=w1243, y=1000.0) -> (x*y=w1247:dbl)
                      n792 = To Double Precision Float(number=w1244) -> (double precision float=w1246:dbl)
                      n793 = Divide(x=w1246, y=w1247) -> (x/y=w1248:dbl)
                      n794 = local write "FPGA_count2ms"(w1248) -> ()
                      n795 = xnode "Read/Write Control"("FPGA VI Reference In"=w1250, "error in"=w1249, "timeTrial_trig"=FALSE ("timeTrial")) -> ("error out"=w1242:errorcluster)  [unwired: 1 out]
                    }
                  }
                }
              }
              "error out 5" <- w1217
              n796 = Select(t=myRIO_BRig_RT__Case_NonExp_stateList."Idle" ("Enum"), s=w1216, f=w1214) -> (s? t:f=w1213:T1)
            }
            frame "End" {
            }
          }
          n797 = local read "MTrig_Audio_trig__R"() -> (w89:bool)
          n798 = local read "MTrig_Audio_trig__L"() -> (w90:bool)
          n799 = local read "MTrig_Laser_trig"() -> (w88:bool)
          n800 = Compound Arithmetic op=OR(w90, w89, w88) -> (w87:bool)
          n801 = local read "START"() -> (w113:bool)
          n802 = local read "STOP_abort"() -> (w112:bool)
          n803 = case shown="True" w87 {
            frame False {
            }
            frame True {
              w129 = FALSE
              n804 = local write "MTrig_Audio_trig__R"(w129) -> ()
              n805 = local write "MTrig_Audio_trig__L"(w129) -> ()
              n806 = local write "MTrig_Laser_trig"(w129) -> ()
            }
          }
          n807 = call "myRIO_BRig_RT_dataMTrig_main__v2.vi"("input_dataMTrig"=w116, "input_Audio_trig_L"=w90, "input_Audio_trig_R"=w89, "input_Laser_trig"=w88) -> ("output_dataMTrig"=w115:u16[], "output_Audio_L"=w107:bool, "output_Audio_R"=w108:bool, "output_Laser"=w86:bool)  [unwired: 12 in]
          n808 = Or(x=w113, y=w112) -> (x .or. y?=w111:bool)
          n809 = Select(t=myRIO_BRig_RT__Case_NonExp_stateList."End" ("Enum"), s=w111, f=w110) -> (s? t:f=w109:T1)
          n810 = Not(x="MTrig_Laser_Switch") -> (.not. x?=w83:bool)
          n811 = And(x=w86, y=w83) -> (x .and. y?=w84:bool)
          n812 = And(x=w86, y="MTrig_Laser_Switch") -> (x .and. y?=w85:bool)
          n813 = xnode "Read/Write Control"("FPGA VI Reference In"=w96, "error in"=w95, "A1_SR"=w117, "A3_SL"=w118, "audioTrigger_L"=w107, "audioTrigger_R"=w108, "LC_Laser_l1"=w84, "LC_Laser_l2"=w85) -> ("FPGA VI Reference Out"=w123:refnum<k20>, "error out"=w122:errorcluster)
          n814 = node-c288() -> ()  [unwired: 1 in, 1 out]
          "cState_NonExp" <- w121
        }
        n815 = node-c288(w70) -> ()  [unwired: 1 out]
        n816 = flat-sequence {
          tunnel: w63 -> [w81]
          tunnel: [w81] -> w62
          tunnel: w61 -> [w80]
          tunnel: [w80] -> w60
          frame #0 {
            w79 = FALSE
            n817 = local write "STOP_endBlock"(w79) -> ()
            n818 = local write "STOP_endTrial"(w79) -> ()
          }
        }
      }
      frame True {
        w1265 = u16 0
        w1283 = u8 0
        w1284 = u16 0 ("idxDataBlock")
        w1286 = u16 100 ("new element/subarray")
        w1287 = u16 100 ("new element/subarray")
        w1307 = T6 refnum items=["Session NI_WebDAV"] ("output_hSession")
        w1316 = FALSE
        w1317 = u16 0
        # "dummyState counter"
        # "audio__L\naudio__R"
        # "Audio params"
        # "nRewards"
        # "idxDataBlock"
        # "Solenoid_Tdelay_R"
        # "Solenoid_Tdelay_L"
        # "RewCalib_N__R"
        # "RewCalib_N__L"
        # "Save dataLick to file\nSend file to Host\nSave dataMTrig\nSend file to Host\nDisconnect"
        # "dataTrial"
        # "dataTrial"
        # "Solenoid_Tcycle_R"
        # "Solenoid_Tcycle_L"
        # "Laser_Tcycle"
        # "Audio_Tcycle_R"
        # "Audio_Tcycle_L"
        # "dataLick"
        # "dataLC"
        # "dataLC"
        # "dataBlock"
        # "dataBlock"
        # "dataMTrig"
        # "dataMTrig"
        # "dataExp"
        # "dataCurrent"
        # "dataExp"
        # "dataCurrent"
        # "spout"
        # "state"
        n819 = call "myRIO_BRig_RT_dataMTrig_Solenoid_Tcycle__L.vi"() -> ("output_Solenoid_Tcycle__L"=w1313:i32)  [unwired: 11 in]
        n820 = call "myRIO_BRig_RT_dataMTrig_Solenoid_Tcycle__R.vi"() -> ("output_Solenoid_Tcycle__R"=w1312:i32)  [unwired: 11 in]
        n821 = call "myRIO_BRig_RT_dataMTrig_Audio_Tcycle__L.vi"() -> ("output_Audio_Tcycle__L"=w1311:i32)  [unwired: 11 in]
        n822 = call "myRIO_BRig_RT_dataMTrig_Audio_Tcycle__R.vi"() -> ("output_Audio_Tcycle__R"=w1310:i32)  [unwired: 11 in]
        n823 = call "myRIO_BRig_RT_dataMTrig_Laser_Tcycle.vi"() -> ("output_Laser_Tcycle"=w1309:i32)  [unwired: 11 in]
        n824 = local read "MTrig_Solenoid_Tcycle__L"() -> (w1292:u16)
        n825 = local read "MTrig_Solenoid_Tcycle__R"() -> (w1291:u16)
        n826 = local read "Tcycle_Reward_L"() -> (w1288:u16)
        n827 = local read "Tcycle_Reward_R"() -> (w1289:u16)
        n828 = local read "MTrig_Laser_Tcycle"() -> (w1290:u16)
        n829 = call "myRIO_BRig_RT_dataMTrig_Solenoid_RewCalib_nCycle__L.vi"() -> ("output_Solenoid_RewCalib_nCycle__L"=w1295:i32)  [unwired: 11 in]
        n830 = call "myRIO_BRig_RT_dataMTrig_Solenoid_Tdelay__L.vi"() -> ("output_Solenoid_Tdelay__L"=w1297:i32)  [unwired: 11 in]
        n831 = call "myRIO_BRig_RT_dataMTrig_Solenoid_RewCalib_nCycle__R.vi"() -> ("output_Solenoid_RewCalib_nCycle__R"=w1296:i32)  [unwired: 11 in]
        n832 = call "myRIO_BRig_RT_dataMTrig_Solenoid_Tdelay__R.vi"() -> ("output_Solenoid_Tdelay__R"=w1298:i32)  [unwired: 11 in]
        n833 = case shown="False" w1275 {
          selector: w1275 -> [_ w1339]
          tunnel: w1274 -> [w1336 w1341]
          tunnel: [w1337 w1341] -> w1270
          tunnel: w1273 -> [_ w1340]
          tunnel: [w1338 w1340] -> w1271
          tunnel: [w1335 w1339] -> w1269
          frame False {
            n834 = call "myRIO__TCP_connect_forWriting.vi"("input_error"=w1336) -> ("output_error"=w1337:errorcluster, "output_connected"=w1335:bool, "output_hTCP"=w1338:refnum<k5>)  [unwired: 8 in]
          }
          frame True {
          }
        }
        n835 = call "myRIO_BRig_RT_dataLick_init.vi"() -> ("output_dataLick"=w1319:u16[][])  [unwired: 11 in]
        n836 = call "myRIO_BRig_RT_dataCurrent_init.vi"() -> ("output_dataCurrent"=w1326:u16[])  [unwired: 11 in]
        n837 = call "myRIO_BRig_RT_dataExp_init.vi"() -> ("output_dataExp"=w1325:u16[])  [unwired: 11 in]
        n838 = call "myRIO_BRig_RT_dataMTrig_init.vi"() -> ("output_dataMTrig"=w1315:u16[])  [unwired: 5 in]
        n839 = call "myRIO_BRig_RT_dataLC_init.vi"() -> ("output_dataLC"=w1323:u16[])  [unwired: 11 in]
        n840 = call "myRIO_BRig_RT_dataBlock_init.vi"() -> ("output_dataBlock"=w1324:u16[][])  [unwired: 11 in]
        n841 = call "myRIO_BRig_RT_dataTrial_init.vi"() -> ("output_dataTrial"=w1308:u16[][])  [unwired: 11 in]
        n842 = local write "I_connect_TCP"(w1269) -> ()
        n843 = Replace Array Subset(array=w1315, new element #1=w1287, index #1=w1295, new element #2=w1287, index #2=w1296, new element #3=w1286, index #3=w1297, new element #4=w1286, index #4=w1298, new element #5=w1292, index #5=w1313, new element #6=w1291, index #6=w1312, new element #7=w1288, index #7=w1311, new element #8=w1289, index #8=w1310, new element #9=w1290, index #9=w1309) -> (w1314:u16[])
        n844 = call "myRIO_BRig_RT_dataAnalog_init.vi"() -> ("output_dataAnalog"=w1280:u16[][])  [unwired: 11 in]
        n845 = call "myRIO_BRig_RT_TCP__start_exp.vi"("input_hTCP"=w1271, "input_I_connected_TCP"=w1269, "input_error"=w1270) -> ("output_hTCP"=w1268:refnum<k5>, "output_error"=w1267:errorcluster)  [unwired: 11 in]
        n846 = Get Date/Time In Seconds() -> (seconds since 1Jan1904=w1294:timestamp)
        n847 = call "myRIO_BRig_RT_arrTrig_init.vi"() -> ("output_arrTrig"=w1264:bool[])  [unwired: 11 in]
        n848 = To Double Precision Float(number=w1294) -> (double precision float=w1293:dbl)
        n849 = node-c288() -> (w1334:T3)  [unwired: 4 in]
        n850 = timed-loop {
          timing: w1334 -> [_]
          timing-out: [_] -> w1333
          shift-right: [w1460] -> _
          shift-left: myRIO_BRig_RT__Case_Exp_stateList."Start1" ("Enum") -> [w1412]
          shift-right: [w1409] -> _
          shift-left: enum16{"Left", "Right"}."Left" -> [w1508]
          tunnel: w1263 -> [w1506]
          tunnel: w1262 -> [w1505]
          shift-right: [w1500] -> _
          shift-left: w1331 -> [w1504]
          shift-right: [w1499] -> _
          shift-left: w1330 -> [w1503]
          tunnel: [w1483] -> w1328
          tunnel: [w1484] -> w1329
          shift-right: [w1485] -> w1299
          shift-left: w1326 -> [w1452]
          shift-right: [w1498] -> _
          shift-left: w1325 -> [w1450]
          shift-right: [w1472] -> w1303
          shift-left: w1314 -> [w1473]
          shift-right: [w1496] -> _
          shift-left: w1324 -> [w1497]
          shift-right: [w1494] -> _
          shift-left: w1323 -> [w1495]
          shift-right: [w1486] -> w1305
          shift-left: w1319 -> [w1487]
          shift-right: [w1474] -> _
          shift-left: w1317 -> [w1482]
          shift-right: [w1447] -> _
          shift-left: w1283 -> [w1481]
          shift-right: [w1475] -> _
          shift-left: w1317 -> [w1480]
          shift-right: [w1476] -> _
          shift-left: w1283 -> [w1479]
          shift-right: [w1448] -> _
          shift-left: w1316 -> [w1477]
          shift-right: [w1449] -> _
          shift-left: w1316 -> [w1478]
          shift-right: [w1458] -> _
          shift-left: w1308 -> [w1459]
          shift-right: [w1457] -> w1301
          shift-left: w1307 -> [w1455]
          shift-right: [w1456] -> w1302
          shift-left: FALSE ("output_Iconnected") -> [w1454]
          tunnel: "Data Set Prefix" -> [w1453]
          tunnel: [w1453] -> w1300
          tunnel: w1293 -> [w1451]
          shift-right: [w1445] -> _
          shift-left: 0 ("idxDataBlock") -> [w1446]
          shift-right: [w1442] -> _
          shift-left: w1284 -> [w1444]
          shift-right: [w1441] -> _
          shift-left: w1284 -> [w1443]
          shift-right: [w1431] -> w1278
          shift-left: 0 -> [w1415]
          shift-right: [w1410] -> _
          shift-left: w1265 -> [w1426]
          shift-right: [w1411] -> _
          shift-left: w1265 -> [w1422]
          shift-right: [w1435] -> _
          shift-left: FALSE -> [w1435]
          shift-right: [w1421] -> _
          shift-left: w1265 -> [w1429]
          shift-right: [w1432] -> w1279
          shift-left: w1280 -> [w1433]
          tunnel: w1268 -> [w1420]
          tunnel: [w1419] -> w1277
          tunnel: w1269 -> [w1416]
          tunnel: [w1416] -> w1276
          tunnel: w1267 -> [w1418]
          tunnel: [w1417] -> w1272
          shift-right: [w1407] -> _
          shift-left: u16 0 -> [w1408]
          shift-right: [w1405] -> _
          shift-left: w1265 -> [w1406]
          shift-right: [w1402] -> _
          shift-left: w1264 -> [w1403]
          stop <- w1493 stop-if-true
          # "arrTrig"
          # "arrTrig"
          # "LC_Laser_l2"
          # "LC_Event_l2"
          # "LC_Laser_l1"
          # "LC_Event_l1"
          # "CueLed"
          # "LC_Laser_l2"
          # "LC_Event_l2"
          # "LC_Laser_l1"
          # "LC_Event_l1"
          # "solenoid__R"
          # "solenoid__L"
          # "spout"
          # "iState"
          # "dataAnalog"
          # "index"
          # "iEvent"
          # "iBlock"
          # "iTrial"
          # "Laser"
          # "Audio R"
          # "Audio L"
          # "Solenoid R"
          # "Solenoid L"
          # "manual triggering"
          # "dataTrial"
          # "dataBlock"
          # "nRewards"
          # "dataExp"
          # "dataCurrent"
          # "audio__L\naudio__R"
          # "time stamp"
          # "Audio params"
          # "nRewards"
          # "idxDataBlock"
          # "idxDataBlock"
          # "activate"
          # "audio__L\naudio__R"
          # "amp__R\nfreq__R"
          # "amp__L\nfreq__L"
          # "dataLC"
          # "solenoid__R"
          # "solenoid__L"
          # "Did a lick occur?"
          # "Update lick counter"
          # "spout"
          # "spout"
          # "state"
          # "state"
          n851 = node-c288() -> ()  [unwired: 1 in, 1 out]
          n852 = local read "MTrig_Solenoid_trig__L"() -> (w1470:bool)
          n853 = local read "MTrig_Solenoid_trig__R"() -> (w1469:bool)
          n854 = local read "MTrig_Audio_trig__L"() -> (w1468:bool)
          n855 = local read "MTrig_Audio_trig__R"() -> (w1467:bool)
          n856 = xnode "Read/Write Control"("FPGA VI Reference In"=w1506, "error in"=w1505) -> ("FPGA VI Reference Out"=w1440:refnum<k20>, "error out"=w1439:errorcluster, "A2_LickL"=w1500:u32, "A4_LickR"=w1499:u32)
          "A2" <- w1500
          "A4" <- w1499
          n857 = local read "MTrig_Laser_trig"() -> (w1466:bool)
          n858 = Greater?(x=w1500, y=w1504) -> (0:w1502:bool)
          n859 = Greater?(x=w1499, y=w1503) -> (0:w1501:bool)
          n860 = Or(x=w1502, y=w1501) -> (x .or. y?=w1507:bool)
          n861 = call "myRIO_BRig_RT_dataMTrig_main.vi"("input_dataMTrig"=w1473, "input_Solenoid_trig_L"=w1470, "input_Solenoid_trig_R"=w1469, "input_Audio_trig_L"=w1468, "input_Audio_trig_R"=w1467, "input_Laser_trig"=w1466) -> ("output_Laser"=w1398:bool, "output_dataMTrig"=w1472:u16[], "output_Solenoid_L"=w1401:bool, "output_Solenoid_R"=w1462:bool, "output_Audio_L"=w1464:bool, "output_Audio_R"=w1465:bool)  [unwired: 8 in]
          n862 = Compound Arithmetic op=OR(w1470, w1469, w1468, w1467, w1466) -> (w1471:bool)
          n863 = case shown="True" w1471 {
            frame False {
            }
            frame True {
              w1509 = FALSE
              n864 = local write "MTrig_Solenoid_trig__L"(w1509) -> ()
              n865 = local write "MTrig_Solenoid_trig__R"(w1509) -> ()
              n866 = local write "MTrig_Audio_trig__L"(w1509) -> ()
              n867 = local write "MTrig_Audio_trig__R"(w1509) -> ()
              n868 = local write "MTrig_Laser_trig"(w1509) -> ()
            }
          }
          n869 = case shown="\"initTrial\"" w1412 {
            selector: w1412 -> [_ _ _ _ _ _ _ _ _ _ _ _ _ _ _ _ _ _ _ _ _ _ _ _ _ _ w2574 _ w2629 _ _ _ _ _ w2746 _ w2819 _ _ _ _ _ w2938 _ w3009 _ w3073 _ w3117 _ _ w3187 _ _ _ _ _ w3358 _ _ _ _ _ _ _ _ _ _ _ _ w3639 w3672]
            tunnel: [myRIO_BRig_RT__Case_Exp_stateList."Start2" ("Enum") myRIO_BRig_RT__Case_Exp_stateList."Start3" ("Enum") myRIO_BRig_RT__Case_Exp_stateList."saveSettings1" ("Enum") myRIO_BRig_RT__Case_Exp_stateList."saveSettings2" ("Enum") myRIO_BRig_RT__Case_Exp_stateList."saveSettings3" ("Enum") myRIO_BRig_RT__Case_Exp_stateList."saveSettings4" ("Enum") myRIO_BRig_RT__Case_Exp_stateList."saveSettings_LC_ENL_l1" ("Enum") myRIO_BRig_RT__Case_Exp_stateList."saveSettings_LC_ENL_l2" ("Enum") myRIO_BRig_RT__Case_Exp_stateList."saveSettings_LC_Cue_l1" ("Enum") myRIO_BRig_RT__Case_Exp_stateList."saveSettings_LC_Cue_l2" ("Enum") myRIO_BRig_RT__Case_Exp_stateList."saveSettings6_LC_l1_Other" ("Enum") myRIO_BRig_RT__Case_Exp_stateList."SaveSettings6_LC_l2_Other" ("Enum") myRIO_BRig_RT__Case_Exp_stateList."setSettings_Audio" ("Enum") myRIO_BRig_RT__Case_Exp_stateList."setSettings_Laser" ("Enum") myRIO_BRig_RT__Case_Exp_stateList."commConnect" ("Enum") w2289 myRIO_BRig_RT__Case_Exp_stateList."initTrial" ("Enum") w2335 myRIO_BRig_RT__Case_Exp_stateList."initTrial3" ("Enum") myRIO_BRig_RT__Case_Exp_stateList."initTrial_LC_ENL1" ("Enum") myRIO_BRig_RT__Case_Exp_stateList."ENL1_pre" ("Enum") myRIO_BRig_RT__Case_Exp_stateList."initTrial_LC_Cue1" ("Enum") myRIO_BRig_RT__Case_Exp_stateList."initTrial_LC_Sel" ("Enum") myRIO_BRig_RT__Case_Exp_stateList."initTrial_LC_Sel" ("Enum") myRIO_BRig_RT__Case_Exp_stateList."initTrial4" ("Enum") w2545 w2571 myRIO_BRig_RT__Case_Exp_stateList."ENL1Penalty" ("Enum") w2630 myRIO_BRig_RT__Case_Exp_stateList."endExp" ("Enum") myRIO_BRig_RT__Case_Exp_stateList."endExp" ("Enum") myRIO_BRig_RT__Case_Exp_stateList."endExp" ("Enum") myRIO_BRig_RT__Case_Exp_stateList."endExp" ("Enum") w2719 w2745 myRIO_BRig_RT__Case_Exp_stateList."Cue1Penalty" ("Enum") w2817 myRIO_BRig_RT__Case_Exp_stateList."endExp" ("Enum") myRIO_BRig_RT__Case_Exp_stateList."endExp" ("Enum") myRIO_BRig_RT__Case_Exp_stateList."endExp" ("Enum") myRIO_BRig_RT__Case_Exp_stateList."endExp" ("Enum") w2908 w2937 myRIO_BRig_RT__Case_Exp_stateList."SelectReward" ("Enum") w3010 myRIO_BRig_RT__Case_Exp_stateList."SelectRewardPost" ("Enum") w3074 myRIO_BRig_RT__Case_Exp_stateList."SelectWrong" ("Enum") w3113 myRIO_BRig_RT__Case_Exp_stateList."endTrial1" ("Enum") myRIO_BRig_RT__Case_Exp_stateList."SelectTimeout" ("Enum") w3189 myRIO_BRig_RT__Case_Exp_stateList."endTrial1" ("Enum") myRIO_BRig_RT__Case_Exp_stateList."endTrial2" ("Enum") myRIO_BRig_RT__Case_Exp_stateList."endTrial3" ("Enum") w3275 w3341 w3358 myRIO_BRig_RT__Case_Exp_stateList."initBlock" ("Enum") w3385 myRIO_BRig_RT__Case_Exp_stateList."commUpload_dataExp" ("Enum") myRIO_BRig_RT__Case_Exp_stateList."endBlock" ("Enum") myRIO_BRig_RT__Case_Exp_stateList."commUpload_dataLC" ("Enum") myRIO_BRig_RT__Case_Exp_stateList."commUpload_dataTrial" ("Enum") myRIO_BRig_RT__Case_Exp_stateList."commUpload_dataCurrent" ("Enum") myRIO_BRig_RT__Case_Exp_stateList."saveData_dataCurrent" ("Enum") myRIO_BRig_RT__Case_Exp_stateList."saveData_dataExp" ("Enum") myRIO_BRig_RT__Case_Exp_stateList."saveData_dataLC" ("Enum") myRIO_BRig_RT__Case_Exp_stateList."saveData_dataTrial" ("Enum") myRIO_BRig_RT__Case_Exp_stateList."commUpload_pre" ("Enum") w3638 w3671] -> w1460
            tunnel: [w1538 w1557 w1579 w1640 w1700 w1766 w1829 w1893 w1957 w2021 w2085 w2128 w2172 w2198 w2260 w2266 w2297 w2318 w2349 w2397 w2426 w2451 w2473 w2490 w2527 w2559 w2587 w2612 w2634 w2650 w2672 w2691 w2710 w2718 w2767 w2795 w2816 w2837 w2858 w2877 w2896 w2919 w2959 w2984 w3007 w3021 w3071 w3095 w3127 w3148 w3168 w3199 w3222 w3234 w3254 w3295 w3314 w3357 w3374 w3388 w3422 w3443 w3464 w3485 w3506 w3534 w3554 w3581 w3601 w3625 w3659 w3692] -> w1409
            tunnel: w1508 -> [w1538 w1557 w1579 w1640 w1700 w1766 w1829 w1893 w1957 w2021 w2085 w2128 w2172 w2198 w2260 w2288 w2297 w2318 w2349 w2397 w2426 w2451 w2473 w2490 w2527 w2559 w2587 w2612 w2634 w2650 w2672 w2691 w2710 w2718 w2767 w2795 w2816 w2837 w2858 w2877 w2896 w2919 w2959 w2984 w3007 w3021 w3071 w3095 w3127 w3148 w3168 w3199 w3222 w3234 w3254 w3295 w3314 w3357 w3374 w3388 w3422 w3443 w3464 w3485 w3506 w3534 w3554 w3581 w3601 w3625 w3659 w3692]
            tunnel: w1507 -> [w1541 w1560 w1576 w1643 w1703 w1769 w1832 w1896 w1960 w2024 w2088 w2131 w2175 w2201 w2263 w2282 w2308 w2336 w2373 w2412 w2440 w2463 w2486 w2515 w2540 w2546 w2570 w2615 w2637 w2656 w2675 w2694 w2713 w2722 w2744 w2801 w2823 w2842 w2861 w2880 w2899 w2917 w2957 w2994 w3017 w3052 w3079 w3106 w3130 w3147 w3180 w3204 w3219 w3242 w3253 w3306 w3340 w3361 w3371 w3397 w3425 w3446 w3467 w3488 w3509 w3537 w3557 w3584 w3604 w3628 w3662 w3695]
            tunnel: w1502 -> [w1540 w1559 w1577 w1642 w1702 w1768 w1831 w1895 w1959 w2023 w2087 w2130 w2174 w2200 w2262 w2281 w2307 w2337 w2372 w2413 w2441 w2464 w2487 w2516 w2541 w2563 w2589 w2614 w2636 w2655 w2674 w2693 w2712 w2736 w2768 w2800 w2822 w2841 w2860 w2879 w2898 w2918 w2956 w2993 w3016 w3051 w3078 w3105 w3129 w3146 w3179 w3203 w3220 w3243 w3252 w3305 w3339 w3360 w3372 w3398 w3424 w3445 w3466 w3487 w3508 w3536 w3556 w3583 w3603 w3627 w3661 w3694]
            tunnel: w1501 -> [w1539 w1558 w1578 w1641 w1701 w1767 w1830 w1894 w1958 w2022 w2086 w2129 w2173 w2199 w2261 w2280 w2306 w2338 w2371 w2414 w2442 w2465 w2488 w2517 w2542 w2562 w2588 w2613 w2635 w2654 w2673 w2692 w2711 w2735 w2769 w2799 w2821 w2840 w2859 w2878 w2897 w2929 w2960 w2992 w3015 w3050 w3077 w3104 w3128 w3145 w3178 w3202 w3221 w3244 w3251 w3304 w3338 w3359 w3373 w3399 w3423 w3444 w3465 w3486 w3507 w3535 w3555 w3582 w3602 w3626 w3660 w3693]
            tunnel: [w1541 w1560 w1576 w1643 w1703 w1769 w1832 w1896 w1960 w2024 w2088 w2131 w2175 w2201 w2263 w2282 w2308 w2336 w2373 w2412 w2440 w2463 w2486 w2515 w2540 w2546 w2570 w2615 w2637 w2656 w2675 w2694 w2713 w2722 w2744 w2801 w2823 w2842 w2861 w2880 w2899 w2917 w2957 w2994 w3017 w3052 w3079 w3106 w3130 w3147 w3180 w3204 w3219 w3242 w3253 w3306 w3340 w3361 w3371 w3397 w3425 w3446 w3467 w3488 w3509 w3537 w3557 w3584 w3604 w3628 w3662 w3695] -> w1490
            tunnel: [w1540 w1559 w1577 w1642 w1702 w1768 w1831 w1895 w1959 w2023 w2087 w2130 w2174 w2200 w2262 w2281 w2307 w2337 w2372 w2413 w2441 w2464 w2487 w2516 w2541 w2563 w2589 w2614 w2636 w2655 w2674 w2693 w2712 w2736 w2768 w2800 w2822 w2841 w2860 w2879 w2898 w2918 w2956 w2993 w3016 w3051 w3078 w3105 w3129 w3146 w3179 w3203 w3220 w3243 w3252 w3305 w3339 w3360 w3372 w3398 w3424 w3445 w3466 w3487 w3508 w3536 w3556 w3583 w3603 w3627 w3661 w3694] -> w1489
            tunnel: [w1539 w1558 w1578 w1641 w1701 w1767 w1830 w1894 w1958 w2022 w2086 w2129 w2173 w2199 w2261 w2280 w2306 w2338 w2371 w2414 w2442 w2465 w2488 w2517 w2542 w2562 w2588 w2613 w2635 w2654 w2673 w2692 w2711 w2735 w2769 w2799 w2821 w2840 w2859 w2878 w2897 w2929 w2960 w2992 w3015 w3050 w3077 w3104 w3128 w3145 w3178 w3202 w3221 w3244 w3251 w3304 w3338 w3359 w3373 w3399 w3423 w3444 w3465 w3486 w3507 w3535 w3555 w3582 w3602 w3626 w3660 w3693] -> w1488
            tunnel: w1452 -> [w1537 w1556 w1575 w1607 w1676 w1704 w1770 w1892 w1956 w2020 w2084 w2127 w2171 w2196 w2210 w2287 w2296 w2334 w2348 w2383 w2425 w2450 w2472 w2500 w2526 w2547 w2573 w2606 w2633 w2651 w2671 w2690 w2709 w2721 w2764 w2794 w2820 w2838 w2857 w2876 w2895 w2910 w2940 w2976 w3012 w3023 w3076 w3096 w3126 w3144 w3169 w3201 w3218 w3231 w3256 w3277 w3312 w3356 w3375 w3400 w3419 w3440 w3461 w3482 w3493 w3523 w3542 w3566 w3598 w3614 w3637 w3670]
            tunnel: w1450 -> [w1536 w1555 w1574 w1638 w1698 w1763 w1826 w1890 w1954 w2018 w2082 w2125 w2169 w2189 w2202 w2286 w2305 w2333 w2356 w2378 w2428 w2443 w2476 w2505 w2530 w2561 w2586 w2605 w2631 w2653 w2670 w2689 w2708 w2717 w2766 w2792 w2815 w2839 w2856 w2875 w2894 w2900 w2958 w2990 w3014 w3044 w3072 w3097 w3124 w3143 w3171 w3198 w3217 w3241 w3245 w3276 w3331 w3355 w3376 w3401 w3418 w3439 w3460 w3481 w3494 w3531 w3551 w3562 w3597 w3622 w3656 w3689]
            tunnel: [w1537 w1556 w1575 w1607 w1676 w1704 w1770 w1892 w1956 w2020 w2084 w2127 w2171 w2196 w2209 w2271 w2296 w2323 w2348 w2382 w2425 w2449 w2471 w2499 w2525 w2544 w2572 w2607 w2632 w2651 w2671 w2690 w2709 w2720 w2763 w2793 w2818 w2838 w2857 w2876 w2895 w2909 w2939 w2991 w3011 w3045 w3075 w3098 w3125 w3144 w3172 w3200 w3218 w3230 w3255 w3277 w3310 w3356 w3375 w3400 w3419 w3440 w3461 w3482 w3493 w3523 w3542 w3566 w3598 w3614 w3637 w3670] -> w1383
            tunnel: [w1536 w1555 w1574 w1637 w1697 w1758 w1825 w1890 w1954 w2018 w2082 w2125 w2169 w2189 w2202 w2285 w2305 w2332 w2356 w2378 w2428 w2443 w2476 w2505 w2530 w2561 w2586 w2605 w2631 w2653 w2670 w2689 w2708 w2717 w2766 w2792 w2815 w2839 w2856 w2875 w2894 w2900 w2958 w2990 w3014 w3044 w3072 w3097 w3124 w3143 w3171 w3198 w3217 w3241 w3245 w3276 w3331 w3355 w3376 w3401 w3418 w3439 w3460 w3481 w3494 w3531 w3551 w3565 w3597 w3622 w3656 w3689] -> w1498
            tunnel: [_ _ _ _ _ _ _ _ _ _ _ _ _ _ _ _ _ _ _ _ _ _ _ _ _ _ _ _ _ _ _ _ _ _ _ _ _ _ _ _ _ _ _ _ w3005 _ _ _ _ _ _ _ _ _ _ _ _ _ _ _ _ _ _ _ _ _ _ _ _ _ _ _] -> w1400
            tunnel: [_ _ _ _ _ _ _ _ _ _ _ _ _ _ _ _ _ _ _ _ _ _ _ _ _ _ _ _ _ _ _ _ _ _ _ _ _ _ _ _ _ _ _ _ w3006 _ _ _ _ _ _ _ _ _ _ _ _ _ _ _ _ _ _ _ _ _ _ _ _ _ _ _] -> w1463
            tunnel: w1497 -> [w1534 w1553 w1572 w1609 w1678 w1764 w1827 w1891 w1955 w2019 w2083 w2126 w2170 w2194 w2257 w2283 w2298 w2313 w2364 w2410 w2438 w2446 w2468 w2489 w2522 w2560 w2585 w2602 w2627 w2652 w2668 w2687 w2706 w2734 w2765 w2791 w2813 w2835 w2854 w2873 w2892 w2928 w2954 w2982 w3013 w3025 w3069 w3094 w3122 w3141 w3170 w3197 w3215 w3233 w3260 w3302 w3323 w3353 w3378 w3403 w3416 w3437 w3458 w3479 w3503 w3517 w3544 w3572 w3591 w3616 w3650 w3683]
            tunnel: [w1534 w1553 w1572 w1609 w1678 w1764 w1827 w1891 w1955 w2019 w2083 w2126 w2170 w2194 w2257 w2283 w2295 w2313 w2364 w2410 w2438 w2446 w2468 w2489 w2522 w2560 w2585 w2602 w2627 w2652 w2668 w2687 w2706 w2734 w2765 w2791 w2813 w2835 w2854 w2873 w2892 w2928 w2954 w2982 w3013 w3024 w3069 w3094 w3122 w3141 w3170 w3197 w3215 w3232 w3260 w3302 w3323 w3353 w3378 w3403 w3416 w3437 w3458 w3479 w3503 w3517 w3544 w3572 w3591 w3616 w3650 w3683] -> w1496
            tunnel: w1495 -> [w1535 w1554 w1573 w1608 w1677 w1765 w1828 w1888 w1952 w2016 w2080 w2123 w2167 w2195 w2258 w2284 w2304 w2331 w2347 w2411 w2439 w2452 w2474 w2503 w2528 w2558 w2569 w2603 w2628 w2649 w2669 w2688 w2707 w2733 w2743 w2790 w2814 w2836 w2855 w2874 w2893 w2927 w2955 w2983 w3008 w3042 w3070 w3093 w3123 w3142 w3167 w3196 w3216 w3240 w3259 w3303 w3330 w3354 w3377 w3402 w3417 w3438 w3459 w3480 w3504 w3530 w3550 w3578 w3589 w3621 w3655 w3688]
            tunnel: [w1535 w1554 w1573 w1608 w1677 w1765 w1828 w1889 w1953 w2017 w2081 w2124 w2168 w2195 w2258 w2284 w2304 w2331 w2347 w2411 w2439 w2452 w2474 w2503 w2528 w2558 w2569 w2603 w2628 w2649 w2669 w2688 w2707 w2733 w2743 w2790 w2814 w2836 w2855 w2874 w2893 w2927 w2955 w2983 w3008 w3042 w3070 w3093 w3123 w3142 w3167 w3196 w3216 w3240 w3259 w3303 w3330 w3354 w3377 w3402 w3417 w3438 w3459 w3480 w3504 w3530 w3550 w3578 w3589 w3621 w3655 w3688] -> w1494
            tunnel: [_ _ _ _ _ _ _ _ _ _ _ _ _ _ _ _ _ _ _ _ _ _ _ _ _ _ _ _ _ _ _ _ _ _ _ _ _ _ _ _ _ _ _ _ _ _ _ _ _ _ _ _ _ _ _ _ _ TRUE _ _ _ _ _ _ _ _ _ _ _ _ _ _] -> w1491
            tunnel: w1482 -> [w1532 w1551 w1570 w1599 w1671 w1753 w1824 w1875 w1944 w2003 w2067 w2095 w2149 _ w2249 w2279 w2303 w2330 w2363 w2409 w2437 w2462 w2485 w2514 w2539 w2557 w2584 w2600 w2626 w2647 w2666 w2685 w2704 w2732 w2760 w2788 w2812 w2833 w2852 w2871 w2890 w2926 w2953 w2972 w3004 w3040 w3068 w3091 w3121 w3140 w3165 w3195 w3214 w3238 w3264 w3301 w3327 w3351 w3369 w3396 w3414 w3435 w3456 w3477 w3501 w3528 w3548 w3576 w3595 w3620 w3654 w3687]
            tunnel: w1481 -> [w1531 w1550 w1569 w1598 w1670 w1752 w1823 w1874 w1943 w2002 w2066 w2096 w2150 _ w2248 w2278 w2302 w2329 w2362 w2408 w2436 w2461 w2484 w2513 w2538 w2556 w2583 w2599 w2625 w2646 w2665 w2684 w2703 w2731 w2759 w2787 w2811 w2832 w2851 w2870 w2889 w2925 w2952 w2971 w3003 w3039 w3067 w3090 w3120 w3139 w3164 w3194 w3213 w3237 w3263 w3300 w3326 w3350 w3368 w3395 w3413 w3434 w3455 w3476 w3500 w3527 w3547 w3575 w3594 w3619 w3653 w3686]
            tunnel: w1480 -> [w1530 w1549 w1568 w1597 w1669 w1751 w1822 w1873 w1942 w2001 w2065 w2097 w2151 _ w2247 w2277 w2301 w2328 w2361 w2407 w2435 w2460 w2483 w2512 w2537 w2555 w2582 w2598 w2624 w2645 w2664 w2683 w2702 w2730 w2758 w2786 w2810 w2831 w2850 w2869 w2888 w2924 w2951 w2970 w3002 w3038 w3066 w3089 w3119 w3138 w3163 w3193 w3212 w3236 w3262 w3299 w3325 w3349 w3367 w3394 w3412 w3433 w3454 w3475 w3499 w3526 w3546 w3574 w3593 w3618 w3652 w3685]
            tunnel: w1479 -> [w1529 w1548 w1567 w1596 w1668 w1750 w1821 w1872 w1941 w2000 w2064 w2098 w2152 _ w2246 w2276 w2300 w2327 w2360 w2406 w2434 w2459 w2482 w2511 w2536 w2554 w2581 w2597 w2623 w2644 w2663 w2682 w2701 w2729 w2757 w2785 w2809 w2830 w2849 w2868 w2887 w2923 w2950 w2969 w3001 w3037 w3065 w3088 w3118 w3137 w3162 w3192 w3211 w3235 w3261 w3298 w3324 w3348 w3366 w3393 w3411 w3432 w3453 w3474 w3498 w3525 w3545 w3573 w3592 w3617 w3651 w3684]
            tunnel: w1478 -> [_ _ _ _ _ _ _ _ _ _ _ _ _ _ _ _ _ _ _ _ _ _ _ _ _ _ _ _ _ _ _ _ _ _ w2762 _ _ _ _ _ _ _ _ _ _ _ _ _ _ _ _ _ _ _ _ _ _ _ _ _ _ _ _ _ _ _ _ _ _ _ _ _]
            tunnel: w1477 -> [_ _ _ _ _ _ _ _ _ _ _ _ _ _ _ _ _ _ _ _ _ _ _ _ _ _ _ _ _ _ _ _ _ _ w2761 _ _ _ _ _ _ _ _ _ _ _ _ _ _ _ _ _ _ _ _ _ _ _ _ _ _ _ _ _ _ _ _ _ _ _ _ _]
            tunnel: [w1532 w1551 w1570 w1599 w1671 w1753 w1824 w1875 w1944 w2003 w2067 w2095 w2149 w2188 w2249 w2279 w2303 w2330 w2363 w2409 w2437 w2462 w2485 w2514 w2539 w2557 w2584 w2600 w2626 w2647 w2666 w2685 w2704 w2732 w2760 w2788 w2812 w2833 w2852 w2871 w2890 w2926 w2953 w2972 w3004 w3040 w3068 w3091 w3121 w3140 w3165 w3195 w3214 w3238 w3264 w3301 w3327 w3351 w3369 w3396 w3414 w3435 w3456 w3477 w3501 w3528 w3548 w3576 w3595 w3620 w3654 w3687] -> w1474
            tunnel: [w1531 w1550 w1569 w1598 w1670 w1752 w1823 w1874 w1943 w2002 w2066 w2096 w2150 w2179 w2248 w2278 w2302 w2329 w2362 w2408 w2436 w2461 w2484 w2513 w2538 w2556 w2583 w2599 w2625 w2646 w2665 w2684 w2703 w2731 w2759 w2787 w2811 w2832 w2851 w2870 w2889 w2925 w2952 w2971 w3003 w3039 w3067 w3090 w3120 w3139 w3164 w3194 w3213 w3237 w3263 w3300 w3326 w3350 w3368 w3395 w3413 w3434 w3455 w3476 w3500 w3527 w3547 w3575 w3594 w3619 w3653 w3686] -> w1447
            tunnel: [w1530 w1549 w1568 w1597 w1669 w1751 w1822 w1873 w1942 w2001 w2065 w2097 w2151 w2187 w2247 w2277 w2301 w2328 w2361 w2407 w2435 w2460 w2483 w2512 w2537 w2555 w2582 w2598 w2624 w2645 w2664 w2683 w2702 w2730 w2758 w2786 w2810 w2831 w2850 w2869 w2888 w2924 w2951 w2970 w3002 w3038 w3066 w3089 w3119 w3138 w3163 w3193 w3212 w3236 w3262 w3299 w3325 w3349 w3367 w3394 w3412 w3433 w3454 w3475 w3499 w3526 w3546 w3574 w3593 w3618 w3652 w3685] -> w1475
            tunnel: [w1529 w1548 w1567 w1596 w1668 w1750 w1821 w1872 w1941 w2000 w2064 w2098 w2152 w2177 w2246 w2276 w2300 w2327 w2360 w2406 w2434 w2459 w2482 w2511 w2536 w2554 w2581 w2597 w2623 w2644 w2663 w2682 w2701 w2729 w2757 w2785 w2809 w2830 w2849 w2868 w2887 w2923 w2950 w2969 w3001 w3037 w3065 w3088 w3118 w3137 w3162 w3192 w3211 w3235 w3261 w3298 w3324 w3348 w3366 w3393 w3411 w3432 w3453 w3474 w3498 w3525 w3545 w3573 w3592 w3617 w3651 w3684] -> w1476
            tunnel: [_ _ _ _ _ _ _ _ _ _ _ _ _ _ _ _ _ _ _ _ _ _ _ _ _ _ _ _ _ _ _ _ _ w2716 w2762 _ _ _ _ _ _ _ _ _ _ _ _ _ _ _ _ _ _ _ _ _ _ _ _ _ _ _ _ _ _ _ _ _ _ _ _ _] -> w1449
            tunnel: [_ _ _ _ _ _ _ _ _ _ _ _ _ _ _ _ _ _ _ _ _ _ _ _ _ _ _ _ _ _ _ _ _ w2715 w2761 _ _ _ _ _ _ _ _ _ _ _ _ _ _ _ _ _ _ _ _ _ _ _ _ _ _ _ _ _ _ _ _ _ _ _ _ _] -> w1448
            tunnel: w1459 -> [w1528 w1547 w1566 w1595 w1667 w1749 w1820 w1871 w1940 w1999 w2063 w2094 w2148 w2186 w2256 w2275 w2299 w2326 w2351 w2399 w2424 w2448 w2470 w2501 w2524 w2553 w2580 w2596 w2622 w2643 w2662 w2681 w2700 w2728 w2756 w2784 w2808 w2829 w2848 w2867 w2886 w2922 w2949 w2966 w3000 w3036 w3064 w3085 w3112 w3136 w3159 w3186 w3210 w3229 w3258 w3291 w3322 w3347 w3379 w3404 w3415 w3436 w3457 w3478 w3502 w3529 w3549 w3577 w3596 w3611 w3649 w3682]
            tunnel: [w1528 w1547 w1566 w1595 w1667 w1749 w1820 w1871 w1940 w1999 w2063 w2094 w2148 w2186 w2256 w2275 w2299 w2326 w2350 w2398 w2417 w2447 w2469 w2501 w2523 w2553 w2580 w2596 w2622 w2643 w2662 w2681 w2700 w2728 w2756 w2784 w2808 w2829 w2848 w2867 w2886 w2922 w2949 w2966 w3000 w3036 w3064 w3085 w3112 w3136 w3159 w3186 w3210 w3229 w3257 w3291 w3322 w3347 w3379 w3404 w3415 w3436 w3457 w3478 w3502 w3529 w3549 w3577 w3596 w3611 w3649 w3682] -> w1458
            tunnel: [w1527 w1546 w1565 w1594 w1666 w1748 w1819 w1870 w1939 w1998 w2062 w2093 w2147 w2185 w2255 w2274 w2310 w2325 w2366 w2405 w2433 w2458 w2481 w2510 w2535 w2552 w2579 w2595 w2621 w2642 w2661 w2680 w2699 w2727 w2755 w2783 w2807 w2828 w2847 w2866 w2885 w2921 w2948 w2965 w2999 w3035 w3063 w3084 w3111 w3135 w3158 w3185 w3209 w3228 w3250 w3297 w3321 w3345 w3380 w3390 w3410 w3431 w3452 w3473 w3497 w3533 w3553 w3580 w3600 w3624 w3658 w3691] -> w1457
            tunnel: [w1526 w1545 w1564 w1593 w1665 w1747 w1818 w1869 w1938 w1997 w2061 w2092 w2146 w2184 w2254 w2273 w2309 w2324 w2365 w2404 w2432 w2457 w2480 w2509 w2534 w2551 w2578 w2594 w2620 w2641 w2660 w2679 w2698 w2726 w2754 w2782 w2806 w2827 w2846 w2865 w2884 w2920 w2947 w2964 w2998 w3034 w3062 w3083 w3110 w3134 w3157 w3184 w3208 w3227 w3249 w3296 w3320 w3346 w3362 w3387 w3420 w3441 w3462 w3483 w3505 w3532 w3552 w3579 w3599 w3623 w3657 w3690] -> w1456
            tunnel: w1455 -> [w1527 w1546 w1565 w1594 w1666 w1748 w1819 w1870 w1939 w1998 w2062 w2093 w2147 w2185 w2255 w2274 w2310 w2325 w2366 w2405 w2433 w2458 w2481 w2510 w2535 w2552 w2579 w2595 w2621 w2642 w2661 w2680 w2699 w2727 w2755 w2783 w2807 w2828 w2847 w2866 w2885 w2921 w2948 w2965 w2999 w3035 w3063 w3084 w3111 w3135 w3158 w3185 w3209 w3228 w3250 w3297 w3321 w3345 _ w3390 w3410 w3431 w3452 w3473 w3497 w3533 w3553 w3580 w3600 w3624 w3658 w3691]
            tunnel: w1454 -> [w1526 w1545 w1564 w1593 w1665 w1747 w1818 w1869 w1938 w1997 w2061 w2092 w2146 w2184 w2254 w2273 w2309 w2324 w2365 w2404 w2432 w2457 w2480 w2509 w2534 w2551 w2578 w2594 w2620 w2641 w2660 w2679 w2698 w2726 w2754 w2782 w2806 w2827 w2846 w2865 w2884 w2920 w2947 w2964 w2998 w3034 w3062 w3083 w3110 w3134 w3157 w3184 w3208 w3227 w3249 w3296 w3320 w3346 _ w3387 w3420 w3441 w3462 w3483 w3505 w3532 w3552 w3579 w3599 w3623 w3657 w3690]
            tunnel: w1453 -> [_ _ _ _ _ _ _ _ _ _ _ _ _ _ _ _ _ _ _ _ _ _ _ _ _ _ _ _ _ _ _ _ _ _ _ _ _ _ _ _ _ _ _ _ _ _ _ _ _ _ _ _ _ _ _ _ _ _ _ _ w3408 w3429 w3450 w3471 w3495 _ _ _ _ _ _ _]
            tunnel: w1451 -> [_ _ _ _ _ _ _ _ _ _ _ _ _ _ _ _ _ _ _ _ _ _ _ _ _ _ _ _ _ _ _ _ _ _ _ _ _ _ _ _ _ _ _ _ _ _ _ _ _ _ _ _ _ _ _ _ _ _ _ _ _ _ _ _ _ _ _ w3567 _ _ _ _]
            tunnel: [w1525 w1544 w1563 w1592 w1664 w1746 w1817 w1868 w1937 w1996 w2060 w2091 w2145 w2183 w2253 w2269 w2293 w2322 w2367 w2403 w2431 w2456 w2479 w2508 w2533 w2550 w2577 w2593 w2619 w2640 w2659 w2678 w2697 w2725 w2753 w2781 w2805 w2826 w2845 w2864 w2883 w2916 w2946 w2963 w2997 w3019 w3061 w3082 w3109 w3133 w3156 w3183 w3207 w3226 w3248 w3294 w3307 w3344 w3365 w3389 w3407 w3428 w3449 w3470 w3492 w3512 w3541 w3561 w3588 w3609 w3648 w3681] -> w1445
            tunnel: w1446 -> [w1525 w1544 w1563 w1592 w1664 w1746 w1817 w1868 w1937 w1996 w2060 w2091 w2145 w2183 w2253 w2269 _ w2322 w2367 w2403 w2431 w2456 w2479 w2508 w2533 w2550 w2577 w2593 w2619 w2640 w2659 w2678 w2697 w2725 w2753 w2781 w2805 w2826 w2845 w2864 w2883 w2916 w2946 w2963 w2997 w3019 w3061 w3082 w3109 w3133 w3156 w3183 w3207 w3226 w3248 w3294 w3308 w3344 w3365 w3389 w3407 w3428 w3449 w3470 w3492 w3512 w3541 w3561 w3588 w3609 w3648 w3681]
            tunnel: w1444 -> [w1524 w1543 w1562 w1591 w1663 w1745 w1816 w1867 w1936 w1995 w2059 w2090 w2144 w2182 w2252 w2268 w2292 w2321 w2359 w2402 w2430 w2455 w2478 w2507 w2532 w2549 w2576 w2592 w2618 w2639 w2658 w2677 w2696 w2724 w2752 w2780 w2804 w2825 w2844 w2863 w2882 w2915 w2945 w2962 w2996 w3033 w3060 w3081 w3108 w3132 w3155 w3182 w3206 w3225 w3247 w3293 w3319 w3343 w3364 w3392 w3406 w3427 w3448 w3469 w3491 w3511 w3540 w3560 w3587 w3608 w3647 w3680]
            tunnel: w1443 -> [w1523 w1542 w1561 w1590 w1662 w1744 w1815 w1866 w1935 w1994 w2058 w2089 w2143 w2181 w2251 w2267 w2291 w2320 w2358 w2401 w2429 w2454 w2477 w2506 w2531 w2548 w2575 w2591 w2617 w2638 w2657 w2676 w2695 w2723 w2751 w2779 w2803 w2824 w2843 w2862 w2881 w2914 w2944 w2961 w2995 w3030 w3059 w3080 w3107 w3131 w3154 w3181 w3205 w3224 w3246 w3292 w3318 w3342 w3363 w3391 w3405 w3426 w3447 w3468 w3490 w3510 w3539 w3559 w3586 w3607 w3646 w3679]
            tunnel: [w1524 w1543 w1562 w1591 w1663 w1745 w1816 w1867 w1936 w1995 w2059 w2090 w2144 w2182 w2252 w2268 w2292 w2321 w2359 w2402 w2430 w2455 w2478 w2507 w2532 w2549 w2576 w2592 w2618 w2639 w2658 w2677 w2696 w2724 w2752 w2780 w2804 w2825 w2844 w2863 w2882 w2915 w2945 w2962 w2996 w3032 w3060 w3081 w3108 w3132 w3155 w3182 w3206 w3225 w3247 w3293 w3319 w3343 w3364 w3392 w3406 w3427 w3448 w3469 w3491 w3511 w3540 w3560 w3587 w3608 w3647 w3680] -> w1442
            tunnel: [w1523 w1542 w1561 w1590 w1662 w1744 w1815 w1866 w1935 w1994 w2058 w2089 w2143 w2181 w2251 w2267 w2291 w2320 w2358 w2401 w2429 w2454 w2477 w2506 w2531 w2548 w2575 w2591 w2617 w2638 w2657 w2676 w2695 w2723 w2751 w2779 w2803 w2824 w2843 w2862 w2881 w2914 w2944 w2961 w2995 w3031 w3059 w3080 w3107 w3131 w3154 w3181 w3205 w3224 w3246 w3292 w3318 w3342 w3363 w3391 w3405 w3426 w3447 w3468 w3490 w3510 w3539 w3559 w3586 w3607 w3646 w3679] -> w1441
            tunnel: w1440 -> [w1522 _ _ _ _ _ _ _ _ _ _ _ _ _ w2244 _ _ w2317 w2370 w2393 _ _ _ _ _ _ _ _ _ _ _ _ _ _ w2748 _ _ _ _ _ _ w2912 w2943 _ _ _ _ _ _ _ w3153 _ _ _ _ w3273 _ _ _ _ _ _ _ _ _ _ _ _ _ _ _ _]
            tunnel: w1439 -> [w1521 _ _ _ _ _ _ _ _ _ _ _ _ _ w2245 _ _ w2316 w2369 w2392 _ _ _ _ _ _ _ _ _ _ _ _ _ _ w2747 _ _ _ _ _ _ w2913 w2942 _ _ _ _ _ _ _ w3152 _ _ _ _ w3272 _ _ _ _ _ _ _ _ _ _ _ _ _ _ _ _]
            tunnel: [_ _ _ _ _ _ _ _ _ _ _ _ _ _ _ _ _ _ _ _ _ _ _ _ _ _ w2567 _ _ _ _ _ _ _ w2741 _ _ _ _ _ _ w2904 w2933 _ _ _ _ _ _ _ _ _ _ _ _ _ _ _ _ _ _ _ _ _ _ _ _ _ _ _ _ _] -> w1391
            tunnel: [_ _ _ _ _ _ _ _ _ _ _ _ _ _ _ _ _ _ _ _ _ _ _ _ _ _ w2566 _ _ _ _ _ _ _ w2740 _ _ _ _ _ _ w2903 w2932 _ _ _ _ _ _ _ _ _ _ _ _ _ _ _ _ _ _ _ _ _ _ _ _ _ _ _ _ _] -> w1390
            tunnel: [_ _ _ _ _ _ _ _ _ _ _ _ _ _ _ _ _ _ _ _ _ _ _ w2502 w2521 _ _ _ _ _ _ _ _ _ _ _ _ _ _ _ _ _ _ _ _ _ _ _ _ _ _ _ _ _ _ _ _ _ _ _ _ _ _ _ _ _ _ _ _ _ _ _] -> w1437
            tunnel: [_ _ _ _ _ _ _ _ _ _ _ _ _ _ _ _ _ _ _ _ _ _ _ _ TRUE ("Recording") _ _ _ _ _ _ _ _ _ _ _ _ _ _ _ _ _ _ _ _ _ _ _ _ _ _ _ _ _ _ _ _ _ _ _ _ _ _ _ _ _ _ _ _ _ _ _] -> w1434
            tunnel: [_ _ _ _ _ _ _ _ _ _ _ _ _ _ _ _ _ _ _ _ _ _ _ w2502 _ _ _ _ _ _ _ _ _ _ _ _ _ _ _ _ _ _ _ _ _ _ _ _ _ _ _ _ _ _ _ _ _ _ _ _ _ _ _ _ _ _ _ _ _ _ _ _] -> w1430
            tunnel: [_ _ _ _ _ _ _ _ _ _ _ _ _ _ _ TRUE _ _ _ _ _ _ _ _ _ _ _ _ _ _ _ _ _ _ _ _ _ _ _ _ _ _ _ _ _ _ _ _ _ _ _ _ _ _ _ _ _ _ _ _ _ _ _ _ _ _ _ _ _ _ _ _] -> w1427
            tunnel: [_ _ _ _ _ _ _ _ _ _ _ _ _ _ _ w2264 _ _ _ _ _ _ _ _ _ _ _ _ _ _ _ _ _ _ _ _ _ _ _ _ _ _ _ _ _ _ _ _ _ _ _ _ _ _ _ _ _ _ _ _ _ _ _ _ _ _ _ _ _ _ _ _] -> w1425
            tunnel: [_ _ _ _ _ _ _ _ _ _ _ _ _ _ _ _ _ TRUE _ _ _ _ _ _ _ _ _ _ _ _ _ _ _ _ _ _ _ _ _ _ _ _ _ _ _ _ _ _ _ _ _ _ _ _ _ _ _ _ _ _ _ _ _ _ _ _ _ _ _ _ _ _] -> w1424
            tunnel: [_ _ _ _ _ _ _ _ _ _ _ _ _ _ _ _ _ w2312 _ _ _ _ _ _ _ _ _ _ _ _ _ _ _ _ _ _ _ _ _ _ _ _ _ _ _ _ _ _ _ _ _ _ _ _ _ _ _ _ _ _ _ _ _ _ _ _ _ _ _ _ _ _] -> w1423
            tunnel: w1408 -> [_ _ _ _ _ _ _ _ _ _ _ _ _ _ _ _ _ _ _ _ _ _ _ _ _ _ _ _ _ _ _ _ _ _ _ _ _ _ _ _ _ _ _ _ _ _ _ _ _ _ _ _ _ _ _ _ _ _ _ _ _ _ _ _ _ _ _ _ _ _ w3644 w3677]
            tunnel: [_ _ _ _ _ _ _ _ _ _ _ _ _ _ _ _ _ _ _ _ _ _ _ _ _ _ _ _ _ _ _ _ _ _ _ _ _ _ _ _ _ _ _ _ _ _ _ _ _ _ _ _ _ _ _ _ _ _ _ _ _ _ _ _ _ _ _ _ _ _ w3642 w3675] -> w1407
            tunnel: w1403 -> [_ _ _ _ _ _ _ _ _ _ _ _ _ _ _ _ _ _ _ _ w2415 w2445 w2467 w2498 w2519 w2543 w2568 w2590 w2616 _ _ _ _ w2714 w2742 w2778 w2802 _ _ _ _ w2905 w2934 _ _ _ _ _ _ _ _ _ _ _ _ _ _ _ _ _ _ _ _ _ _ _ _ _ _ _ _ _]
            tunnel: [_ _ _ _ _ _ _ _ _ _ _ _ _ _ _ _ _ _ _ w2380 w2415 w2444 w2466 w2497 w2518 w2543 w2568 w2590 w2616 _ _ _ _ w2714 w2742 w2778 w2802 _ _ _ _ w2905 w2934 _ _ _ _ _ _ _ _ _ _ _ _ _ _ _ _ _ _ _ _ _ _ _ _ _ _ _ _ _] -> w1402
            tunnel: [_ _ _ _ _ _ _ _ _ _ _ _ _ _ _ _ _ _ _ _ _ _ _ _ _ _ w2565 _ _ _ _ _ _ _ w2739 _ _ _ _ _ _ w2902 w2931 _ _ _ _ _ _ _ _ _ _ _ _ _ _ _ _ _ _ _ _ _ _ _ _ _ _ _ _ _] -> w1395
            tunnel: [_ _ _ _ _ _ _ _ _ _ _ _ _ _ _ _ _ _ _ _ _ _ _ _ _ _ w2564 _ _ _ _ _ _ _ w2738 _ _ _ _ _ _ w2901 w2930 _ _ _ _ _ _ _ _ _ _ _ _ _ _ _ _ _ _ _ _ _ _ _ _ _ _ _ _ _] -> w1393
            tunnel: [_ _ _ _ _ _ _ _ _ _ _ _ _ _ _ _ _ _ _ _ _ _ _ _ _ _ _ _ _ _ _ _ _ _ w2737 _ _ _ _ _ _ _ _ _ _ _ _ _ _ _ _ _ _ _ _ _ _ _ _ _ _ _ _ _ _ _ _ _ _ _ _ _] -> w1399
            frame "Start1", Default {
              w1520 = FALSE ("SelectionState")
              n870 = xnode "Read/Write Control"("FPGA VI Reference In"=w1522, "error in"=w1521, "SelectionState"=w1520, "LR_reward_Laser_l1"=w1520, "LR_wrong_Laser_l1"=w1520, "LR_reward_Event_l1"=w1520, "LR_wrong_Event_l1"=w1520, "Left(F)_or_Right(T)"=w1520, "ignoreWrong"=w1520, "SelectionState"=w1520, "LR_reward_Laser_l2"=w1520, "LR_wrong_laser_l2"=w1520, "LR_reward_Event_l2"=w1520, "LR_wrong_Event_l2"=w1520, "LC_Event_l1"=w1520, "LC_Laser_l1"=w1520, "LC_Laser_l2"=w1520, "LC_Event_l2"=w1520, "CueLed_Event"=w1520) -> ()  [unwired: 2 out]
            }
            frame "Start2" {
            }
            frame "Start3" {
            }
            frame "saveSettings1" {
              n871 = call "myRIO_BRig_RT_dataExp_Audio_freq__L.vi"() -> ("output_Audio_freq__L"=w1615:i32)  [unwired: 11 in]
              n872 = call "myRIO_BRig_RT_dataExp_Audio_freq__R.vi"() -> ("output_Audio_freq__R"=w1614:i32)  [unwired: 11 in]
              n873 = call "myRIO_BRig_RT_dataExp_Audio_amp__L.vi"() -> ("output_Audio_amp__L"=w1613:i32)  [unwired: 11 in]
              n874 = call "myRIO_BRig_RT_dataExp_Audio_amp__R.vi"() -> ("output_Audio_amp__R"=w1611:i32)  [unwired: 11 in]
              n875 = call "myRIO_BRig_RT_dataExp_TPB_min__L.vi"() -> ("output_TPB_min__L"=w1623:i32)  [unwired: 11 in]
              n876 = call "myRIO_BRig_RT_dataExp_TPB_min__R.vi"() -> ("output_TPB_min__R"=w1621:i32)  [unwired: 11 in]
              n877 = call "myRIO_BRig_RT_dataExp_TPB_max__L.vi"() -> ("output_TPB_max__L"=w1619:i32)  [unwired: 11 in]
              n878 = call "myRIO_BRig_RT_dataExp_TPB_max__R.vi"() -> ("output_TPB_max__R"=w1617:i32)  [unwired: 11 in]
              n879 = call "myRIO_BRig_RT_dataExp_Cue1Param_AudioLed_Count_Switch.vi"() -> ("output_Cue1Param_AudioLed_Count_Switch"=w1585:i32)  [unwired: 11 in]
              n880 = call "myRIO_BRig_RT_dataExp_Cue1Param_AudioLed_Probability_Switch.vi"() -> ("output_Cue1Param_AudioLed_Probability_Switch"=w1583:i32)  [unwired: 11 in]
              n881 = call "myRIO_BRig_RT_dataExp_Cue1Param_CueType_Switch.vi"() -> ("output_Cue1Param_CueType_Switch"=w1581:i32)  [unwired: 11 in]
              n882 = call "myRIO_BRig_RT_dataExp_ItrialUntilReward.vi"() -> ("output_I_trialUntilReward"=w1636:i32)  [unwired: 11 in]
              n883 = call "myRIO_BRig_RT_dataExp_IblockUntilReward.vi"() -> ("output_I_blockUntilReward"=w1632:i32)  [unwired: 11 in]
              n884 = call "myRIO_BRig_RT_dataExp_CueCycles.vi"() -> ("output_CueCycles"=w1631:i32)  [unwired: 11 in]
              n885 = call "myRIO_BRig_RT_dataExp_ENL_min.vi"() -> ("output_ENL_min"=w1629:i32)  [unwired: 11 in]
              n886 = call "myRIO_BRig_RT_dataExp_ENL_max.vi"() -> ("output_ENL_max"=w1627:i32)  [unwired: 11 in]
              n887 = call "myRIO_BRig_RT_dataExp_ENL_penalty.vi"() -> ("output_ENL_penalty"=w1625:i32)  [unwired: 11 in]
              n888 = local read "Audio_Freq__L"() -> (w1589:u8)
              n889 = local read "Audio_Freq__R"() -> (w1587:u8)
              n890 = local read "Audio_Amp__L"() -> (w1612:u16)
              n891 = local read "TpB_Min_L"() -> (w1622:u16)
              n892 = local read "TpB_Min_R"() -> (w1620:u16)
              n893 = local read "TpB_Max_L"() -> (w1618:u16)
              n894 = local read "TpB_Max_R"() -> (w1616:u16)
              n895 = local read "Audio_Amp__R"() -> (w1610:u16)
              n896 = local read "TrialUntilReward"() -> (w1635:bool)
              n897 = local read "CueCycles"() -> (w1630:u16)
              n898 = local read "Tcycle_ENL_min"() -> (w1628:u16)
              n899 = local read "Tcycle_ENL_max"() -> (w1626:u16)
              n900 = local read "Tcycle_ENLPenalty"() -> (w1624:u16)
              n901 = local read "Cue1Param_AudioLed_Count_Switch"() -> (w1584:u16)
              n902 = local read "Cue1Param_AudioLed_Probability_Switch"() -> (w1582:u16)
              n903 = local read "Cue1Param_CueType_Switch"() -> (w1580:u16)
              n904 = To Unsigned Word Integer(number=w1587) -> (unsigned 16bit integer=w1586:u16)
              n905 = To Unsigned Word Integer(number=w1589) -> (unsigned 16bit integer=w1588:u16)
              n906 = Boolean To (0,1)(Boolean=w1635) -> (0, 1=w1634:i16)
              n907 = To Unsigned Word Integer(number=w1634) -> (unsigned 16bit integer=w1633:u16)
              n908 = local read "BUR_min"() -> (w1604:u16)
              n909 = local read "BUR_max"() -> (w1605:u16)
              n910 = Not Equal To 0?(x=w1604) -> (x != 0?=w1603:bool)
              n911 = Not Equal To 0?(x=w1605) -> (x != 0?=w1602:bool)
              n912 = And(x=w1603, y=w1602) -> (x .and. y?=w1601:bool)
              n913 = Boolean To (0,1)(Boolean=w1601) -> (0, 1=w1606:i16)
              n914 = To Unsigned Word Integer(number=w1606) -> (unsigned 16bit integer=w1600:u16)
              n915 = Replace Array Subset(array=w1638, new element #1=w1633, index #1=w1636, new element #2=w1600, index #2=w1632, new element #3=w1630, index #3=w1631, new element #4=w1628, index #4=w1629, new element #5=w1626, index #5=w1627, new element #6=w1624, index #6=w1625, new element #7=w1622, index #7=w1623, new element #8=w1620, index #8=w1621, new element #9=w1618, index #9=w1619, new element #10=w1616, index #10=w1617, new element #11=w1588, index #11=w1615, new element #12=w1586, index #12=w1614, new element #13=w1612, index #13=w1613, new element #14=w1610, index #14=w1611, new element #15=w1584, index #15=w1585, new element #16=w1582, index #16=w1583, new element #17=w1580, index #17=w1581) -> (w1637:u16[])
            }
            frame "saveSettings2" {
              n916 = call "myRIO_BRig_RT_dataExp_Tcycle_Cue1_Audio_min.vi"() -> ("output_Tcycle_Cue1_Audio_min"=w1681:i32)  [unwired: 11 in]
              n917 = call "myRIO_BRig_RT_dataExp_Tcycle_Cue1_Audio_max.vi"() -> ("output_Tcycle_Cue1_Audio_max"=w1680:i32)  [unwired: 11 in]
              n918 = call "myRIO_BRig_RT_dataExp_Tcycle_Cue1Penalty_Audio.vi"() -> ("output_Tcycle_Cue1Penalty_Audio"=w1679:i32)  [unwired: 11 in]
              n919 = call "myRIO_BRig_RT_dataExp_Tcycle_RewardPost.vi"() -> ("output_Tcycle_RewardPost"=w1687:i32)  [unwired: 11 in]
              n920 = call "myRIO_BRig_RT_dataExp_Tcycle_Wrong.vi"() -> ("output_Tcycle_Wrong"=w1685:i32)  [unwired: 11 in]
              n921 = call "myRIO_BRig_RT_dataExp_Tcycle_Timeout.vi"() -> ("output_Tcycle_Timeout"=w1683:i32)  [unwired: 11 in]
              n922 = call "myRIO_BRig_RT_dataExp_SolenoidProbability_L.vi"() -> ("output_SolenoidProbability_L"=w1659:i32)  [unwired: 11 in]
              n923 = call "myRIO_BRig_RT_dataExp_SolenoidProbability_R.vi"() -> ("output_SolenoidProbability_R"=w1658:i32)  [unwired: 11 in]
              n924 = call "myRIO_BRig_RT_dataExp_Cue1Param_AudioLed_Count_NS.vi"() -> ("output_Cue1Param_AudioLed_Count_NS"=w1655:i32)  [unwired: 11 in]
              n925 = call "myRIO_BRig_RT_dataExp_Cue1Param_AudioLed_Probability_NS.vi"() -> ("output_Cue1Param_AudioLed_Probability_NS"=w1653:i32)  [unwired: 11 in]
              n926 = call "myRIO_BRig_RT_dataExp_Cue1Param_CueType_NS.vi"() -> ("output_Cue1Param_CueType_NS"=w1651:i32)  [unwired: 11 in]
              n927 = call "myRIO_BRig_RT_dataExp_nBlock.vi"() -> ("output_nBlock"=w1696:i32)  [unwired: 11 in]
              n928 = call "myRIO_BRig_RT_dataExp_nTrial.vi"() -> ("output_nTrial"=w1695:i32)  [unwired: 11 in]
              n929 = call "myRIO_BRig_RT_dataExp_runTime_seconds.vi"() -> ("output_RunTime_minutes"=w1694:i32)  [unwired: 11 in]
              n930 = call "myRIO_BRig_RT_dataExp_Tcycle_Selection.vi"() -> ("output_Tcycle_Selection"=w1693:i32)  [unwired: 11 in]
              n931 = call "myRIO_BRig_RT_dataExp_Tcycle_Reward__L.vi"() -> ("output_Tcycle_Reward__L"=w1691:i32)  [unwired: 11 in]
              n932 = call "myRIO_BRig_RT_dataExp_Tcycle_Reward__R.vi"() -> ("output_Tcycle_Reward__R"=w1689:i32)  [unwired: 11 in]
              n933 = local read "Tcycle_CuePenalty_Audio"() -> (w1672:u16)
              n934 = call "myRIO_BRig_RT_dataExp_Tcycle_Cue1_LED_min.vi"() -> ("output_Tcycle_Cue1_LED_min"=w1649:i32)  [unwired: 11 in]
              n935 = call "myRIO_BRig_RT_dataExp_Tcycle_Cue1_LED_max.vi"() -> ("output_Tcycle_Cue1_LED_max"=w1648:i32)  [unwired: 11 in]
              n936 = call "myRIO_BRig_RT_dataExp_Tcycle_Cue1Penalty_LED.vi"() -> ("output_Tcycle_Cue1Penalty_LED"=w1647:i32)  [unwired: 11 in]
              n937 = local read "Tcycle_Cue_Audio_max"() -> (w1660:u16)
              n938 = local read "Tcycle_Cue_Audio_min"() -> (w1661:u16)
              n939 = local read "Tcycle_RewardPost"() -> (w1686:u16)
              n940 = local read "Tcycle_Wrong"() -> (w1684:u16)
              n941 = local read "Tcycle_Timeout"() -> (w1682:u16)
              n942 = local read "Tcycle_Selection"() -> (w1692:u16)
              n943 = local read "Tcycle_Reward_L"() -> (w1690:u16)
              n944 = local read "Tcycle_Reward_R"() -> (w1688:u16)
              n945 = local read "Cue1Param_AudioLed_Count_NS"() -> (w1654:u16)
              n946 = local read "Cue1Param_AudioLed_Probability_NS"() -> (w1652:u16)
              n947 = local read "Cue1Param_CueType_NS"() -> (w1650:u16)
              n948 = local read "SolenoidProbability_R"() -> (w1656:u16)
              n949 = local read "SolenoidProbability_L"() -> (w1657:u16)
              n950 = local read "Tcycle_CuePenalty_LED"() -> (w1644:u16)
              n951 = local read "Tcycle_Cue_LED_min"() -> (w1646:u16)
              n952 = local read "Tcycle_Cue_LED_max"() -> (w1645:u16)
              n953 = Replace Array Subset(array=w1698, new element #1=u16 0, index #1=w1696, new element #2=u16 0, index #2=w1695, new element #3=u16 0, index #3=w1694, new element #4=w1692, index #4=w1693, new element #5=w1690, index #5=w1691, new element #6=w1688, index #6=w1689, new element #7=w1686, index #7=w1687, new element #8=w1684, index #8=w1685, new element #9=w1682, index #9=w1683, new element #10=w1661, index #10=w1681, new element #11=w1660, index #11=w1680, new element #12=w1672, index #12=w1679, new element #13=w1657, index #13=w1659, new element #14=w1656, index #14=w1658, new element #15=w1654, index #15=w1655, new element #16=w1652, index #16=w1653, new element #17=w1650, index #17=w1651, new element #18=w1646, index #18=w1649, new element #19=w1645, index #19=w1648, new element #20=w1644, index #20=w1647) -> (w1697:u16[])
            }
            frame "saveSettings3" {
              w1710 = 100.0 ("y")
              n954 = call "myRIO_BRig_RT_dataExp_laser1_Freq.vi"() -> ("output_laser1_Freq"=w1743:i32)  [unwired: 11 in]
              n955 = call "myRIO_BRig_RT_dataExp_laser1_Tpeak.vi"() -> ("output_laser1_Tpeak"=w1738:i32)  [unwired: 11 in]
              n956 = call "myRIO_BRig_RT_dataExp_laser1_Tshutter.vi"() -> ("output_laser1_Tshutter"=w1733:i32)  [unwired: 11 in]
              n957 = call "myRIO_BRig_RT_dataExp_FPGA_f_count2ms.vi"() -> ("output_FPGA_f_count2ms"=w1728:i32)  [unwired: 11 in]
              n958 = call "myRIO_BRig_RT_dataExp_laser1_Power_min.vi"() -> ("output_laser1_Power_min"=w1723:i32)  [unwired: 11 in]
              n959 = call "myRIO_BRig_RT_dataExp_laser1_Power_max.vi"() -> ("output_laser1_Power_max"=w1716:i32)  [unwired: 11 in]
              n960 = call "myRIO_BRig_RT_dataExp_laser1_Power_step.vi"() -> ("output_laser1_Power_step"=w1715:i32)  [unwired: 11 in]
              n961 = call "myRIO_BRig_RT_dataExp_laser1_duration.vi"() -> ("output_laser1_duration"=w1718:i32)  [unwired: 11 in]
              n962 = local read "Laser_Tshutter_l1"() -> (w1730:dbl)
              n963 = local read "Laser_Tpeak_l1"() -> (w1735:dbl)
              n964 = local read "Laser_power_max_l1"() -> (w1709:dbl)
              n965 = local read "Laser_power_step_l1"() -> (w1708:dbl)
              n966 = local read "Laser_power_min_l1"() -> (w1720:dbl)
              n967 = local read "Laser_Freq_l1"() -> (w1742:dbl)
              n968 = call "myRIO_BRig_RT_dataExp_BUR_min.vi"() -> ("output_BUR_min"=w1762:i32)  [unwired: 11 in]
              n969 = call "myRIO_BRig_RT_dataExp_BUR_max.vi"() -> ("output_BUR_max"=w1760:i32)  [unwired: 11 in]
              n970 = call "myRIO_BRig_RT_dataExp_Audio_sp__L.vi"() -> ("output_Audio_sp__L"=w1757:i32)  [unwired: 11 in]
              n971 = call "myRIO_BRig_RT_dataExp_Audio_sp__R.vi"() -> ("output_Audio_sp__R"=w1756:i32)  [unwired: 11 in]
              n972 = local read "FPGA_count2ms"() -> (w1725:dbl)
              n973 = local read "sp_LeftSpout"() -> (w1755:u16)
              n974 = local read "BUR_max"() -> (w1759:u16)
              n975 = local read "sp_RightSpout"() -> (w1754:u16)
              n976 = local read "BUR_min"() -> (w1761:u16)
              n977 = Multiply(x=w1742, y=w1710) -> (x*y=w1741:dbl)
              n978 = Multiply(x=w1735, y=w1710) -> (x*y=w1737:dbl)
              n979 = Multiply(x=w1730, y=w1710) -> (x*y=w1732:dbl)
              n980 = Multiply(x=w1725, y=w1710) -> (x*y=w1727:dbl)
              n981 = Multiply(x=w1720, y=w1710) -> (x*y=w1722:dbl)
              n982 = Multiply(x=w1709, y=w1710) -> (x*y=w1714:dbl)
              n983 = Multiply(x=w1708, y=w1710) -> (x*y=w1712:dbl)
              n984 = Round To Nearest(number=w1741) -> (nearest integer value=w1740:dbl)
              n985 = Round To Nearest(number=w1737) -> (nearest integer value=w1736:dbl)
              n986 = Round To Nearest(number=w1732) -> (nearest integer value=w1731:dbl)
              n987 = Round To Nearest(number=w1727) -> (nearest integer value=w1726:dbl)
              n988 = Round To Nearest(number=w1722) -> (nearest integer value=w1721:dbl)
              n989 = Round To Nearest(number=w1714) -> (nearest integer value=w1713:dbl)
              n990 = Round To Nearest(number=w1712) -> (nearest integer value=w1711:dbl)
              n991 = To Unsigned Word Integer(number=w1740) -> (unsigned 16bit integer=w1739:u16)
              n992 = To Unsigned Word Integer(number=w1736) -> (unsigned 16bit integer=w1734:u16)
              n993 = To Unsigned Word Integer(number=w1731) -> (unsigned 16bit integer=w1729:u16)
              n994 = To Unsigned Word Integer(number=w1726) -> (unsigned 16bit integer=w1724:u16)
              n995 = To Unsigned Word Integer(number=w1721) -> (unsigned 16bit integer=w1719:u16)
              n996 = To Unsigned Word Integer(number=w1713) -> (unsigned 16bit integer=w1707:u16)
              n997 = To Unsigned Word Integer(number=w1711) -> (unsigned 16bit integer=w1706:u16)
              n998 = local read "Laser_duration_l1"() -> (w1717:u16)
              n999 = Replace Array Subset(array=w1763, new element #1=w1761, index #1=w1762, new element #2=w1759, index #2=w1760, new element #3=w1755, index #3=w1757, new element #4=w1754, index #4=w1756, new element #5=w1739, index #5=w1743, new element #6=w1734, index #6=w1738, new element #7=w1729, index #7=w1733, new element #8=w1724, index #8=w1728, new element #9=w1719, index #9=w1723, new element #10=w1707, index #10=w1716, new element #11=w1706, index #11=w1715, new element #12=w1717, index #12=w1718) -> (w1758:u16[])
            }
            frame "saveSettings4" {
              w1783 = 100.0 ("y")
              n1000 = call "myRIO_BRig_RT_dataExp_laser2_Freq.vi"() -> ("output_laser2_Freq"=w1772:i32)  [unwired: 11 in]
              n1001 = call "myRIO_BRig_RT_dataExp_laser2_Tpeak.vi"() -> ("output_laser2_Tpeak"=w1774:i32)  [unwired: 11 in]
              n1002 = call "myRIO_BRig_RT_dataExp_laser2_Tshutter.vi"() -> ("output_laser2_Tshutter"=w1776:i32)  [unwired: 11 in]
              n1003 = call "myRIO_BRig_RT_dataExp_laser2_Power_min.vi"() -> ("output_laser2_Power_min"=w1791:i32)  [unwired: 11 in]
              n1004 = call "myRIO_BRig_RT_dataExp_laser2_Power_max.vi"() -> ("output_laser2_Power_max"=w1790:i32)  [unwired: 11 in]
              n1005 = call "myRIO_BRig_RT_dataExp_laser2_Power_step.vi"() -> ("output_laser2_Power_step"=w1789:i32)  [unwired: 11 in]
              n1006 = call "myRIO_BRig_RT_dataExp_laser2_duration.vi"() -> ("output_laser2_duration"=w1788:i32)  [unwired: 11 in]
              n1007 = call "myRIO_BRig_RT_dataExp_CueLed_Freq.vi"() -> ("output_CueLed_Freq"=w1780:i32)  [unwired: 11 in]
              n1008 = call "myRIO_BRig_RT_dataExp_CueLed_Tpeak.vi"() -> ("output_CueLed_Tpeak"=w1779:i32)  [unwired: 11 in]
              n1009 = local read "Laser_Tshutter_l2"() -> (w1806:dbl)
              n1010 = local read "Laser_Tpeak_l2"() -> (w1809:dbl)
              n1011 = local read "Laser_power_max_l2"() -> (w1796:dbl)
              n1012 = local read "Laser_power_step_l2"() -> (w1795:dbl)
              n1013 = local read "Laser_power_min_l2"() -> (w1803:dbl)
              n1014 = local read "Laser_Freq_l2"() -> (w1814:dbl)
              n1015 = local read "CueLed_Tpeak"() -> (w1781:dbl)
              n1016 = local read "CueLed_Freq"() -> (w1782:dbl)
              n1017 = Multiply(x=w1814, y=w1783) -> (x*y=w1813:dbl)
              n1018 = Multiply(x=w1809, y=w1783) -> (x*y=w1811:dbl)
              n1019 = Multiply(x=w1806, y=w1783) -> (x*y=w1808:dbl)
              n1020 = Multiply(x=w1803, y=w1783) -> (x*y=w1805:dbl)
              n1021 = Multiply(x=w1796, y=w1783) -> (x*y=w1800:dbl)
              n1022 = Multiply(x=w1795, y=w1783) -> (x*y=w1798:dbl)
              n1023 = Multiply(x=w1782, y=w1783) -> (x*y=w1784:dbl)
              n1024 = Multiply(x=w1781, y=w1783) -> (x*y=w1785:dbl)
              n1025 = Round To Nearest(number=w1813) -> (nearest integer value=w1812:dbl)
              n1026 = Round To Nearest(number=w1811) -> (nearest integer value=w1810:dbl)
              n1027 = Round To Nearest(number=w1808) -> (nearest integer value=w1807:dbl)
              n1028 = Round To Nearest(number=w1805) -> (nearest integer value=w1804:dbl)
              n1029 = Round To Nearest(number=w1800) -> (nearest integer value=w1799:dbl)
              n1030 = Round To Nearest(number=w1798) -> (nearest integer value=w1797:dbl)
              n1031 = Round To Nearest(number=w1784) -> (nearest integer value=w1787:dbl)
              n1032 = Round To Nearest(number=w1785) -> (nearest integer value=w1786:dbl)
              n1033 = To Unsigned Word Integer(number=w1812) -> (unsigned 16bit integer=w1771:u16)
              n1034 = To Unsigned Word Integer(number=w1810) -> (unsigned 16bit integer=w1773:u16)
              n1035 = To Unsigned Word Integer(number=w1807) -> (unsigned 16bit integer=w1775:u16)
              n1036 = To Unsigned Word Integer(number=w1804) -> (unsigned 16bit integer=w1802:u16)
              n1037 = To Unsigned Word Integer(number=w1799) -> (unsigned 16bit integer=w1794:u16)
              n1038 = To Unsigned Word Integer(number=w1797) -> (unsigned 16bit integer=w1793:u16)
              n1039 = To Unsigned Word Integer(number=w1787) -> (unsigned 16bit integer=w1778:u16)
              n1040 = To Unsigned Word Integer(number=w1786) -> (unsigned 16bit integer=w1777:u16)
              n1041 = local read "Laser_duration_l2"() -> (w1801:u16)
              n1042 = Replace Array Subset(array=w1826, new element #1=w1771, index #1=w1772, new element #2=w1773, index #2=w1774, new element #3=w1775, index #3=w1776, new element #4=w1802, index #4=w1791, new element #5=w1794, index #5=w1790, new element #6=w1793, index #6=w1789, new element #7=w1801, index #7=w1788, new element #8=w1778, index #8=w1780, new element #9=w1777, index #9=w1779) -> (w1825:u16[])
            }
            frame "saveSettings_LC_ENL_l1" {
              # "Selection First"
              # "Count"
              # "Tdelay"
              # "Probability"
              # "OnOff"
              # "Block"
              # "delayOpt"
              # "Count"
              # "Tdelay"
              # "Probability"
              # "OnOff"
              # "Block"
              # "ENL1 All"
              # "delayOpt"
              # "Count"
              # "Tdelay"
              # "Probability"
              # "OnOff"
              # "Block"
              # "ENL1 First"
              n1043 = local read "LC_ENL1_delayOpt_Switch_l1"() -> (w1864:bool)
              n1044 = call "myRIO_BRig_RT_dataLC_ENL1_Block_NS_l1.vi"() -> ("output_ENL1_All_Block"=w1861:i32)  [unwired: 11 in]
              n1045 = call "myRIO_BRig_RT_dataLC_ENL1_OnOff_NS_l1.vi"() -> ("output_ENL1_OnOff_NS_l1"=w1851:i32)  [unwired: 11 in]
              n1046 = call "myRIO_BRig_RT_dataLC_ENL1_Probability_NS_l1.vi"() -> ("output_ENL1_Probability_NS_l1"=w1850:i32)  [unwired: 11 in]
              n1047 = call "myRIO_BRig_RT_dataLC_ENL1_Tdelay_NS_l1.vi"() -> ("output_ENL1_Tdelay_NS_l1"=w1849:i32)  [unwired: 11 in]
              n1048 = call "myRIO_BRig_RT_dataLC_ENL1_Count_NS_l1.vi"() -> ("output_ENL1_Count_NS_l1"=w1848:i32)  [unwired: 11 in]
              n1049 = call "myRIO_BRig_RT_dataLC_ENL1_delayOpt_NS_l1.vi"() -> ("output_ENL1_delayOpt_NS_l1"=w1847:i32)  [unwired: 11 in]
              n1050 = call "myRIO_BRig_RT_dataLC_ENL1_Block_Switch_l1.vi"() -> ("output_ENL1_Block_Switch_l1"=w1887:i32)  [unwired: 11 in]
              n1051 = call "myRIO_BRig_RT_dataLC_ENL1_OnOff_Switch_l1.vi"() -> ("output_ENL1_OnOff_Switch_l1"=w1885:i32)  [unwired: 11 in]
              n1052 = call "myRIO_BRig_RT_dataLC_ENL1_Probability_Switch_l1.vi"() -> ("output_ENL1_Probability_Switch_l1"=w1881:i32)  [unwired: 11 in]
              n1053 = call "myRIO_BRig_RT_dataLC_ENL1_Tdelay_Switch_l1.vi"() -> ("output_ENL1_Tdelay_Switch_l1"=w1879:i32)  [unwired: 11 in]
              n1054 = call "myRIO_BRig_RT_dataLC_ENL1_Count_Switch_l1.vi"() -> ("output_ENL1_Count_Switch_l1"=w1877:i32)  [unwired: 11 in]
              n1055 = call "myRIO_BRig_RT_dataLC_ENL1_delayOpt_Switch_l1.vi"() -> ("output_ENL1_delayOpt_Switch_l1"=w1863:i32)  [unwired: 11 in]
              n1056 = local read "LC_ENL1_Count_Switch_l1"() -> (w1876:u16)
              n1057 = local read "LC_ENL1_Probability_Switch_l1"() -> (w1880:u16)
              n1058 = local read "LC_ENL1_Block_Switch_l1"() -> (w1886:u16)
              n1059 = local read "LC_ENL1_Tdelay_Switch_l1"() -> (w1878:u16)
              n1060 = local read "LC_ENL1_OnOff_Switch_l1"() -> (w1884:bool)
              n1061 = call "myRIO_BRig_RT_dataLC_Selection_Block_Switch_l1.vi"() -> ("output_Selection_Block_Switch_l1"=w1845:i32)  [unwired: 11 in]
              n1062 = call "myRIO_BRig_RT_dataLC_Selection_OnOff_Switch_l1.vi"() -> ("output_Selection_OnOff_Switch_l1"=w1844:i32)  [unwired: 11 in]
              n1063 = call "myRIO_BRig_RT_dataLC_Selection_Probability_Switch_l1.vi"() -> ("output_Selection_Probability_Switch_l1"=w1843:i32)  [unwired: 11 in]
              n1064 = call "myRIO_BRig_RT_dataLC_Selection_Tdelay_Switch_l1.vi"() -> ("output_Selection_Tdelay_Switch_l1"=w1842:i32)  [unwired: 11 in]
              n1065 = call "myRIO_BRig_RT_dataLC_Selection_Count_Switch_l1.vi"() -> ("output_Selection_Count_Switch_l1"=w1841:i32)  [unwired: 11 in]
              n1066 = local read "LC_ENL1_OnOff_NS_l1"() -> (w1857:bool)
              n1067 = local read "LC_ENL1_Probability_NS_l1"() -> (w1855:u16)
              n1068 = local read "LC_ENL1_delayOpt_NS_l1"() -> (w1853:bool)
              n1069 = local read "LC_Sel_Probability_Switch_l1"() -> (w1836:u16)
              n1070 = local read "LC_ENL1_Tdelay_NS_l1"() -> (w1846:u16)
              n1071 = local read "LC_ENL1_Block_NS_l1"() -> (w1858:u16)
              n1072 = local read "LC_ENL1_Count_NS_l1"() -> (w1854:u16)
              n1073 = local read "LC_Sel_Tdelay_Switch_l1"() -> (w1835:u16)
              n1074 = local read "LC_Sel_OnOff_Switch_l1"() -> (w1839:bool)
              n1075 = local read "LC_Sel_Count_Switch_l1"() -> (w1834:u16)
              n1076 = local read "LC_Sel_Block_Switch_l1"() -> (w1838:u16)
              n1077 = Boolean To (0,1)(Boolean=w1864) -> (0, 1=w1865:i16)
              n1078 = Boolean To (0,1)(Boolean=w1884) -> (0, 1=w1883:i16)
              n1079 = Boolean To (0,1)(Boolean=w1857) -> (0, 1=w1860:i16)
              n1080 = To Unsigned Word Integer(number=w1865) -> (unsigned 16bit integer=w1862:u16)
              n1081 = To Unsigned Word Integer(number=w1883) -> (unsigned 16bit integer=w1882:u16)
              n1082 = Boolean To (0,1)(Boolean=w1853) -> (0, 1=w1859:i16)
              n1083 = To Unsigned Word Integer(number=w1860) -> (unsigned 16bit integer=w1856:u16)
              n1084 = Boolean To (0,1)(Boolean=w1839) -> (0, 1=w1840:i16)
              n1085 = To Unsigned Word Integer(number=w1859) -> (unsigned 16bit integer=w1852:u16)
              n1086 = To Unsigned Word Integer(number=w1840) -> (unsigned 16bit integer=w1837:u16)
              n1087 = Replace Array Subset(array=w1888, new element #1=w1886, index #1=w1887, new element #2=w1882, index #2=w1885, new element #3=w1880, index #3=w1881, new element #4=w1878, index #4=w1879, new element #5=w1876, index #5=w1877, new element #6=w1862, index #6=w1863, new element #7=w1858, index #7=w1861, new element #8=w1856, index #8=w1851, new element #9=w1855, index #9=w1850, new element #10=w1846, index #10=w1849, new element #11=w1854, index #11=w1848, new element #12=w1852, index #12=w1847, new element #13=w1838, index #13=w1845, new element #14=w1837, index #14=w1844, new element #15=w1836, index #15=w1843, new element #16=w1835, index #16=w1842, new element #17=w1834, index #17=w1841) -> (w1889:u16[])
            }
            frame "saveSettings_LC_ENL_l2" {
              # "Selection First"
              # "Count"
              # "Tdelay"
              # "Probability"
              # "OnOff"
              # "Block"
              # "delayOpt"
              # "Count"
              # "Tdelay"
              # "Probability"
              # "OnOff"
              # "Block"
              # "ENL1 All"
              # "delayOpt"
              # "Count"
              # "Tdelay"
              # "Probability"
              # "OnOff"
              # "Block"
              # "ENL1 First"
              n1088 = call "myRIO_BRig_RT_dataLC_ENL1_Block_Switch_l2.vi"() -> ("output_ENL1_Block_Switch_l2"=w1908:i32)  [unwired: 11 in]
              n1089 = call "myRIO_BRig_RT_dataLC_ENL1_OnOff_Switch_l2.vi"() -> ("output_ENL1_OnOff_Switch_l2"=w1909:i32)  [unwired: 11 in]
              n1090 = call "myRIO_BRig_RT_dataLC_ENL1_Probability_Switch_l2.vi"() -> ("output_ENL1_Probability_Switch_l2"=w1910:i32)  [unwired: 11 in]
              n1091 = call "myRIO_BRig_RT_dataLC_ENL1_Tdelay_Switch_l2.vi"() -> ("output_ENL1_Tdelay_Switch_l2"=w1911:i32)  [unwired: 11 in]
              n1092 = call "myRIO_BRig_RT_dataLC_ENL1_Count_Switch_l2.vi"() -> ("output_ENL1_Count_Switch_l2"=w1912:i32)  [unwired: 11 in]
              n1093 = call "myRIO_BRig_RT_dataLC_ENL1_delayOpt_Switch_l2.vi"() -> ("output_ENL1_delayOpt_Switch_l2"=w1913:i32)  [unwired: 11 in]
              n1094 = local read "LC_ENL1_delayOpt_Switch_l2"() -> (w1933:bool)
              n1095 = call "myRIO_BRig_RT_dataLC_ENL1_Block_NS_l2.vi"() -> ("output_ENL1_Block_NS_l2"=w1902:i32)  [unwired: 11 in]
              n1096 = call "myRIO_BRig_RT_dataLC_ENL1_OnOff_NS_l2.vi"() -> ("output_ENL1_OnOff_NS_l2"=w1903:i32)  [unwired: 11 in]
              n1097 = call "myRIO_BRig_RT_dataLC_ENL1_Probability_NS_l2.vi"() -> ("output_ENL1_Probability_NS_l2"=w1904:i32)  [unwired: 11 in]
              n1098 = call "myRIO_BRig_RT_dataLC_ENL1_Tdelay_NS_l2.vi"() -> ("output_ENL1_Tdelay_NS_l2"=w1905:i32)  [unwired: 11 in]
              n1099 = call "myRIO_BRig_RT_dataLC_ENL1_Count_NS_l2.vi"() -> ("output_ENL1_Count_NS_l2"=w1906:i32)  [unwired: 11 in]
              n1100 = call "myRIO_BRig_RT_dataLC_ENL1_delayOpt_NS_l2.vi"() -> ("output_ENL1_delayOpt_NS_l2"=w1907:i32)  [unwired: 11 in]
              n1101 = local read "LC_ENL1_Count_Switch_l2"() -> (w1945:u16)
              n1102 = local read "LC_ENL1_Probability_Switch_l2"() -> (w1947:u16)
              n1103 = local read "LC_ENL1_Block_Switch_l2"() -> (w1951:u16)
              n1104 = local read "LC_ENL1_Tdelay_Switch_l2"() -> (w1946:u16)
              n1105 = local read "LC_ENL1_OnOff_Switch_l2"() -> (w1950:bool)
              n1106 = call "myRIO_BRig_RT_dataLC_Selection_Block_Switch_l2.vi"() -> ("output_Selection_Block_Switch_l2"=w1901:i32)  [unwired: 11 in]
              n1107 = call "myRIO_BRig_RT_dataLC_Selection_OnOff_Switch_l2.vi"() -> ("output_Selection_OnOff_Switch_l2"=w1900:i32)  [unwired: 11 in]
              n1108 = call "myRIO_BRig_RT_dataLC_Selection_Probability_Switch_l2.vi"() -> ("output_Selection_Probability_Switch_l1"=w1899:i32)  [unwired: 11 in]
              n1109 = call "myRIO_BRig_RT_dataLC_Selection_Tdelay_Switch_l2.vi"() -> ("output_Selection_Tdelay_Switch_l2"=w1898:i32)  [unwired: 11 in]
              n1110 = call "myRIO_BRig_RT_dataLC_Selection_Count_Switch_l2.vi"() -> ("output_Selection_Count_Switch_l2"=w1897:i32)  [unwired: 11 in]
              n1111 = local read "LC_ENL1_OnOff_NS_l2"() -> (w1928:bool)
              n1112 = local read "LC_ENL1_Probability_NS_l2"() -> (w1926:u16)
              n1113 = local read "LC_ENL1_delayOpt_NS_l2"() -> (w1924:bool)
              n1114 = local read "LC_Sel_Probability_Switch_l2"() -> (w1917:u16)
              n1115 = local read "LC_ENL1_Tdelay_NS_l2"() -> (w1922:u16)
              n1116 = local read "LC_ENL1_Block_NS_l2"() -> (w1929:u16)
              n1117 = local read "LC_ENL1_Count_NS_l2"() -> (w1925:u16)
              n1118 = local read "LC_Sel_Tdelay_Switch_l2"() -> (w1916:u16)
              n1119 = local read "LC_Sel_OnOff_Switch_l2"() -> (w1920:bool)
              n1120 = local read "LC_Sel_Count_Switch_l2"() -> (w1915:u16)
              n1121 = local read "LC_Sel_Block_Switch_l2"() -> (w1919:u16)
              n1122 = Boolean To (0,1)(Boolean=w1933) -> (0, 1=w1934:i16)
              n1123 = Boolean To (0,1)(Boolean=w1950) -> (0, 1=w1949:i16)
              n1124 = Boolean To (0,1)(Boolean=w1928) -> (0, 1=w1931:i16)
              n1125 = To Unsigned Word Integer(number=w1934) -> (unsigned 16bit integer=w1932:u16)
              n1126 = To Unsigned Word Integer(number=w1949) -> (unsigned 16bit integer=w1948:u16)
              n1127 = Boolean To (0,1)(Boolean=w1924) -> (0, 1=w1930:i16)
              n1128 = To Unsigned Word Integer(number=w1931) -> (unsigned 16bit integer=w1927:u16)
              n1129 = Boolean To (0,1)(Boolean=w1920) -> (0, 1=w1921:i16)
              n1130 = To Unsigned Word Integer(number=w1930) -> (unsigned 16bit integer=w1923:u16)
              n1131 = To Unsigned Word Integer(number=w1921) -> (unsigned 16bit integer=w1918:u16)
              n1132 = Replace Array Subset(array=w1952, new element #1=w1951, index #1=w1908, new element #2=w1948, index #2=w1909, new element #3=w1947, index #3=w1910, new element #4=w1946, index #4=w1911, new element #5=w1945, index #5=w1912, new element #6=w1932, index #6=w1913, new element #7=w1929, index #7=w1902, new element #8=w1927, index #8=w1903, new element #9=w1926, index #9=w1904, new element #10=w1922, index #10=w1905, new element #11=w1925, index #11=w1906, new element #12=w1923, index #12=w1907, new element #13=w1919, index #13=w1901, new element #14=w1918, index #14=w1900, new element #15=w1917, index #15=w1899, new element #16=w1916, index #16=w1898, new element #17=w1915, index #17=w1897) -> (w1953:u16[])
            }
            frame "saveSettings_LC_Cue_l1" {
              # "Selection All"
              # "Count"
              # "Tdelay"
              # "Probability"
              # "OnOff"
              # "Block"
              # "delayOpt"
              # "Count"
              # "Tdelay"
              # "Probability"
              # "OnOff"
              # "Block"
              # "Cue1 All"
              # "delayOpt"
              # "Count"
              # "Tdelay"
              # "Probability"
              # "OnOff"
              # "Block"
              # "Cue1 First"
              n1133 = call "myRIO_BRig_RT_dataLC_Cue1_delayOpt_Switch_l1.vi"() -> ("output_Cue1_delayOpt_Switch_l1"=w1992:i32)  [unwired: 11 in]
              n1134 = call "myRIO_BRig_RT_dataLC_Cue1_Block_Switch_l1.vi"() -> ("output_Cue1_Block_Switch_l1"=w2015:i32)  [unwired: 11 in]
              n1135 = call "myRIO_BRig_RT_dataLC_Cue1_OnOff_Switch_l1.vi"() -> ("output_Cue1_OnOff_Switch_l1"=w2013:i32)  [unwired: 11 in]
              n1136 = call "myRIO_BRig_RT_dataLC_Cue1_Probability_Switch_l1.vi"() -> ("output_Cue1_Probability_Switch_l1"=w2009:i32)  [unwired: 11 in]
              n1137 = call "myRIO_BRig_RT_dataLC_Cue1_Tdelay_Switch_l1.vi"() -> ("output_Cue1_Tdelay_Switch_l1"=w2007:i32)  [unwired: 11 in]
              n1138 = call "myRIO_BRig_RT_dataLC_Cue1_Count_Switch_l1.vi"() -> ("output_Cue1_Count_Switch_l1"=w2005:i32)  [unwired: 11 in]
              n1139 = local read "LC_Cue1_delayOpt_Switch_l1"() -> (w1991:bool)
              n1140 = call "myRIO_BRig_RT_dataLC_Cue1_Block_NS_l1.vi"() -> ("output_Cue1_Block_NS_l1"=w1989:i32)  [unwired: 11 in]
              n1141 = call "myRIO_BRig_RT_dataLC_Cue1_OnOff_NS_l1.vi"() -> ("output_Cue1_OnOff_NS_l1"=w1988:i32)  [unwired: 11 in]
              n1142 = call "myRIO_BRig_RT_dataLC_Cue1_Probability_NS_l1.vi"() -> ("output_Cue1_l1_All_Probability"=w1987:i32)  [unwired: 11 in]
              n1143 = call "myRIO_BRig_RT_dataLC_Cue1_Tdelay_NS_l1.vi"() -> ("output_Cue1_Tdelay_NS_l1"=w1986:i32)  [unwired: 11 in]
              n1144 = call "myRIO_BRig_RT_dataLC_Cue1_Count_NS_l1.vi"() -> ("output_Cue1_Count_NS_l1"=w1985:i32)  [unwired: 11 in]
              n1145 = call "myRIO_BRig_RT_dataLC_Cue1_delayOpt_NS_l1.vi"() -> ("output_Cue1_delayOpt_NS_l1"=w1984:i32)  [unwired: 11 in]
              n1146 = local read "LC_Cue1_Count_Switch_l1"() -> (w2004:u16)
              n1147 = local read "LC_Cue1_Probability_Switch_l1"() -> (w2008:u16)
              n1148 = local read "LC_Cue1_Block_Switch_l1"() -> (w2014:u16)
              n1149 = local read "LC_Cue1_Tdelay_Switch_l1"() -> (w2006:u16)
              n1150 = local read "LC_Cue1_OnOff_Switch_l1"() -> (w2012:bool)
              n1151 = local read "LC_Cue1_OnOff_NS_l1"() -> (w1980:bool)
              n1152 = call "myRIO_BRig_RT_dataLC_Selection_Block_NS_l1.vi"() -> ("output_Selection_Block_NS_l1"=w1973:i32)  [unwired: 11 in]
              n1153 = call "myRIO_BRig_RT_dataLC_Selection_OnOff_NS_l1.vi"() -> ("output_Selection_OnOff_NS_l1"=w1972:i32)  [unwired: 11 in]
              n1154 = call "myRIO_BRig_RT_dataLC_Selection_Probability_NS_l1.vi"() -> ("output_Selection_Probability_NS_l1"=w1971:i32)  [unwired: 11 in]
              n1155 = call "myRIO_BRig_RT_dataLC_Selection_Tdelay_NS_l1.vi"() -> ("output_Selection_Tdelay_NS_l1"=w1970:i32)  [unwired: 11 in]
              n1156 = call "myRIO_BRig_RT_dataLC_Selection_Count_NS_l1.vi"() -> ("output_Selection_Count_NS_l1"=w1963:i32)  [unwired: 11 in]
              n1157 = local read "LC_Cue1_delayOpt_NS_l1"() -> (w1981:bool)
              n1158 = local read "LC_Cue1_Probability_NS_l1"() -> (w1977:u16)
              n1159 = local read "LC_Cue1_Tdelay_NS_l1"() -> (w1976:u16)
              n1160 = local read "LC_Cue1_Count_NS_l1"() -> (w1975:u16)
              n1161 = local read "LC_Cue1_Block_NS_l1"() -> (w1979:u16)
              n1162 = local read "LC_Sel_Probability_NS_l1"() -> (w1965:u16)
              n1163 = local read "LC_Sel_Tdelay_NS_l1"() -> (w1964:u16)
              n1164 = local read "LC_Sel_OnOff_NS_l1"() -> (w1967:bool)
              n1165 = local read "LC_Sel_Count_NS_l1"() -> (w1962:u16)
              n1166 = local read "LC_Sel_Block_NS_l1"() -> (w1969:u16)
              n1167 = Boolean To (0,1)(Boolean=w1991) -> (0, 1=w1993:i16)
              n1168 = Boolean To (0,1)(Boolean=w2012) -> (0, 1=w2011:i16)
              n1169 = Boolean To (0,1)(Boolean=w1980) -> (0, 1=w1983:i16)
              n1170 = To Unsigned Word Integer(number=w1993) -> (unsigned 16bit integer=w1990:u16)
              n1171 = To Unsigned Word Integer(number=w2011) -> (unsigned 16bit integer=w2010:u16)
              n1172 = To Unsigned Word Integer(number=w1983) -> (unsigned 16bit integer=w1978:u16)
              n1173 = Boolean To (0,1)(Boolean=w1981) -> (0, 1=w1982:i16)
              n1174 = Boolean To (0,1)(Boolean=w1967) -> (0, 1=w1968:i16)
              n1175 = To Unsigned Word Integer(number=w1982) -> (unsigned 16bit integer=w1974:u16)
              n1176 = To Unsigned Word Integer(number=w1968) -> (unsigned 16bit integer=w1966:u16)
              n1177 = Replace Array Subset(array=w2016, new element #1=w2014, index #1=w2015, new element #2=w2010, index #2=w2013, new element #3=w2008, index #3=w2009, new element #4=w2006, index #4=w2007, new element #5=w2004, index #5=w2005, new element #6=w1990, index #6=w1992, new element #7=w1979, index #7=w1989, new element #8=w1978, index #8=w1988, new element #9=w1977, index #9=w1987, new element #10=w1976, index #10=w1986, new element #11=w1975, index #11=w1985, new element #12=w1974, index #12=w1984, new element #13=w1969, index #13=w1973, new element #14=w1966, index #14=w1972, new element #15=w1965, index #15=w1971, new element #16=w1964, index #16=w1970, new element #17=w1962, index #17=w1963) -> (w2017:u16[])
            }
            frame "saveSettings_LC_Cue_l2" {
              # "Selection All"
              # "Count"
              # "Tdelay"
              # "Probability"
              # "OnOff"
              # "Block"
              # "delayOpt"
              # "Count"
              # "Tdelay"
              # "Probability"
              # "OnOff"
              # "Block"
              # "Cue1 All"
              # "delayOpt"
              # "Count"
              # "Tdelay"
              # "Probability"
              # "OnOff"
              # "Block"
              # "Cue1 First"
              n1178 = call "myRIO_BRig_RT_dataLC_Cue1_delayOpt_Switch_l2.vi"() -> ("output_Cue1_delayOpt_Switch_l2"=w2056:i32)  [unwired: 11 in]
              n1179 = call "myRIO_BRig_RT_dataLC_Cue1_Block_Switch_l2.vi"() -> ("output_Cue1_Block_Switch_l2"=w2079:i32)  [unwired: 11 in]
              n1180 = call "myRIO_BRig_RT_dataLC_Cue1_OnOff_Switch_l2.vi"() -> ("output_Cue1_OnOff_Switch_l2"=w2077:i32)  [unwired: 11 in]
              n1181 = call "myRIO_BRig_RT_dataLC_Cue1_Probability_Switch_l2.vi"() -> ("output_Cue1_l2_First_Probability"=w2073:i32)  [unwired: 11 in]
              n1182 = call "myRIO_BRig_RT_dataLC_Cue1_Tdelay_Switch_l2.vi"() -> ("output_Cue1_Tdelay_Switch_l2"=w2071:i32)  [unwired: 11 in]
              n1183 = call "myRIO_BRig_RT_dataLC_Cue1_Count_Switch_l2.vi"() -> ("output_Cue1_Count_Switch_l2"=w2069:i32)  [unwired: 11 in]
              n1184 = local read "LC_Cue1_delayOpt_Switch_l2"() -> (w2055:bool)
              n1185 = call "myRIO_BRig_RT_dataLC_Cue1_Block_NS_l2.vi"() -> ("output_Cue1_Block_NS_l2"=w2053:i32)  [unwired: 11 in]
              n1186 = call "myRIO_BRig_RT_dataLC_Cue1_OnOff_NS_l2.vi"() -> ("output_Cue1_OnOff_NS_l2"=w2052:i32)  [unwired: 11 in]
              n1187 = call "myRIO_BRig_RT_dataLC_Cue1_Probability_NS_l2.vi"() -> ("output_Cue1_l2_All_Probability"=w2051:i32)  [unwired: 11 in]
              n1188 = call "myRIO_BRig_RT_dataLC_Cue1_Tdelay_NS_l2.vi"() -> ("output_Cue1_Tdelay_NS_l2"=w2050:i32)  [unwired: 11 in]
              n1189 = call "myRIO_BRig_RT_dataLC_Cue1_Count_NS_l2.vi"() -> ("output_Cue1_Count_NS_l2"=w2049:i32)  [unwired: 11 in]
              n1190 = call "myRIO_BRig_RT_dataLC_Cue1_delayOpt_NS_l2.vi"() -> ("output_Cue1_delayOpt_NS_l2"=w2048:i32)  [unwired: 11 in]
              n1191 = local read "LC_Cue1_Count_Switch_l2"() -> (w2068:u16)
              n1192 = local read "LC_Cue1_Probability_Switch_l2"() -> (w2072:u16)
              n1193 = local read "LC_Cue1_Block_Switch_l2"() -> (w2078:u16)
              n1194 = local read "LC_Cue1_Tdelay_Switch_l2"() -> (w2070:u16)
              n1195 = local read "LC_Cue1_OnOff_Switch_l2"() -> (w2076:bool)
              n1196 = local read "LC_Cue1_OnOff_NS_l2"() -> (w2044:bool)
              n1197 = call "myRIO_BRig_RT_dataLC_Selection_Block_NS_l2.vi"() -> ("output_Selection_Block_NS_l2"=w2029:i32)  [unwired: 11 in]
              n1198 = call "myRIO_BRig_RT_dataLC_Selection_OnOff_NS_l2.vi"() -> ("output_Selection_OnOff_NS_l2"=w2028:i32)  [unwired: 11 in]
              n1199 = call "myRIO_BRig_RT_dataLC_Selection_Probability_NS_l2.vi"() -> ("output_Selection_Probability_NS_l2"=w2027:i32)  [unwired: 11 in]
              n1200 = call "myRIO_BRig_RT_dataLC_Selection_Tdelay_NS_l2.vi"() -> ("output_Selection_Tdelay_NS_l2"=w2026:i32)  [unwired: 11 in]
              n1201 = call "myRIO_BRig_RT_dataLC_Selection_Count_NS_l2.vi"() -> ("output_Selection_Count_NS_l2"=w2025:i32)  [unwired: 11 in]
              n1202 = local read "LC_Cue1_delayOpt_NS_l2"() -> (w2045:bool)
              n1203 = local read "LC_Cue1_Probability_NS_l2"() -> (w2041:u16)
              n1204 = local read "LC_Cue1_Tdelay_NS_l2"() -> (w2040:u16)
              n1205 = local read "LC_Cue1_Count_NS_l2"() -> (w2039:u16)
              n1206 = local read "LC_Cue1_Block_NS_l2"() -> (w2043:u16)
              n1207 = local read "LC_Sel_Probability_NS_l2"() -> (w2033:u16)
              n1208 = local read "LC_Sel_Tdelay_NS_l2"() -> (w2032:u16)
              n1209 = local read "LC_Sel_OnOff_NS_l2"() -> (w2035:bool)
              n1210 = local read "LC_Sel_Count_NS_l2"() -> (w2031:u16)
              n1211 = local read "LC_Sel_Block_NS_l2"() -> (w2037:u16)
              n1212 = Boolean To (0,1)(Boolean=w2055) -> (0, 1=w2057:i16)
              n1213 = Boolean To (0,1)(Boolean=w2076) -> (0, 1=w2075:i16)
              n1214 = Boolean To (0,1)(Boolean=w2044) -> (0, 1=w2047:i16)
              n1215 = To Unsigned Word Integer(number=w2057) -> (unsigned 16bit integer=w2054:u16)
              n1216 = To Unsigned Word Integer(number=w2075) -> (unsigned 16bit integer=w2074:u16)
              n1217 = To Unsigned Word Integer(number=w2047) -> (unsigned 16bit integer=w2042:u16)
              n1218 = Boolean To (0,1)(Boolean=w2045) -> (0, 1=w2046:i16)
              n1219 = Boolean To (0,1)(Boolean=w2035) -> (0, 1=w2036:i16)
              n1220 = To Unsigned Word Integer(number=w2046) -> (unsigned 16bit integer=w2038:u16)
              n1221 = To Unsigned Word Integer(number=w2036) -> (unsigned 16bit integer=w2034:u16)
              n1222 = Replace Array Subset(array=w2080, new element #1=w2078, index #1=w2079, new element #2=w2074, index #2=w2077, new element #3=w2072, index #3=w2073, new element #4=w2070, index #4=w2071, new element #5=w2068, index #5=w2069, new element #6=w2054, index #6=w2056, new element #7=w2043, index #7=w2053, new element #8=w2042, index #8=w2052, new element #9=w2041, index #9=w2051, new element #10=w2040, index #10=w2050, new element #11=w2039, index #11=w2049, new element #12=w2038, index #12=w2048, new element #13=w2037, index #13=w2029, new element #14=w2034, index #14=w2028, new element #15=w2033, index #15=w2027, new element #16=w2032, index #16=w2026, new element #17=w2031, index #17=w2025) -> (w2081:u16[])
            }
            frame "saveSettings6_LC_l1_Other" {
              # "Trial"
              # "Tdelay"
              # "Probability"
              # "OnOff"
              # "Block"
              # "Wrong"
              # "Trial"
              # "Tdelay"
              # "Probability"
              # "OnOff"
              # "Block"
              # "Reward"
              n1223 = call "myRIO_BRig_RT_dataLC_Wrong_Block_l1.vi"() -> ("output_Wrong_Block_l1"=w2110:i32)  [unwired: 11 in]
              n1224 = call "myRIO_BRig_RT_dataLC_Wrong_OnOff_l1.vi"() -> ("output_Wrong_OnOff_l1"=w2109:i32)  [unwired: 11 in]
              n1225 = call "myRIO_BRig_RT_dataLC_Wrong_Probability_l1.vi"() -> ("output_Wrong_Probability_l1"=w2108:i32)  [unwired: 11 in]
              n1226 = call "myRIO_BRig_RT_dataLC_Wrong_Tdelay_l1.vi"() -> ("output_Wrong_Tdelay_l1"=w2107:i32)  [unwired: 11 in]
              n1227 = call "myRIO_BRig_RT_dataLC_Wrong_Trial_l1.vi"() -> ("output_Wrong_Trial_l1"=w2106:i32)  [unwired: 11 in]
              n1228 = call "myRIO_BRig_RT_dataLC_Reward_Block_l1.vi"() -> ("output_Reward_Block_l1"=w2122:i32)  [unwired: 11 in]
              n1229 = call "myRIO_BRig_RT_dataLC_Reward_OnOff_l1.vi"() -> ("output_Reward_OnOff_l1"=w2120:i32)  [unwired: 11 in]
              n1230 = call "myRIO_BRig_RT_dataLC_Reward_Probability_l1.vi"() -> ("output_Reward_Probability_l1"=w2116:i32)  [unwired: 11 in]
              n1231 = call "myRIO_BRig_RT_dataLC_Reward_Tdelay_l1.vi"() -> ("output_Reward_Tdelay_l1"=w2114:i32)  [unwired: 11 in]
              n1232 = call "myRIO_BRig_RT_dataLC_Reward_Trial_l1.vi"() -> ("output_Reward_Trial_l1"=w2112:i32)  [unwired: 11 in]
              n1233 = local read "LC_Wrong_OnOff_l1"() -> (w2104:bool)
              n1234 = local read "LC_Wrong_Probability_l1"() -> (w2101:u16)
              n1235 = local read "LC_Wrong_Block_l1"() -> (w2103:u16)
              n1236 = local read "LC_Wrong_Tdelay_l1"() -> (w2100:u16)
              n1237 = local read "LC_Wrong_Trial_l1"() -> (w2099:u16)
              n1238 = local read "LC_Reward_Probability_l1"() -> (w2115:u16)
              n1239 = local read "LC_Reward_Block_l1"() -> (w2121:u16)
              n1240 = local read "LC_Reward_Tdelay_l1"() -> (w2113:u16)
              n1241 = local read "LC_Reward_OnOff_l1"() -> (w2119:bool)
              n1242 = local read "LC_Reward_Trial_l1"() -> (w2111:u16)
              n1243 = Boolean To (0,1)(Boolean=w2104) -> (0, 1=w2105:i16)
              n1244 = Boolean To (0,1)(Boolean=w2119) -> (0, 1=w2118:i16)
              n1245 = To Unsigned Word Integer(number=w2105) -> (unsigned 16bit integer=w2102:u16)
              n1246 = To Unsigned Word Integer(number=w2118) -> (unsigned 16bit integer=w2117:u16)
              n1247 = Replace Array Subset(array=w2123, new element #1=w2121, index #1=w2122, new element #2=w2117, index #2=w2120, new element #3=w2115, index #3=w2116, new element #4=w2113, index #4=w2114, new element #5=w2111, index #5=w2112, new element #6=w2103, index #6=w2110, new element #7=w2102, index #7=w2109, new element #8=w2101, index #8=w2108, new element #9=w2100, index #9=w2107, new element #10=w2099, index #10=w2106) -> (w2124:u16[])
            }
            frame "SaveSettings6_LC_l2_Other" {
              # "Trial"
              # "Tdelay"
              # "Probability"
              # "OnOff"
              # "Block"
              # "Wrong"
              # "Trial"
              # "Tdelay"
              # "Probability"
              # "OnOff"
              # "Block"
              # "Reward"
              n1248 = call "myRIO_BRig_RT_dataLC_Wrong_Block_l2.vi"() -> ("output_Wrong_Block_l2"=w2133:i32)  [unwired: 11 in]
              n1249 = call "myRIO_BRig_RT_dataLC_Wrong_OnOff_l2.vi"() -> ("output_Wrong_OnOff_l2"=w2134:i32)  [unwired: 11 in]
              n1250 = call "myRIO_BRig_RT_dataLC_Wrong_Probability_l2.vi"() -> ("output_Wrong_Probability_l2"=w2135:i32)  [unwired: 11 in]
              n1251 = call "myRIO_BRig_RT_dataLC_Wrong_Tdelay_l2.vi"() -> ("output_Wrong_Tdelay_l2"=w2136:i32)  [unwired: 11 in]
              n1252 = call "myRIO_BRig_RT_dataLC_Wrong_Trial_l2.vi"() -> ("output_Wrong_Trial_l2"=w2137:i32)  [unwired: 11 in]
              n1253 = call "myRIO_BRig_RT_dataLC_Reward_Block_l2.vi"() -> ("output_Reward_Block_l2"=w2138:i32)  [unwired: 11 in]
              n1254 = call "myRIO_BRig_RT_dataLC_Reward_OnOff_l2.vi"() -> ("output_Reward_OnOff_l2"=w2139:i32)  [unwired: 11 in]
              n1255 = call "myRIO_BRig_RT_dataLC_Reward_Probability_l2.vi"() -> ("output_Reward_Probability_l2"=w2140:i32)  [unwired: 11 in]
              n1256 = call "myRIO_BRig_RT_dataLC_Reward_Tdelay_l2.vi"() -> ("output_Reward_Tdelay_l2"=w2141:i32)  [unwired: 11 in]
              n1257 = call "myRIO_BRig_RT_dataLC_Reward_Trial_l2.vi"() -> ("output_Reward_Trial_l2"=w2142:i32)  [unwired: 11 in]
              n1258 = local read "LC_Wrong_OnOff_l2"() -> (w2158:bool)
              n1259 = local read "LC_Wrong_Probability_l2"() -> (w2155:u16)
              n1260 = local read "LC_Wrong_Block_l2"() -> (w2157:u16)
              n1261 = local read "LC_Wrong_Tdelay_l2"() -> (w2154:u16)
              n1262 = local read "LC_Wrong_Trial_l2"() -> (w2153:u16)
              n1263 = local read "LC_Reward_Probability_l2"() -> (w2162:u16)
              n1264 = local read "LC_Reward_Block_l2"() -> (w2166:u16)
              n1265 = local read "LC_Reward_Tdelay_l2"() -> (w2161:u16)
              n1266 = local read "LC_Reward_OnOff_l2"() -> (w2165:bool)
              n1267 = local read "LC_Reward_Trial_l2"() -> (w2160:u16)
              n1268 = Boolean To (0,1)(Boolean=w2158) -> (0, 1=w2159:i16)
              n1269 = Boolean To (0,1)(Boolean=w2165) -> (0, 1=w2164:i16)
              n1270 = To Unsigned Word Integer(number=w2159) -> (unsigned 16bit integer=w2156:u16)
              n1271 = To Unsigned Word Integer(number=w2164) -> (unsigned 16bit integer=w2163:u16)
              n1272 = Replace Array Subset(array=w2167, new element #1=w2166, index #1=w2138, new element #2=w2163, index #2=w2139, new element #3=w2162, index #3=w2140, new element #4=w2161, index #4=w2141, new element #5=w2160, index #5=w2142, new element #6=w2157, index #6=w2133, new element #7=w2156, index #7=w2134, new element #8=w2155, index #8=w2135, new element #9=w2154, index #9=w2136, new element #10=w2153, index #10=w2137) -> (w2168:u16[])
            }
            frame "setSettings_Audio" {
              # "amp_L"
              # "amp_R"
              # "freq_L"
              # "freq_R"
              n1273 = call "myRIO_BRig_RT_dataExp_Audio_amp__L.vi"() -> ("output_Audio_amp__L"=w2193:i32)  [unwired: 11 in]
              n1274 = call "myRIO_BRig_RT_dataExp_Audio_amp__R.vi"() -> ("output_Audio_amp__R"=w2192:i32)  [unwired: 11 in]
              n1275 = call "myRIO_BRig_RT_dataExp_Audio_freq__L.vi"() -> ("output_Audio_freq__L"=w2191:i32)  [unwired: 11 in]
              n1276 = call "myRIO_BRig_RT_dataExp_Audio_freq__R.vi"() -> ("output_Audio_freq__R"=w2190:i32)  [unwired: 11 in]
              n1277 = Index Array(array=w2189, index #1=w2193, index #2=w2192, index #3=w2191, index #4=w2190) -> (element #1=w2188:u16, element #2=w2187:u16, element #3=w2180:u16, element #4=w2178:u16)
              n1278 = To Unsigned Byte Integer(number=w2180) -> (unsigned 8bit integer=w2179:u8)
              n1279 = To Unsigned Byte Integer(number=w2178) -> (unsigned 8bit integer=w2177:u8)
            }
            frame "setSettings_Laser" {
              w2219 = u32 0 ("laser2_selRew_Ndelay")
              # "tDelay"
              # "Wrong l1"
              # "Reward l1"
              n1280 = local read "Laser_Tpeak_l1"() -> (w2230:dbl)
              n1281 = local read "Laser_Tshutter_l1"() -> (w2228:dbl)
              n1282 = local read "Laser_Freq_l1"() -> (w2229:dbl)
              n1283 = local read "Laser_duration_l1"() -> (w2204:u16)
              n1284 = local read "Laser_Tpeak_l2"() -> (w2226:dbl)
              n1285 = local read "Laser_Tshutter_l2"() -> (w2224:dbl)
              n1286 = local read "Laser_Freq_l2"() -> (w2225:dbl)
              n1287 = local read "Laser_duration_l2"() -> (w2203:u16)
              n1288 = local read "CueLed_Freq"() -> (w2213:dbl)
              n1289 = local read "CueLed_Tpeak"() -> (w2214:dbl)
              n1290 = call "myRIO_BRig_RT_dataLC_Reward_Tdelay_l1.vi"() -> ("output_Reward_Tdelay_l1"=w2242:i32)  [unwired: 11 in]
              n1291 = call "myRIO_BRig_RT_dataLC_Wrong_Tdelay_l1.vi"() -> ("output_Wrong_Tdelay_l1"=w2243:i32)  [unwired: 11 in]
              n1292 = local read "FPGA_count2ms"() -> (w2215:dbl)
              n1293 = Index Array(array=w2210, index #1=w2242, index #2=w2243) -> (element #1=w2241:u16, element #2=w2240:u16)
              n1294 = To Double Precision Float(number=w2241) -> (double precision float=w2237:dbl)
              n1295 = To Double Precision Float(number=w2240) -> (double precision float=w2234:dbl)
              n1296 = To Unsigned Word Integer(number=w2215) -> (unsigned 16bit integer=w2231:u16)
              n1297 = call "myRIO_BRig_RT__calc_laser_FPGA_N.vi"("input_FPGA_ms2count"=w2215, "input_Tpeak"=w2230, "input_Freq"=w2229, "input_Tshutter"=w2228, "input_duration"=w2204) -> ("output_laser_Npeak"=w2218:u32, "output_laser_Nvalley"=w2217:u32, "output_laser_Nshutter"=w2216:u32, "output_laser_Nduration"=w2227:u32, "output_laser_Tduration"=w2208:u16)  [unwired: 6 in]
              n1298 = Multiply(x=w2215, y=w2237) -> (x*y=w2238:dbl)
              n1299 = Multiply(x=w2215, y=w2234) -> (x*y=w2235:dbl)
              n1300 = call "myRIO_BRig_RT__calc_laser_FPGA_N__CueLed.vi"("input_FPGA_ms2count"=w2215, "input_Tpeak"=w2214, "input_Freq"=w2213) -> ("output_laser_Npeak"=w2212:u32, "output_laser_Nvalley"=w2211:u32)  [unwired: 11 in]
              n1301 = call "myRIO_BRig_RT__calc_laser_FPGA_N.vi"("input_FPGA_ms2count"=w2215, "input_Tpeak"=w2226, "input_Freq"=w2225, "input_Tshutter"=w2224, "input_duration"=w2203) -> ("output_laser_Npeak"=w2223:u32, "output_laser_Nvalley"=w2222:u32, "output_laser_Nshutter"=w2221:u32, "output_laser_Nduration"=w2220:u32, "output_laser_Tduration"=w2207:u16)  [unwired: 6 in]
              n1302 = Round Toward +Infinity(x=w2238) -> (ceil(x): smallest int >= x=w2239:dbl)
              n1303 = Round Toward +Infinity(x=w2235) -> (ceil(x): smallest int >= x=w2236:dbl)
              n1304 = To Unsigned Long Integer(number=w2239) -> (unsigned 32bit integer=w2233:u32)
              n1305 = To Unsigned Long Integer(number=w2236) -> (unsigned 32bit integer=w2232:u32)
              n1306 = xnode "Read/Write Control"("FPGA VI Reference In"=w2244, "error in"=w2245, "LC_nPeak_l1"=w2218, "LC_nValley_l1"=w2217, "LC_nShutter_l1"=w2216, "LR_reward_nDelay_l1"=w2233, "LR_wrong_nDelay_l1"=w2232, "LR_reward_nTotal_l1"=w2227, "LR_wrong_nTotal_l1"=w2227, "k1__counter_per_ms"=w2231, "LC_nPeak_l2"=w2223, "LC_nValley_l2"=w2222, "LC_nShutter_l2"=w2221, "LR_reward_nDelay_l2"=w2219, "LR_wrong_nDelay_l2"=w2219, "LR_reward_nTotal_l2"=w2220, "LR_wrong_nTotal_l2"=w2220, "CueLed_nPeak"=w2212, "CueLed_nValley"=w2211) -> ("error out"=→"error out":errorcluster)  [unwired: 1 out]
              n1307 = call "myRIO_BRig_RT_dataCurrent_laser1_pulse_duration.vi"() -> ("output_laser1_pulse_duration"=w2206:i32)  [unwired: 11 in]
              n1308 = call "myRIO_BRig_RT_dataCurrent_laser2_pulse_duration.vi"() -> ("output_laser2_pulse_duration"=w2205:i32)  [unwired: 11 in]
              n1309 = Replace Array Subset(array=w2210, new element #1=w2208, index #1=w2206, new element #2=w2207, index #2=w2205) -> (w2209:u16[])
            }
            frame "initBlock" {
              n1310 = call "myRIO_Brig_RT__Case_Exp_State_initBlock.vi"("input_spout"=w2288, "input_dataExp"=w2286, "input_dataCurrent"=w2287) -> ("output_spout"=w2266:enum16{"Left", "Right"}, "output_state"=w2289:T2, "output_dataExp"=w2285:u16[], "output_dataCurrent"=w2271:u16[], "output_TpB_target"=→"TpB_target":u16)  [unwired: 3 in, 1 out]
              "cSpout" <- w2266
              n1311 = call "myRIO_BRig_RT_dataCurrent_iBlock.vi"() -> ("output_iBlock"=w2270:i32)  [unwired: 11 in]
              n1312 = Index Array(array=w2271, index=w2270) -> (element=w2264:u16)
              "iBlock" <- w2264
            }
            frame "initBlock2" {
              n1313 = local write "nRewards_cur"(u16 0 ("nRewards_cur")) -> ()
              n1314 = call "myRIO_BRig_RT__Case_Exp_State_initBlock2.vi"("input_spout"=w2297, "input_dataBlock"=w2298, "input_dataCurrent"=w2296) -> ("idxDataBlock"=w2293:i32, "output_dataBlock"=w2295:u16[][])  [unwired: 7 in]
            }
            frame "initTrial" {
              n1315 = xnode "Read/Write Control"("FPGA VI Reference In"=w2317, "error in"=w2316, "SelectionState"=FALSE) -> ("error out"=w2315:errorcluster)  [unwired: 1 out]
              n1316 = call "myRIO_Brig_RT__Case_Exp_State_initTrial__v2.vi"("input_spout"=w2318, "input_dataBlock"=w2313, "input_dataExp"=w2333, "input_dataCurrent"=w2334) -> ("output_state"=w2335:T2, "output_dataExp"=w2332:u16[], "output_dataCurrent"=w2323:u16[], "output_iTrial"=w2312:u16, "output_SolenoidReward"=→"SolenoidReward":bool)  [unwired: 3 in]
              "iTrial" <- w2312
              n1317 = local write "error out"(w2315) -> ()
            }
            frame "initTrial2" {
              # "trialUntilReward"
              n1318 = call "myRIO_BRig_RT__Case_Exp_subState_LC__initTrial__v3.vi"("input_dataCurrent"=w2348, "input_dataLC"=w2347, "input_spout"=w2349, "input_dataTrial"=w2351) -> ("output_dataTrial"=w2350:u16[][], "output_LR_Wrong_Laser_l2"=w2339:bool, "output_LR_Reward_Laser_l2"=w2340:bool, "output_LR_Reward_Event_l1"=w2346:bool, "output_LR_Wrong_Event_l1"=w2345:bool, "output_LR_Reward_Laser_l1"=w2344:bool, "output_LR_Wrong_Laser_l1"=w2343:bool, "output_LR_Reward_Event_l2"=w2342:bool, "output_LR_Wrong_Event_l2"=w2341:bool)  [unwired: 7 in]
              n1319 = call "myRIO_BRig_RT_dataExp_ItrialUntilReward.vi"() -> ("output_I_trialUntilReward"=w2355:i32)  [unwired: 11 in]
              n1320 = Index Array(array=w2356, index=w2355) -> (element=w2354:u16)
              n1321 = Equal?(x=w2349, y=enum16{"Left", "Right"}."Right") -> (x = y?=w2353:bool)
              n1322 = Not Equal To 0?(x=w2354) -> (x != 0?=w2352:bool)
              n1323 = xnode "Read/Write Control"("FPGA VI Reference In"=w2370, "error in"=w2369, "Left(F)_or_Right(T)"=w2353, "ignoreWrong"=w2352, "LR_reward_Event_l1"=w2346, "LR_wrong_Event_l1"=w2345, "LR_reward_Laser_l1"=w2344, "LR_wrong_Laser_l1"=w2343, "LR_reward_Event_l2"=w2342, "LR_wrong_Event_l2"=w2341, "LR_reward_Laser_l2"=w2340, "LR_wrong_laser_l2"=w2339) -> ("error out"=→"error_initTrial":errorcluster)  [unwired: 1 out]
            }
            frame "initTrial3" {
              # "Cue1_CueType"
              n1324 = call "myRIO_BRig_RT_dataExp_CueLed.vi"() -> ("output_CueLed"=w2377:i32)  [unwired: 11 in]
              n1325 = call "myRIO_BRig_RT_arrTrig_init.vi"() -> ("output_arrTrig"=w2381:bool[])  [unwired: 11 in]
              n1326 = Index Array(array=w2378, index=w2377) -> (element=w2376:u16)
              n1327 = call "myRIO_BRig_RT_arrTrig_Cue1_CueType_AudioLed.vi"() -> ("output_arrTrig_Cue1_CueType_AudioLed"=w2379:i32)  [unwired: 11 in]
              n1328 = Not Equal To 0?(x=w2376) -> (x != 0?=w2375:bool)
              n1329 = call "myRIO_BRig_RT__Case_Exp_State_initTrial_dataTrial.vi"("input_spout"=w2397, "input_dataCurrent"=w2383, "input_dataExp"=w2378, "input_dataTrial"=w2399) -> ("output_laserPower_l2"=w2385:u16, "output_dataCurrent"=w2382:u16[], "output_dataTrial"=w2398:u16[][], "output_laserPower_l1"=w2394:u16)  [unwired: 4 in]
              n1330 = To Double Precision Float(number=w2394) -> (double precision float=w2396:dbl)
              n1331 = To Double Precision Float(number=w2385) -> (double precision float=w2388:dbl)
              n1332 = Replace Array Subset(array=w2381, new element=w2375, index=w2379) -> (w2380:bool[])
              n1333 = Divide(x=w2396, y=100.0 ("x")) -> (x/y=w2390:dbl)
              "power_l1" <- w2390
              n1334 = Divide(x=w2388, y=100.0 ("x")) -> (x/y=w2386:dbl)
              "power_l2" <- w2386
              n1335 = call "myRIO__convert__Voltage_to_FPGAvalue.vi"("input_voltage"=w2390) -> ("output_PortC"=w2389:i16)  [unwired: 9 in, 1 out]
              n1336 = call "myRIO__convert__Voltage_to_FPGAvalue.vi"("input_voltage"=w2386) -> ("output_PortC"=w2384:i16)  [unwired: 9 in, 1 out]
              n1337 = xnode "Read/Write Control"("FPGA VI Reference In"=w2393, "error in"=w2392, "AnaOut_0"=w2389, "AnaOut_1"=w2384) -> ("error out"=→"error out 4":errorcluster)  [unwired: 1 out]
            }
            frame "initTrial4" {
              n1338 = call "myRIO_BRig_RT_dataCurrent_idxDataTrial.vi"() -> ("output_idxDataTrial"=w2423:i32)  [unwired: 11 in]
              n1339 = call "myRIO_BRig_RT_dataTrial_activeRecording.vi"() -> ("output_activeRecording"=w2420:i32)  [unwired: 11 in]
              n1340 = Index Array(array=w2425, index=w2423) -> (element=w2422:u16)
              n1341 = Boolean To (0,1)(Boolean="Recording") -> (0, 1=w2419:i16)
              n1342 = To Long Integer(number=w2422) -> (32bit integer=w2421:i32)
              n1343 = To Unsigned Word Integer(number=w2419) -> (unsigned 16bit integer=w2418:u16)
              n1344 = Replace Array Subset(array=w2424, new element=w2418, index (row)=w2421, index (col)=w2420) -> (w2417:u16[][])
            }
            frame "initTrial_LC_ENL1" {
              n1345 = call "myRIO_BRig_RT__Case_Exp_State_initTrial_LC_ENL1__v3.vi"("input_dataTrial"=w2448, "input_spout"=w2451, "input_arrTrig"=w2445, "input_dataBlock"=w2446, "input_dataLC"=w2452, "input_dataCurrent"=w2450) -> ("output_arrTrig"=w2444:bool[], "output_dataTrial"=w2447:u16[][], "output_dataCurrent"=w2449:u16[])  [unwired: 3 in]
            }
            frame "initTrial_LC_Cue1" {
              n1346 = call "myRIO_BRig_RT__Case_Exp_State_initTrial_LC_Cue1__v3.vi"("input_dataTrial"=w2470, "input_spout"=w2473, "input_arrTrig"=w2467, "input_dataBlock"=w2468, "input_dataLC"=w2474, "input_dataCurrent"=w2472) -> ("output_arrTrig"=w2466:bool[], "output_dataTrial"=w2469:u16[][], "output_dataCurrent"=w2471:u16[])  [unwired: 3 in]
            }
            frame "initTrial_LC_Cue1_2" {
              w2502 = TRUE ("Recording")
              n1347 = local read "Cue1Param_AudioLed_Probability_Switch"() -> (w2495:u16)
              n1348 = local read "Cue1Param_AudioLed_Count_Switch"() -> (w2494:u16)
              n1349 = local read "Cue1Param_AudioLed_Probability_NS"() -> (w2492:u16)
              n1350 = local read "Cue1Param_AudioLed_Count_NS"() -> (w2491:u16)
              n1351 = local read "Cue1Param_CueType_Switch"() -> (w2496:u16)
              n1352 = local read "Cue1Param_CueType_NS"() -> (w2493:u16)
              n1353 = call "myRIO_BRig_RT__Case_Exp_State_initTrial_LC_Cue1_2.vi"("input_CueType_Switch"=w2496, "input_Probability_Switch"=w2495, "input_Count_Switch"=w2494, "input_CueType_NS"=w2493, "input_Probability_NS"=w2492, "input_Count_NS"=w2491, "input_spout"=w2490, "input_dataBlock"=w2489, "input_dataCurrent"=w2500, "input_arrTrig"=w2498) -> ("output_dataCurrent"=w2499:u16[], "output_arrTrig"=w2497:bool[])  [unwired: 8 in]
            }
            frame "initTrial_LC_Sel" {
              n1354 = call "myRIO_BRig_RT__Case_Exp_State_initTrial_LC_Sel__v3.vi"("input_dataTrial"=w2524, "input_spout"=w2527, "input_arrTrig"=w2519, "input_dataBlock"=w2522, "input_dataLC"=w2528, "input_dataCurrent"=w2526) -> ("output_arrTrig"=w2518:bool[], "output_dataTrial"=w2523:u16[][], "output_dataCurrent"=w2525:u16[])  [unwired: 3 in]
              n1355 = local read "Recording"() -> (w2521:bool)
            }
            frame "ENL1_pre" {
              n1356 = call "myRIO_BRig_RT__Case_Exp_State_Enl1Pre__v3.vi"("input_I_lick"=w2546, "input_arrTrig"=w2543, "input_dataCurrent"=w2547) -> ("output_dataCurrent"=w2544:u16[], "output_state"=w2545:T2)  [unwired: 3 in, 4 out]
            }
            frame "ENL1" {
              n1357 = call "myRIO_BRig_RT__Case_Exp_State_ENL1__v3.vi"("I_lick"=w2570, "input_arrTrig"=w2568, "input_state"=w2574, "input_dataCurrent"=w2573) -> ("output_l1_laserOn"=w2566:bool, "output_l1_laserEvent"=w2567:bool, "output_state"=w2571:T2, "output_dataCurrent"=w2572:u16[], "output_l2_laserEvent"=w2565:bool, "output_l2_laserOn"=w2564:bool)  [unwired: 2 in]
            }
            frame "ENL1Penalty_pre" {
              # "Tcycle"
              # "counter"
              n1358 = call "myRIO_BRig_RT_dataCurrent_Tcycle_generic.vi"() -> ("output_Tcycle_generic"=w2609:i32)  [unwired: 11 in]
              n1359 = call "myRIO_BRig_RT_dataCurrent_count_generic.vi"() -> ("output_count_generic"=w2611:i32)  [unwired: 11 in]
              n1360 = call "myRIO_BRig_RT_dataExp_ENL_penalty.vi"() -> ("output_ENL_penalty"=w2604:i32)  [unwired: 11 in]
              n1361 = Index Array(array=w2605, index=w2604) -> (element=w2608:u16)
              n1362 = Replace Array Subset(array=w2606, new element #1=u16 0 ("new element/subarray"), index #1=w2611, new element #2=w2608, index #2=w2609) -> (w2607:u16[])
            }
            frame "ENL1Penalty" {
              n1363 = call "myRIO_BRig_RT__Case_Exp_State_ENL1Penalty.vi"("input_state"=w2629, "input_dataCurrent"=w2633) -> ("output_state"=w2630:T2, "output_dataCurrent"=w2632:u16[])  [unwired: 8 in]
            }
            frame "ENL2_pre" {
            }
            frame "ENL2" {
            }
            frame "ENL2Penalty_pre" {
            }
            frame "ENL2Penalty" {
            }
            frame "Cue1_pre" {
              n1364 = call "myRIO_BRig_RT__Case_Exp_State_Cue1Pre__v3.vi"("input_dataCurrent"=w2721, "input_dataExp"=w2717, "input_arrTrig"=w2714, "input_spout"=w2718) -> ("output_audioR"=w2715:bool, "output_audioL"=w2716:bool, "output_state"=w2719:T2, "output_dataCurrent"=w2720:u16[])  [unwired: 7 in, 5 out]
            }
            frame "Cue1" {
              n1365 = call "myRIO_BRig_RT__Case_Exp_State_Cue1__v3.vi"("I_lick"=w2744, "input_arrTrig"=w2742, "input_state"=w2746, "input_dataCurrent"=w2764) -> ("output_l1_laserOn"=w2740:bool, "output_l1_laserEvent"=w2741:bool, "output_state"=w2745:T2, "output_dataCurrent"=w2763:u16[], "output_l2_laserEvent"=w2739:bool, "output_CueLed_Event"=w2737:bool, "output_l2_laserOn"=w2738:bool)  [unwired: 1 in]
              n1366 = Equal?(x=myRIO_BRig_RT__Case_Exp_stateList."Selection_pre", y=w2745) -> (x = y?=w2749:bool)
              n1367 = xnode "Read/Write Control"("FPGA VI Reference In"=w2748, "error in"=w2747, "SelectionState"=w2749) -> ()  [unwired: 2 out]
            }
            frame "Cue1Penalty_pre" {
              # "Tcycle"
              # "counter"
              n1368 = call "myRIO_BRig_RT_dataCurrent_Tcycle_generic.vi"() -> ("output_Tcycle_generic"=w2796:i32)  [unwired: 11 in]
              n1369 = call "myRIO_BRig_RT_dataCurrent_count_generic.vi"() -> ("output_count_generic"=w2798:i32)  [unwired: 11 in]
              n1370 = call "myRIO_BRig_RT_dataExp_CueLed.vi"() -> ("output_CueLed"=w2776:i32)  [unwired: 11 in]
              n1371 = call "myRIO_BRig_RT_dataExp_Tcycle_Cue1Penalty_Audio.vi"() -> ("output_Tcycle_Cue1Penalty_Audio"=w2777:i32)  [unwired: 11 in]
              n1372 = call "myRIO_BRig_RT_dataExp_Tcycle_Cue1Penalty_LED.vi"() -> ("output_Tcycle_Cue1Penalty_LED"=w2775:i32)  [unwired: 11 in]
              n1373 = Index Array(array=w2792, index #1=w2776, index #2=w2777, index #3=w2775) -> (element #1=w2774:u16, element #2=w2772:u16, element #3=w2771:u16)
              n1374 = Equal To 0?(x=w2774) -> (x = 0?=w2773:bool)
              n1375 = Select(t=w2772, s=w2773, f=w2771) -> (s? t:f=w2770:u16)
              n1376 = Replace Array Subset(array=w2794, new element #1=u16 0 ("new element/subarray"), index #1=w2798, new element #2=w2770, index #2=w2796) -> (w2793:u16[])
            }
            frame "Cue1Penalty" {
              n1377 = call "myRIO_BRig_RT__Case_Exp_State_Cue1Penalty.vi"("input_state"=w2819, "input_dataCurrent"=w2820) -> ("output_state"=w2817:T2, "output_dataCurrent"=w2818:u16[])  [unwired: 8 in]
            }
            frame "Cue2_pre" {
            }
            frame "Cue2" {
            }
            frame "Cue2Penalty_pre" {
            }
            frame "Cue2Penalty" {
            }
            frame "Selection_pre" {
              n1378 = xnode "Read/Write Control"("FPGA VI Reference In"=w2912, "error in"=w2913) -> ("error out"=→"error_Selection_pre":errorcluster, "SelectReward"=w2906:bool, "SelectWrong"=w2907:bool)  [unwired: 1 out]
              n1379 = call "myRIO_BRig_RT__Case_Exp_State_SelectPre__v3.vi"("input_dataCurrent"=w2910, "input_SelectWrong"=w2907, "input_SelectReward"=w2906, "input_dataExp"=w2900, "input_arrTrig"=w2905) -> ("output_state"=w2908:T2, "output_dataCurrent"=w2909:u16[], "output_l1_laserEvent"=w2904:bool, "output_l1_laserOn"=w2903:bool, "output_l2_laserOn"=w2901:bool, "output_l2_laserEvent"=w2902:bool)  [unwired: 5 in]
            }
            frame "Selection" {
              n1380 = xnode "Read/Write Control"("FPGA VI Reference In"=w2943, "error in"=w2942) -> ("error out"=→"error_Selection":errorcluster, "SelectReward"=w2936:bool, "SelectWrong"=w2935:bool)  [unwired: 1 out]
              n1381 = call "myRIO_BRig_RT__Case_Exp_State_Selection__v2.vi"("input_dataCurrent"=w2940, "input_state"=w2938, "input_FPGA_SelectReward"=w2936, "input_FPGA_SelectWrong"=w2935, "input_arrTrig"=w2934) -> ("output_state"=w2937:T2, "output_dataCurrent"=w2939:u16[], "output_LC_Event_l1"=w2933:bool, "output_LC_Laser_l2"=w2930:bool, "output_LC_Event_l2"=w2931:bool, "output_LC_Laser_l1"=w2932:bool)  [unwired: 5 in]
            }
            frame "SelectReward_pre" {
              # "iState"
              # "Tcycle\nReward"
              # "nRewTrials"
              # "Tcycle\nGeneric"
              # "counter"
              n1382 = call "myRIO_BRig_RT_dataCurrent_nRewTrials.vi"() -> ("output_nRewTrials"=w2975:i32)  [unwired: 11 in]
              n1383 = Equal?(x=w2984, y=enum16{"Left", "Right"}."Left") -> (x = y?=w2985:bool)
              n1384 = Index Array(array=w2976, index=w2975) -> (element=w2974:u16)
              n1385 = call "myRIO_BRig_RT_dataExp_Tcycle_Reward__L.vi"() -> ("output_Tcycle_Reward__L"=w2988:i32)  [unwired: 11 in]
              n1386 = call "myRIO_BRig_RT_dataExp_Tcycle_Reward__R.vi"() -> ("output_Tcycle_Reward__R"=w2989:i32)  [unwired: 11 in]
              n1387 = Increment(x=w2974) -> (x+1=w2973:u16)
              n1388 = Select(t=w2988, s=w2985, f=w2989) -> (s? t:f=w2987:i32)
              n1389 = call "myRIO_BRig_RT__Case_Exp_subState_LC__Reward.vi"("input_spout"=w2984, "input_dataCurrent"=w2976, "input_dataLC"=w2983) -> ()  [unwired: 6 in, 2 out]
              n1390 = call "myRIO_BRig_RT_dataCurrent_count_generic.vi"() -> ("output_count_generic"=w2978:i32)  [unwired: 11 in]
              n1391 = call "myRIO_BRig_RT_dataCurrent_Tcycle_generic.vi"() -> ("output_Tcycle_generic"=w2979:i32)  [unwired: 11 in]
              n1392 = Index Array(array=w2990, index=w2987) -> (element=w2980:u16)
              n1393 = call "myRIO_BRig_RT_dataCurrent_iState.vi"() -> ("output_iState"=w2968:i32)  [unwired: 11 in]
              n1394 = Replace Array Subset(array=w2976, new element #1=w2973, index #1=w2975, new element #2=u16 0 ("new element/subarray"), index #2=w2978, new element #3=w2980, index #3=w2979, new element #4=u16 1 ("new element/subarray"), index #4=w2968) -> (w2991:u16[])
            }
            frame "SelectReward" {
              n1395 = call "myRIO_BRig_RT__Case_Exp_State_Reward.vi"("input_dataCurrent"=w3012, "input_state"=w3009, "input_spout"=w3007) -> ("output_dataCurrent"=w3011:u16[], "output_state"=w3010:T2, "output__L"=w3005:bool, "output__R"=w3006:bool)  [unwired: 9 in]
            }
            frame "SelectRewardPost_pre" {
              # "nRewards"
              # "nRewTrials"
              # "Tcycle"
              # "counter"
              n1396 = call "myRIO_BRig_RT_dataBlock_nRewards__L.vi"() -> ("output_nRewards__L"=w3028:i32)  [unwired: 11 in]
              n1397 = call "myRIO_BRig_RT_dataBlock_nRewards__R.vi"() -> ("output_nRewards__R"=w3027:i32)  [unwired: 11 in]
              n1398 = call "myRIO_BRig_RT_dataCurrent_Tcycle_generic.vi"() -> ("output_Tcycle_generic"=w3047:i32)  [unwired: 11 in]
              n1399 = call "myRIO_BRig_RT_dataCurrent_count_generic.vi"() -> ("output_count_generic"=w3049:i32)  [unwired: 11 in]
              n1400 = case shown="\"Left\", Default" w3021 {
                tunnel: w3033 -> [w3054 w3058]
                tunnel: [w3053 w3058] -> w3032
                tunnel: [w3055 w3056] -> w3031
                tunnel: w3030 -> [w3055 w3057]
                frame "Left", Default {
                  n1401 = Increment(x=w3054) -> (x+1=w3053:u16)
                }
                frame "Right" {
                  n1402 = Increment(x=w3057) -> (x+1=w3056:u16)
                }
              }
              "nRewards_Left" <- w3032
              "nRewards_Right" <- w3031
              n1403 = Equal?(x=w3021, y=enum16{"Left", "Right"}."Left") -> (x = y?=w3020:bool)
              n1404 = Select(t=w3028, s=w3020, f=w3027) -> (s? t:f=w3026:i32)
              n1405 = call "myRIO_BRig_RT_dataExp_Tcycle_RewardPost.vi"() -> ("output_Tcycle_RewardPost"=w3043:i32)  [unwired: 11 in]
              n1406 = call "myRIO_BRig_RT_dataCurrent_nRewTrials.vi"() -> ("output_nRewTrials"=w3029:i32)  [unwired: 11 in]
              n1407 = Index Array(array=w3044, index=w3043) -> (element=w3046:u16)
              n1408 = Index Array(array=w3023, index=w3029) -> (element=w3018:u16)
              n1409 = Replace Array Subset(array=w3023, new element #1=u16 0 ("new element/subarray"), index #1=w3049, new element #2=w3046, index #2=w3047) -> (w3045:u16[])
              n1410 = Replace Array Subset(array=w3025, new element=w3018, index (row)=w3019, index (col)=w3026) -> (w3024:u16[][])
              n1411 = local write "nRewards_cur"(w3018) -> ()
            }
            frame "SelectRewardPost" {
              n1412 = call "myRIO_BRig_RT__Case_Exp_State_RewardPost.vi"("input_state"=w3073, "input_dataCurrent"=w3076) -> ("output_state"=w3074:T2, "output_dataCurrent"=w3075:u16[])  [unwired: 8 in]
            }
            frame "SelectWrong_pre" {
              # "iState"
              # "Tcycle"
              # "counter"
              n1413 = call "myRIO_BRig_RT_dataCurrent_Tcycle_generic.vi"() -> ("output_Tcycle_generic"=w3101:i32)  [unwired: 11 in]
              n1414 = call "myRIO_BRig_RT_dataCurrent_count_generic.vi"() -> ("output_count_generic"=w3103:i32)  [unwired: 11 in]
              n1415 = call "myRIO_BRig_RT_dataExp_Tcycle_Wrong.vi"() -> ("output_Tcycle_Wrong"=w3099:i32)  [unwired: 11 in]
              n1416 = call "myRIO_BRig_RT__Case_Exp_subState_LC__Wrong.vi"("input_spout"=w3095, "input_dataCurrent"=w3096, "input_dataLC"=w3093) -> ()  [unwired: 6 in, 2 out]
              n1417 = Index Array(array=w3097, index=w3099) -> (element=w3100:u16)
              n1418 = call "myRIO_BRig_RT_dataCurrent_iState.vi"() -> ("output_iState"=w3087:i32)  [unwired: 11 in]
              n1419 = Replace Array Subset(array=w3096, new element #1=u16 0 ("new element/subarray"), index #1=w3103, new element #2=w3100, index #2=w3101, new element #3=u16 2 ("new element/subarray"), index #3=w3087) -> (w3098:u16[])
            }
            frame "SelectWrong" {
              n1420 = call "myRIO_BRig_RT__Case_Exp_State_Wrong.vi"("input_state"=w3117, "input_dataCurrent"=w3126) -> ("output_state"=w3114:T2, "output_dataCurrent"=w3125:u16[])  [unwired: 8 in]
              n1421 = Not Equal?(x=w3117, y=w3114) -> (x != y?=w3116:bool)
              n1422 = Select(t=myRIO_BRig_RT__Case_Exp_stateList."SelectWrong_post" ("Enum"), s=w3116, f=w3114) -> (s? t:f=w3113:T2)
            }
            frame "SelectWrong_post" {
            }
            frame "SelectTimeout_pre" {
              # "iState"
              # "Tcycle"
              # "counter"
              n1423 = xnode "Read/Write Control"("FPGA VI Reference In"=w3153, "error in"=w3152, "SelectionState"=FALSE) -> ("error out"=→"error out 3":errorcluster)  [unwired: 1 out]
              n1424 = call "myRIO_BRig_RT_dataCurrent_Tcycle_generic.vi"() -> ("output_Tcycle_generic"=w3175:i32)  [unwired: 11 in]
              n1425 = call "myRIO_BRig_RT_dataCurrent_count_generic.vi"() -> ("output_count_generic"=w3173:i32)  [unwired: 11 in]
              n1426 = call "myRIO_BRig_RT_dataExp_Tcycle_Timeout.vi"() -> ("output_Tcycle_Timeout"=w3177:i32)  [unwired: 11 in]
              n1427 = call "myRIO_BRig_RT__Case_Exp_subState_LC__Timeout.vi"("input_spout"=w3168, "input_dataCurrent"=w3169, "input_dataLC"=w3167) -> ()  [unwired: 6 in, 2 out]
              n1428 = Index Array(array=w3171, index=w3177) -> (element=w3176:u16)
              n1429 = call "myRIO_BRig_RT_dataCurrent_iState.vi"() -> ("output_iState"=w3161:i32)  [unwired: 11 in]
              n1430 = Replace Array Subset(array=w3169, new element #1=u16 0 ("new element/subarray"), index #1=w3173, new element #2=w3176, index #2=w3175, new element #3=u16 3 ("new element/subarray"), index #3=w3161) -> (w3172:u16[])
            }
            frame "SelectTimeout" {
              n1431 = call "myRIO_BRig_RT__Case_Exp_State_Timeout.vi"("input_dataLC"=w3196, "input_state"=w3187, "input_dataCurrent"=w3201) -> ("output_state"=w3188:T2, "output_dataCurrent"=w3200:u16[])  [unwired: 6 in, 1 out]
              n1432 = Not Equal?(x=w3187, y=w3188) -> (x != y?=w3191:bool)
              n1433 = Select(t=myRIO_BRig_RT__Case_Exp_stateList."SelectTimeout_post" ("Enum"), s=w3191, f=w3188) -> (s? t:f=w3189:T2)
            }
            frame "SelectTimeout_post" {
            }
            frame "endTrial1" {
              # "Update dataBlock"
              n1434 = call "myRIO_BRig_RT__Case_Exp_State_endTrial1.vi"("input_spout"=w3234, "input_dataBlock"=w3233, "input_dataCurrent"=w3231) -> ("output_dataBlock"=w3232:u16[][], "output_dataCurrent"=w3230:u16[])  [unwired: 7 in]
            }
            frame "endTrial2" {
              # "update dataTrial"
              n1435 = call "myRIO_BRig_RT__Case_Exp_State_endTrial2.vi"("input_dataExp"=w3245, "input_spout"=w3254, "input_dataTrial"=w3258, "input_dataCurrent"=w3256) -> ("output_dataTrial"=w3257:u16[][], "output_dataCurrent"=w3255:u16[])  [unwired: 6 in]
            }
            frame "endTrial3" {
              # "nRewTrials"
              # "iTrial"
              # "I_blockUntilReward"
              # "TPB"
              # "end block?"
              n1436 = local read "STOP_endTrial"() -> (w3283:bool)
              n1437 = local read "STOP_abort"() -> (w3282:bool)
              n1438 = xnode "Read/Write Control"("FPGA VI Reference In"=w3273, "error in"=w3272, "SelectionState"=FALSE) -> ("error out"=→"error out 2":errorcluster)  [unwired: 1 out]
              n1439 = local read "START"() -> (w3280:bool)
              n1440 = call "myRIO_BRig_RT_dataExp_IblockUntilReward.vi"() -> ("output_I_blockUntilReward"=w3290:i32)  [unwired: 11 in]
              n1441 = Index Array(array=w3276, index=w3290) -> (element=w3274:u16)
              n1442 = Not(x=w3280) -> (.not. x?=w3281:bool)
              n1443 = Not Equal To 0?(x=w3274) -> (x != 0?=w3288:bool)
              n1444 = Compound Arithmetic op=OR(w3283, w3281, w3282) -> (w3268:bool)
              n1445 = call "myRIO_BRig_RT_dataCurrent_nRewTrials.vi"() -> ("output_nRewTrials"=w3286:i32)  [unwired: 11 in]
              n1446 = call "myRIO_BRig_RT_dataCurrent_iTrial.vi"() -> ("output_iTrial"=w3287:i32)  [unwired: 11 in]
              n1447 = Select(t=w3286, s=w3288, f=w3287) -> (s? t:f=w3285:i32)
              n1448 = call "myRIO_BRig_RT_dataCurrent_TpB.vi"() -> ("output_TpB"=w3289:i32)  [unwired: 11 in]
              n1449 = Index Array(array=w3277, index #1=w3289, index #2=w3285) -> (element #1=w3278:u16, element #2=w3279:u16)
              n1450 = Less Or Equal?(x=w3278, y=w3279) -> (x <= y?=w3269:bool)
              n1451 = Or(x=w3268, y=w3269) -> (x .or. y?=w3266:bool)
              n1452 = Select(t=myRIO_BRig_RT__Case_Exp_stateList."saveData_dataBlock" ("Enum"), s=w3266, f=myRIO_BRig_RT__Case_Exp_stateList."dummyState" ("Enum")) -> (s? t:f=w3275:T2)
            }
            frame "endBlock" {
              # "R"
              # "L"
              # "idxDataBlock"
              n1453 = Equal?(x=w3314, y=enum16{"Left", "Right"}."Left") -> (x = y?=w3313:bool)
              n1454 = call "myRIO_BRig_RT_dataCurrent_idxDataBlockL.vi"() -> ("output_idxDataBlock__L"=w3317:i32)  [unwired: 11 in]
              n1455 = call "myRIO_BRig_RT_dataCurrent_idxDataBlockR.vi"() -> ("output_idxDataBlock__R"=w3316:i32)  [unwired: 11 in]
              n1456 = Increment(x=w3308) -> (x+1=w3307:i32)
              n1457 = local read "START"() -> (w3337:bool)
              n1458 = local read "STOP_endBlock"() -> (w3332:bool)
              n1459 = local read "STOP_endTrial"() -> (w3335:bool)
              n1460 = local read "STOP_abort"() -> (w3334:bool)
              n1461 = Select(t=w3317, s=w3313, f=w3316) -> (s? t:f=w3311:i32)
              n1462 = To Unsigned Word Integer(number=w3307) -> (unsigned 16bit integer=w3309:u16)
              n1463 = Not(x=w3337) -> (.not. x?=w3336:bool)
              n1464 = Replace Array Subset(array=w3312, new element=w3309, index=w3311) -> (w3310:u16[])
              n1465 = Compound Arithmetic op=OR(w3336, w3332, w3335, w3334) -> (w3333:bool)
              n1466 = Select(t=myRIO_BRig_RT__Case_Exp_stateList."endExp" ("Enum"), s=w3333, f=myRIO_BRig_RT__Case_Exp_stateList."dummyState_endBlock" ("Enum")) -> (s? t:f=w3341:T2)
            }
            frame "endExp" {
            }
            frame "commConnect" {
              n1467 = call "myRIO_BRig_RT_comm_webdav_connect.vi"("input_password"="Host Password", "input_username"="Host UserName") -> ("output_Iconnected"=w3362:bool, "output_hSession"=w3380:T6)  [unwired: 7 in, 1 out]
              "Connected To Host?" <- w3362
              n1468 = case shown="False" w3362 {
                frame False {
                  n1469 = One Button Dialog(message="Connection Failed!\nData not being saved!") -> ()  [unwired: 1 in, 1 out]
                }
                frame True {
                }
              }
            }
            frame "commUpload_pre" {
              n1470 = Select(t=myRIO_BRig_RT__Case_Exp_stateList."commUpload_dataBlock" ("Enum"), s=w3387, f=myRIO_BRig_RT__Case_Exp_stateList."endBlock") -> (s? t:f=w3385:T2)
            }
            frame "commUpload_dataBlock" {
              n1471 = call "myRIO_BRig_RT_comm_webdav_uploadFile__data.vi"("input_fileName_prefix"=w3408, "input_fileName"="dataBlock" ("input_filename"), "input_hSession"=w3410) -> ()  [unwired: 8 in, 1 out]
            }
            frame "commUpload_dataCurrent" {
              n1472 = call "myRIO_BRig_RT_comm_webdav_uploadFile__data.vi"("input_fileName_prefix"=w3429, "input_fileName"="dataCurrent" ("input_filename"), "input_hSession"=w3431) -> ()  [unwired: 8 in, 1 out]
            }
            frame "commUpload_dataExp" {
              n1473 = call "myRIO_BRig_RT_comm_webdav_uploadFile__data.vi"("input_fileName_prefix"=w3450, "input_fileName"="dataExp" ("input_filename"), "input_hSession"=w3452) -> ()  [unwired: 8 in, 1 out]
            }
            frame "commUpload_dataLC" {
              n1474 = call "myRIO_BRig_RT_comm_webdav_uploadFile__data.vi"("input_fileName_prefix"=w3471, "input_fileName"="dataLC" ("input_filename"), "input_hSession"=w3473) -> ()  [unwired: 8 in, 1 out]
            }
            frame "commUpload_dataTrial" {
              n1475 = call "myRIO_BRig_RT_comm_webdav_uploadFile__data.vi"("input_fileName_prefix"=w3495, "input_fileName"="dataTrial" ("input_filename"), "input_hSession"=w3497) -> ()  [unwired: 8 in, 1 out]
            }
            frame "saveData_dataBlock" {
              # "idxDataBlockR"
              # "idxDataBlockL"
              n1476 = call "myRIO_BRig_RT_dataCurrent_idxDataBlockL.vi"() -> ("output_idxDataBlock__L"=w3521:i32)  [unwired: 11 in]
              n1477 = call "myRIO_BRig_RT_dataCurrent_idxDataBlockR.vi"() -> ("output_idxDataBlock__R"=w3522:i32)  [unwired: 11 in]
              n1478 = Index Array(array=w3523, index #1=w3521, index #2=w3522) -> (element #1=w3520:u16, element #2=w3519:u16)
              n1479 = Greater?(x=w3520, y=w3519) -> (0:w3518:bool)
              n1480 = Select(t=w3520, s=w3518, f=w3519) -> (s? t:f=w3516:u16)
              n1481 = Increment(x=w3516) -> (x+1=w3515:u16)
              n1482 = To Long Integer(number=w3515) -> (32bit integer=w3514:i32)
              n1483 = Array Subset(array=w3517, length (row)=w3514) -> (w3513:u16[][])  [unwired: 3 in]
              n1484 = call "myRIO_BRig_RT_comm_webdav_saveArrayToFile__2D_u16.vi"("Array"=w3513, "input_filename"="dataBlock") -> ()  [unwired: 10 in]
            }
            frame "saveData_dataCurrent" {
              n1485 = call "myRIO_BRig_RT_comm_webdav_saveArrayToFile__1D_u16.vi"("Array"=w3542, "input_filename"="dataCurrent") -> ()  [unwired: 10 in]
            }
            frame "saveData_dataExp" {
              # "runTime"
              n1486 = Get Date/Time In Seconds() -> (seconds since 1Jan1904=w3570:timestamp)
              n1487 = To Double Precision Float(number=w3570) -> (double precision float=w3569:dbl)
              n1488 = call "myRIO_BRig_RT_dataExp_runTime_seconds.vi"() -> ("output_RunTime_minutes"=w3568:i32)  [unwired: 11 in]
              n1489 = Subtract(x=w3569, y=w3567) -> (x-y=w3564:dbl)
              n1490 = To Unsigned Word Integer(number=w3564) -> (unsigned 16bit integer=w3563:u16)
              n1491 = Replace Array Subset(array=w3562, new element=w3563, index=w3568) -> (w3565:u16[])
              n1492 = call "myRIO_BRig_RT_comm_webdav_saveArrayToFile__1D_u16.vi"("Array"=w3565, "input_filename"="dataExp") -> ()  [unwired: 10 in]
            }
            frame "saveData_dataLC" {
              n1493 = call "myRIO_BRig_RT_comm_webdav_saveArrayToFile__1D_u16.vi"("Array"=w3589, "input_filename"="dataLC") -> ()  [unwired: 10 in]
            }
            frame "saveData_dataTrial" {
              # "idxTrial"
              n1494 = call "myRIO_BRig_RT_dataCurrent_idxDataTrial.vi"() -> ("output_idxDataTrial"=w3613:i32)  [unwired: 11 in]
              n1495 = Index Array(array=w3614, index=w3613) -> (element=w3606:u16)
              n1496 = Increment(x=w3606) -> ()  [unwired: 1 out]
              n1497 = To Long Integer(number=w3606) -> (32bit integer=w3610:i32)
              n1498 = Array Subset(array=w3611, length (row)=w3610) -> (w3612:u16[][])  [unwired: 3 in]
              n1499 = call "myRIO_BRig_RT_comm_webdav_saveArrayToFile__2D_u16.vi"("Array"=w3612, "input_filename"="dataTrial") -> ()  [unwired: 10 in]
            }
            frame "dummyState" {
              n1500 = call "myRIO_BRig_RT_dataCurrent_iTrial.vi"() -> ("output_iTrial"=w3636:i32)  [unwired: 11 in]
              n1501 = Index Array(array=w3637, index=w3636) -> (element=w3635:u16)
              n1502 = Equal?(x=w3635, y=u16 1) -> (x = y?=w3633:bool)
              n1503 = Equal To 0?(x=w3644) -> (x = 0?=w3645:bool)
              n1504 = Select(t=u16 13, s=w3633, f=u16 15) -> (s? t:f=w3630:u16)
              n1505 = Select(t=w3630, s=w3645, f=w3644) -> (s? t:f=w3643:u16)
              n1506 = Decrement(x=w3643) -> (x-1=w3642:u16)
              n1507 = Equal To 0?(x=w3642) -> (x = 0?=w3641:bool)
              n1508 = Select(t=myRIO_BRig_RT__Case_Exp_stateList."initTrial" ("Enum"), s=w3641, f=w3639) -> (s? t:f=w3638:T2)
            }
            frame "dummyState_endBlock" {
              n1509 = call "myRIO_BRig_RT_dataCurrent_iTrial.vi"() -> ("output_iTrial"=w3669:i32)  [unwired: 11 in]
              n1510 = Index Array(array=w3670, index=w3669) -> (element=w3668:u16)
              n1511 = Equal?(x=w3668, y=u16 1) -> (x = y?=w3666:bool)
              n1512 = Equal To 0?(x=w3677) -> (x = 0?=w3678:bool)
              n1513 = Select(t=u16 1, s=w3666, f=u16 3) -> (s? t:f=w3663:u16)
              n1514 = Select(t=w3663, s=w3678, f=w3677) -> (s? t:f=w3676:u16)
              n1515 = Decrement(x=w3676) -> (x-1=w3675:u16)
              n1516 = Equal To 0?(x=w3675) -> (x = 0?=w3674:bool)
              n1517 = Select(t=myRIO_BRig_RT__Case_Exp_stateList."initBlock" ("Enum"), s=w3674, f=w3672) -> (s? t:f=w3671:T2)
            }
          }
          n1518 = local read "MTrig_Laser_Switch"() -> (w1396:bool)
          n1519 = Not(x=w1396) -> (.not. x?=w1397:bool)
          n1520 = Select(t=w1434, s=w1437, f=w1435) -> (s? t:f=w1436:bool)
          n1521 = And(x=w1398, y=w1397) -> (x .and. y?=w1392:bool)
          n1522 = And(x=w1398, y=w1396) -> (x .and. y?=w1394:bool)
          n1523 = Or(x=w1395, y=w1394) -> (x .or. y?=w1385:bool)
          n1524 = Or(x=w1394, y=w1393) -> (x .or. y?=w1384:bool)
          n1525 = Or(x=w1391, y=w1392) -> (x .or. y?=w1387:bool)
          n1526 = Or(x=w1392, y=w1390) -> (x .or. y?=w1386:bool)
          n1527 = Or(x=w1400, y=w1401) -> (x .or. y?=w1389:bool)
          n1528 = Or(x=w1463, y=w1462) -> (x .or. y?=w1388:bool)
          n1529 = case shown="False" w1490 {
            tunnel: w1487 -> [w1511 w1519]
            tunnel: w1489 -> [_ w1516]
            tunnel: w1488 -> [_ w1515]
            tunnel: w1412 -> [_ w1514]
            tunnel: w1460 -> [_ w1513]
            tunnel: [w1511 w1518] -> w1486
            tunnel: [w1510 w1517] -> w1485
            tunnel: w1383 -> [w1510 w1512]
            frame False {
            }
            frame True {
              n1530 = call "myRIO_BRig_RT__Case_Exp__recordLick.vi"("intput_state__trialEnd"=w1513, "intput_state__trialStart"=w1514, "input_lick__R"=w1515, "input_lick__L"=w1516, "input_dataCurrent"=w1512, "input_dataLick"=w1519) -> ("output_dataCurrent"=w1517:u16[], "output_dataLick"=w1518:u16[][])  [unwired: 4 in]
            }
          }
          n1531 = Or(x=w1464, y=w1449) -> (x .or. y?=w1438:bool)
          n1532 = Or(x=w1448, y=w1465) -> (x .or. y?=w1461:bool)
          n1533 = Or(x=w1491, y="STOP_abort") -> (x .or. y?=w1493:bool)
          n1534 = Select(t=w1423, s=w1424, f=w1422) -> (s? t:f=w1411:u16)
          n1535 = Select(t=w1425, s=w1427, f=w1426) -> (s? t:f=w1410:u16)
          n1536 = Select(t=u16 0, s=w1430, f=w1429) -> (s? t:f=w1414:u16)
          n1537 = xnode "Read/Write Control"("FPGA VI Reference In"=w1440, "error in"=w1439, "A6_Act"=w1436, "audioTrigger_L"=w1438, "audioAmp_L"=w1474, "audioFreq_L_kHz"=w1447, "audioTrigger_R"=w1461, "audioAmp_R"=w1475, "audioFreq_R_kHz"=w1476, "CueLed_Event"=w1399, "A3_SL"=w1389, "A1_SR"=w1388, "LC_Event_l1"=w1387, "LC_Laser_l1"=w1386, "LC_Event_l2"=w1385, "LC_Laser_l2"=w1384) -> ("FPGA VI Reference Out"=w1484:refnum<k20>, "error out"=w1483:errorcluster, "AnaIn_0"=w1404:i16, "AnaIn_1"=w1413:i16)
          n1538 = call "myRIO_BRig_RT_dataAnalog_enterData__PortC.vi"("input_iState"=w1412, "input_AI0"=w1404, "input_iEvent"=w1414, "input_AI1"=w1413, "input_iTrial"=w1411, "input_iBlock"=w1410, "input_index"=w1415, "input_dataAnalog"=w1433) -> ("output_dataAnalog"=w1432:u16[][])  [unwired: 3 in]
          n1539 = call "myRIO_BRig_RT_TCP__v3__PortC.vi"("input_hTCP"=w1420, "input_AI1"=w1413, "input_AI0"=w1404, "input_I_connected_TCP"=w1416, "input_iBlock"=w1410, "input_spout"=w1409, "input_iTrial"=w1411, "input_error"=w1418, "input_countTrial"=w1406, "input_iState"=w1412) -> ("output_hTCP"=w1419:refnum<k5>, "output_countTrial"=w1405:u16, "output_error"=w1417:errorcluster)  [unwired: 3 in]
          n1540 = node-c288() -> ()  [unwired: 1 in, 1 out]
          n1541 = Increment(x=w1414) -> (x+1=w1421:u16)
          n1542 = Increment(x=w1415) -> (x+1=w1431:i32)
          "cState" <- w1412
        }
        n1543 = node-c288(w1333) -> ()  [unwired: 1 out]
        n1544 = flat-sequence {
          tunnel: w1329 -> [w1378]
          tunnel: w1328 -> [w1377]
          tunnel: [w1376] -> w1321
          tunnel: [w1375] -> w1320
          tunnel: [w1381] -> w1322
          tunnel: [w1382] -> w1327
          tunnel: w1321 -> [w1382]
          tunnel: w1320 -> [w1381]
          frame #0 {
            w1372 = u8 0
            w1373 = u16 0 ("AudioLeft_phase_inc")
            w1374 = FALSE
            n1545 = xnode "Read/Write Control"("FPGA VI Reference In"=w1378, "error in"=w1377, "Counts_Reset"=TRUE, "audioTrigger_L"=w1374, "audioFreq_L_kHz"=w1372, "audioAmp_L"=w1373, "audioTrigger_R"=w1374, "audioFreq_R_kHz"=w1372, "audioAmp_R"=w1373, "A3_SL"=w1374, "A1_SR"=w1374, "A6_Act"=w1374) -> ("FPGA VI Reference Out"=w1376:refnum<k20>, "error out"=w1375:errorcluster)
          }
          frame #1 {
            w1380 = FALSE ("START")
            n1546 = local write "START"(w1380) -> ()
            n1547 = local write "STOP_endTrial"(w1380) -> ()
            n1548 = local write "STOP_endBlock"(w1380) -> ()
          }
        }
        n1549 = stacked-sequence {
          tunnel: w1305 -> [w1352 _]
          tunnel: w1303 -> [w1353 _]
          tunnel: w1302 -> [_ w1358]
          tunnel: w1301 -> [_ w1357]
          tunnel: w1300 -> [_ w1356]
          tunnel: w1299 -> [w1346 _]
          tunnel: w1279 -> [w1343 _]
          tunnel: w1278 -> [w1342 _]
          frame #0 {
            n1550 = call "myRIO_BRig_RT_dataCurrent_idxDataLick.vi"() -> ("output_idxDataLick"=w1347:i32)  [unwired: 11 in]
            n1551 = Index Array(array=w1346, index=w1347) -> (element=w1349:u16)
            n1552 = Array Subset(array=w1343, length (row)=w1342) -> (w1344:u16[][])  [unwired: 3 in]
            n1553 = Increment(x=w1349) -> (x+1=w1350:u16)
            n1554 = call "myRIO_BRig_RT_comm_webdav_saveArrayToFile__1D_u16.vi"("Array"=w1353, "input_filename"="dataMTrig") -> ()  [unwired: 10 in]
            n1555 = To Long Integer(number=w1350) -> (32bit integer=w1348:i32)
            n1556 = Array Subset(array=w1352, length (row)=w1348) -> (w1351:u16[][])  [unwired: 3 in]
            n1557 = call "myRIO_BRig_RT_comm_webdav_saveArrayToFile__2D_u16.vi"("Array"=w1351, "input_filename"="dataLick") -> ()  [unwired: 10 in]
            n1558 = call "myRIO_BRig_RT_comm_webdav_saveArrayToFile__2D_u16.vi"("Array"=w1344, "input_filename"="dataAnalog") -> ()  [unwired: 10 in]
          }
          frame #1 {
            n1559 = case shown="True" w1358 {
              tunnel: w1357 -> [_ w1360]
              tunnel: w1356 -> [_ w1359]
              frame False {
              }
              frame True {
                n1560 = stacked-sequence {
                  tunnel: w1360 -> [w1362 w1369 w1371]
                  tunnel: w1359 -> [w1363 w1368 _]
                  frame #0 {
                    n1561 = call "myRIO_BRig_RT_comm_webdav_uploadFile__announce.vi"("input_addText"=TRUE, "input_fileName_prefix"=w1363, "intput_fileName"="curExp_end", "intput_hSession"=w1362) -> ("output_Isuccess"=w1361:bool)  [unwired: 6 in, 1 out]
                    n1562 = case shown="True" w1361 {
                      frame False {
                        n1563 = One Button Dialog(message="!!! Warning !!! Your data is located at C:\\BehaviorRig\\commTransfer") -> ()  [unwired: 1 in, 1 out]
                      }
                      frame True {
                        n1564 = Wait (ms)(milliseconds to wait=u32 20) -> ()  [unwired: 1 out]
                      }
                    }
                  }
                  frame #1 {
                    n1565 = call "myRIO_BRig_RT__endExp_sendData.vi"("input_fileName_prefix"=w1368, "input_hSession"=w1369) -> ()  [unwired: 8 in, 2 out]
                  }
                  frame #2 {
                    n1566 = local write "Connected To Host?"(FALSE ("Connected To Host?")) -> ()
                    n1567 = call <vilib>:"Close Session.vi"("session handle"=w1371) -> ()  [unwired: 14 in, 1 out]
                  }
                }
              }
            }
          }
        }
      }
    }
    n1568 = local read "STOP_abort"() -> (w44:bool)
  }
  n1569 = case shown="True" w5 {
    tunnel: w4 -> [_ w3701]
    tunnel: w3 -> [_ w3700]
    frame False {
    }
    frame True {
      n1570 = call "myRIO__TCP_disconnect_forWrite.vi"("input_error"=w3700, "input_hTCP"=w3701) -> ()  [unwired: 9 in, 1 out]
    }
  }
  n1571 = xnode "Read/Write Control"("FPGA VI Reference In"=w16, "error in"=w15, "FPGA_Stop"=TRUE) -> ("FPGA VI Reference Out"=w21:refnum<k20>, "error out"=w22:errorcluster)
  n1572 = xnode "Close FPGA VI Reference"("FPGA VI Reference In"=w21, "error in"=w22) -> ("error out"=w20:errorcluster)
  n1573 = call <vilib>:"Reset myRIO.vi"("error in (no error)"=w20) -> ()  [unwired: 10 in, 1 out]
